vi "RUNNER_Sievert_auto_RLC-CRZPhi.vi"() -> ()   [LabVIEW 2011]
uses:
  <vilib>/Utility/error.llb/DialogType.ctl
  <vilib>/DAQmx/write.llb/DAQmx Write (Digital Bool 1Line 1Point).vi
  <vilib>/DAQmx/create/channels.llb/DAQmx Create Channel (DO-Digital Output).vi
  <vilib>/DAQmx/miscellaneous.llb/DAQmx Fill In Error Info.vi
  <vilib>/Analysis/Matrix/Numeric/Conversions/Array To Matrix - RA.vi
  <vilib>/Analysis/Matrix/Numeric/Conversions/Matrix To Array - RM.vi
  <vilib>/Analysis/NI_AALPro.lvlib
  <vilib>/Analysis/Matrix/NI_Matrix.lvlib
  <vilib>/Analysis/NI_AALBase.lvlib
panel:
  out "S#1_auto":dbl
  out "S#01":dbl
  out "output array 3":u32[](array[numeric])
  out "PCh1 2":dbl[](array[numeric])
  out "tempo carga 2":dbl[](array[numeric])
  out "path RLC_mean 2":path
  out "MEASURE R [Ohm ]":dbl
  out "tempo carga":dbl[](array[numeric])
  out "PCh1":dbl[](array[numeric])
  out "output array 2":u32[](array[numeric])
  out "MEASURE C [F ]":dbl
  out "Automatico 2":dynamicdata(graph)
  out "termopar K 2":dbl format="%.3g"
  out "termopar K":string
  out "output NTC":dbl
  out "termopar K":dbl format="%.3g"
  out "path RLC_mean":path
  out "estagio 5":i32
  out "FIM":bool=TRUE
  out "limpo":i32
  in  "N fit":i32=5
  in  "ATM wait":u32
  in  "SET":i32
  in  "time subarray":dbl[](array[numeric])
  out "P cinetica mean 2":dbl format="%0.2f"
  out "T cinetica mean 3":dbl format="%0.2f"
  out "Time cinetica":dbl format="%0.2f"
  in  "T subarray 3":dbl[](array[numeric])
  in  "P T  index 2":i32
  in  "P subarray 2":dbl[](array[numeric])
  in  "Numeric":dbl=4.0
  in  "T subarray 2":dbl[](array[numeric])
  out "T cinetica mean 2":dbl format="%0.2f"
  out "P cinetica mean":dbl format="%0.2f"
  in  "P subarray":dbl[](array[numeric])
  in  "P T  index":i32
  out "T string":string
  out "P string":string
  out "path 2_cinetica":path
  out "Polynomial Coefficients 2":dbl[](array[numeric])
  out "Polynomial Coefficients":dbl[](array[numeric])
  in  "Count SET":i32=-1
  out "Set atual":i32
  out "mean pressure":dbl format="%.4p"
  out "Set number":i32
  in  "Tab Control":T1(tab)
  out "T":bool
  out "ZPf2":bool
  out "Pf2":bool
  out "Pit":bool
  out "ZPit":bool
  out "Camara":dbl(slide) scale=0.0..59.5 scale format="%#_3g"
  in  "Save manual":bool
  in  "Open Button":bool
  out "String 2":string
  in  "ATM":bool
  in  "Câmara":bool
  in  "Vácuo":bool
  in  "Entrada Gás":bool
  in  "Manual Ctrl":bool
  in  "stop":bool
  out "P-manual":dynamicdata(graph)
  in  "Clear":bool
  out "path":path
  in  "Nota":string
  in  "Sample name":string
  in  "File name":string
  out "Linear Model Graph":dbl[][](graph)
  out "Linear Model Graph 2":dbl[][](graph)
  in  "N to fit":i32=60
  out "N":i32
  out "Vácuo":bool
  out "Atm":bool
  out "Câmara":bool
  out "String_cinetica":string
  out "Vol Ref":dbl(slide) scale=0.0..60.0 scale format="%#_4f"
  out "Entrada gás":bool
  in  "Guardar\nCinetica":bool
  out "p fit":dbl format="%#_4g"
  out "T fit":dbl format="%#_4g"
  in  "Open Button 2":bool
  out "x >= y?":bool
  in  "seconds":dbl
  out "Elapsed Time (sec)":dbl format="%.1f"
  out "bar/N":dbl format="%#_4p"
  in  "correção\n NTC":dbl
  out "mean H2 sensor (V)":dbl format="%#_4p"
  in  "correçao\n termopar":dbl
  out "Boolean 3":bool
  out "String 3":string
  out "T 2":bool
  out "ZPit 2":bool
  out "Pit 2":bool
  out "Pf2 2":bool
  out "ZPf2 2":bool
  out "Camara 2":dbl(slide) scale=0.0..40.0 scale format="%#_3g"
  out "Vácuo 2":bool
  out "Atm 2":bool
  out "Câmara 2":bool
  out "Vol Ref 3":dbl(slide) scale=0.0..100.0 scale format="%#_4f"
  out "Entrada gás 2":bool
  in  "Auto Ctrl":bool
  in  "Play Button":bool
  out "time stamp":timestamp format="%<%.2X>T"
  out "Time (sec)":dbl format="%.1f"
  in  "clear":bool
  out "Automatico":dynamicdata(graph)
  out "Linear P":T2(graph)
  out "Linear T":T2(graph)
  out "Contador":i32
  in  "STOP (bar/s)":dbl format="%#_5p"
  out "P (bar/s)":dbl format="%#_5p"
  out "bar/s":dbl format="%#_4p"
  out "P fit":dbl format="%#_4g"
  out "T fit":dbl format="%#_4g"
  out "x = y?":bool
  out "teste slope":i32
  in  "Set P auto":dbl
  in  "Step P":dbl=2.0
  in  "P_max":dbl=2.0
  in  "P_max camara":dbl=2.0
  out "Carga":bool=TRUE
  out "Descarga":bool
  out "String":string
  in  "P_min descarga":dbl
  in  "Boolean":bool
  in  "Array":dbl[](array[numeric])
  out "Boolean 2":bool
  out "Desc SET":i32
  in  "ZPf2 time":dbl=24.0
  in  "Ciclos":dbl
  out "Efetuados":dbl
  in  "patamar milliseconds to wait":u32=500
  in  "N fit patamar":i32=100
  in  "Step ZPit":dbl
  out "Read ZPit":bool
  in  "Estagio auto":i32
  out "mean H2 sensor":dbl format="%#_4p"
  in  "Ntest":i32=5
  in  "N fit 2":i32=100
  in  "Read val open":bool
  out "mean 18":dbl format="%.3p"
  out "mean 17":dbl format="%.3p"
  in  "C50L":bool
  in  "C50N":bool
  in  "C100L":bool
  in  "C100N":bool
  in  "C1KL":bool
  in  "C1KN":bool
  in  "C10KL":bool
  in  "C10KN":bool
  out "String 4":string
  in  "Combo Box":string(combo)
  in  "Refresh Button":bool
  in  "Close RLC 2":bool
  in  "RLC on/off":bool
  out "mean 16":dbl format="%.3p"
  out "mean 15":dbl format="%.3p"
  out "mean 14":dbl format="%.3p"
  out "mean 13":dbl format="%.3p"
  out "mean 12":dbl format="%.3p"
  out "mean 11":dbl format="%.3p"
  out "mean 10":dbl format="%.3p"
  out "mean 9":dbl format="%.3p"
  out "mean 8":dbl format="%.3p"
  out "mean 7":dbl format="%.3p"
  out "mean 6":dbl format="%.3p"
  out "mean 5":dbl format="%.3p"
  out "mean 4":dbl format="%.3p"
  out "mean 3":dbl format="%.3p"
  out "mean 2":dbl format="%.3p"
  out "mean":dbl format="%.3p"
  out "SET 2":dbl
  out "C-50-L":bool
  out "MEASURE B":dbl
  out "MEASURE A":dbl
  out "C-50-N":bool
  out "MEASURE B 2":dbl
  out "MEASURE A 2":dbl
  out "C-100-L":bool
  out "MEASURE B 3":dbl
  out "MEASURE A 3":dbl
  out "C-100-N":bool
  out "MEASURE B 4":dbl
  out "MEASURE A 4":dbl
  out "C-1K-L":bool
  out "MEASURE B 5":dbl
  out "MEASURE A 5":dbl
  out "C-1K-N":bool
  out "MEASURE B 6":dbl
  out "MEASURE A 6":dbl
  out "C-10K-L":bool
  out "MEASURE B 7":dbl
  out "MEASURE A 7":dbl
  out "C-10K-N":bool
  out "MEASURE B 8":dbl
  out "MEASURE A 8":dbl
  out "Z-50-L":bool
  out "MEASURE B 9":dbl
  out "MEASURE A 9":dbl
  out "Z-50-N":bool
  out "MEASURE B 10":dbl
  out "MEASURE A 10":dbl
  out "Z-100-L":bool
  out "MEASURE B 11":dbl
  out "MEASURE A 11":dbl
  out "Z-100-N":bool
  out "MEASURE B 12":dbl
  out "MEASURE A 12":dbl
  out "Z-1K-L":bool
  out "MEASURE B 13":dbl
  out "MEASURE A 13":dbl
  out "Z-1K-N":bool
  out "MEASURE B 14":dbl
  out "MEASURE A 14":dbl
  out "Z-10K-L":bool
  out "MEASURE B 15":dbl
  out "MEASURE A 15":dbl
  out "Z-10K-N":bool
  out "MEASURE B 16":dbl
  out "MEASURE A 16":dbl
  out "RLC300 - digimess":string
  in  "Time RLC":u32=5000
  in  "Ligar RLC":bool
  out "path RLC_completo":path
  out "Waveform Chart P 2":dbl[][](graph)
  out "Waveform Chart":dynamicdata(graph)
  in  "graph RLC":bool
  in  "Refresh Button 2":bool
  in  "Z50L":bool
  in  "Z50N":bool
  in  "Z100L":bool
  in  "Z100N":bool
  in  "Z1KL":bool
  in  "Z1KN":bool
  in  "Z10KL":bool
  in  "Z10KN":bool
  out "T(º) FIT":dbl
  out "Waveform Chart 2":dynamicdata(graph)
  out "XY Graph 2":cluster{"Value":dbl[], "Value":dbl[]}[](graph)
  in  "t-sivert01(s)":dbl
  out "dP/dt (bar/s)":dbl format="%#_5p"
  in  "Save - Sievert 01":bool
  in  "File name 2":string
  in  "Nota 01":string
  in  "Sample name 2":string
  in  "Save S#1":bool
  out "path 2":path
  out "Boolean 4":bool
  out "P(bar) FIT":dbl
  in  "ON/OFF":bool
  in  "Refresh Button 3":bool
  # "P vol ref"
  # "P Câmara"
  # "P vol ref"
  # "P Câmara"
  # "C ( F )"
  # "R ( Ohm )"
  # "Z ( Ohm )"
  # "Phase ( deg)"
types:
  T1 = enum32{"Manual", "Automatico", "RLC - CDH2", "Sievert 01"}
  T2 = cluster{"Real 2D Array":dbl[], "Best Linear Fit":dbl[]}[]
  T3 = enum16{"open", "replace", "create", "open or create", "replace or create", "replace or create with confirmation"}
  T4 = typedef "DialogType.ctl" = u16
  T5 = cluster{"Value":dbl[], "Best Polynomial Fit":dbl[]}
  T6 = cluster{"Value":dbl[], "Best Polynomial Fit":dbl[]}[]
  T7 = typedef "NI_Matrix.lvlib/RealMatrix.ctl" = dbl[][]
  T8 = cluster{"Real 2D Array":dbl[], "Real 2D Array":dbl[]}
  T9 = cluster{"Real 2D Array":dbl[], "Best Linear Fit":dbl[]}
  T10 = cluster{"Real 2D Array":dbl[], "Best Polynomial Fit":dbl[]}
  T11 = cluster{"Real 2D Array":dbl[], "Best Polynomial Fit":dbl[]}[]
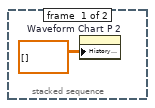
[diagram p7: hidden frame]
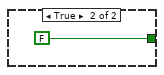
[diagram p12: hidden frame]
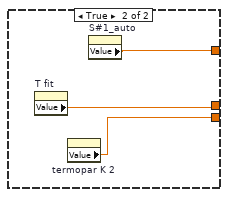
[diagram p15: hidden frame]
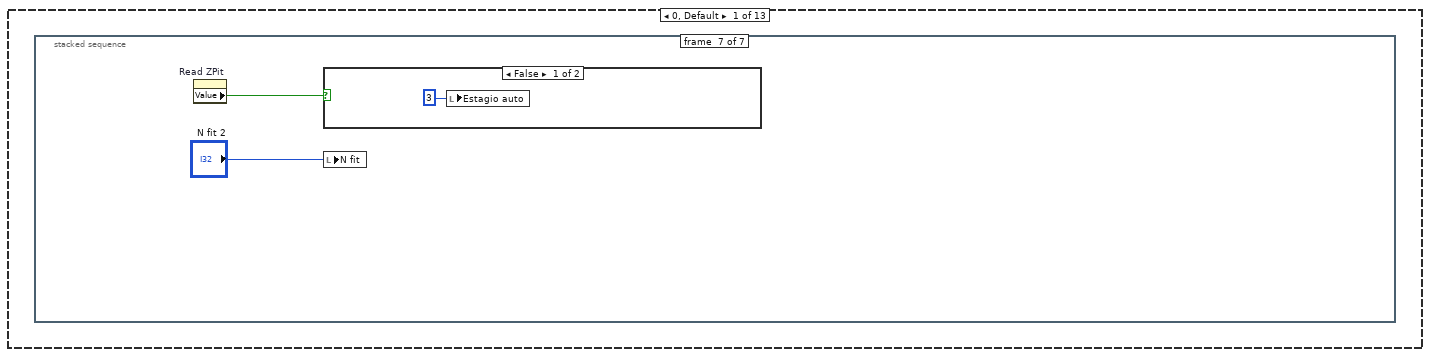
[diagram p20: hidden frame]
diagram:
  w2 = TRUE ("C1KN")
  (unwired) dbl[] [0.5, 1.0, 2.0, 3.0, 4.0, 5.0, 6.0, 7.0, 8.0, 9.0, 10.0, 11.0, 12.0, 13.0, 14.0, 15.0, 16.0, 17.0, 18.0, 19.0, 20.0, 30.0, 40.0, 50.0, 60.0, 70.0] ("Array")
  n1 = local write "N to fit"(5 ("Numeric")) -> ()
  n2 = local write "Step ZPit"(5.0 ("Step ZPit")) -> ()
  n3 = local write "Time RLC"(u32 5 ("Time RLC")) -> ()
  n4 = local write "Ciclos"(0.0 ("Ciclos")) -> ()
  n5 = local write "Desc SET"(0 ("Desc SET")) -> ()
  n6 = local write "Efetuados"(0.0 ("Efetuados")) -> ()
  n7 = local write "estagio 5"(0 ("estagio 5")) -> ()
  n8 = local write "teste slope"(0 ("teste slope")) -> ()
  n9 = local write "SET"(0 ("SET auto")) -> ()
  n10 = local write "limpo"(0 ("limpo")) -> ()
  n11 = local write "N fit"(5 ("N fit")) -> ()
  n12 = local write "ATM wait"(u32 4 ("ATM wait")) -> ()
  n13 = local write "Estagio auto"(0 ("Estagio auto")) -> ()
  n14 = local write "P T  index"(0 ("index")) -> ()
  n15 = local write "seconds"(2.0 ("seconds")) -> ()
  n16 = local write "C1KN"(w2) -> ()
  n17 = local write "Z1KN"(w2) -> ()
  n18 = local write "Read ZPit"(TRUE ("Read ZPit")) -> ()
  n19 = local write "Descarga"(FALSE ("Descarga")) -> ()
  n20 = local write "Carga"(TRUE ("Carga")) -> ()
  n21 = local write "FIM"(FALSE ("FIM")) -> ()
  n22 = local write "t-sivert01(s)"(10.0 ("t-sivert01(s)")) -> ()
  n23 = local write "P_max"(50.0 ("P_max")) -> ()
  n24 = local write "P_max camara"(25.0 ("P_max camara")) -> ()
  n25 = local write "correção\n NTC"(0.5 ("correção NTC")) -> ()
  n26 = local write "Set P auto"(0.5 ("Set P auto")) -> ()
  n27 = local write "P_min descarga"(0.025 ("P_min descarga")) -> ()
  n28 = local write "Array"(dbl[] [0.5, 1.0, 2.0, 3.0, 4.0, 4.0, 4.0, 4.0, 4.0, 4.0, 4.0, 5.0, 5.0, 5.0, 7.0, 10.0, 15.0, 20.0, 25.0, 25.0, 25.0, 30.0, 40.0, 50.0, 60.0, 70.0] ("Array")) -> ()
  n29 = local write "P subarray"(dbl[] [0.0, 1.0] ("subarray")) -> ()
  n30 = local write "T subarray 2"(dbl[] [0.0, 1.0] ("subarray")) -> ()
  n31 = local write "Combo Box"("rlc_read_cCN.py" ("Combo Box")) -> ()
  n32 = while {
    tunnel: path "C:/H2_Painel/painel_auto/RLC_CDH" ("Path") -> [w40]
    stop <- w52 stop-if-true
    n33 = property on="FIM" class="Bool (strict)"() -> ("Value"=w50:bool)  [unwired: 2 in, 2 out]
    n34 = property on="path" class="Path"() -> ("Value"=w47:path)  [unwired: 2 in, 2 out]
    n35 = case shown="True" "Ligar RLC" {
      tunnel: w40 -> [_ w231]
      frame False {
      }
      frame True {
        n36 = call "RLC_open.vi"("Path"=w231) -> ("String 2"=w232:string)  [unwired: 9 in, 1 out]
        n37 = local write "RLC300 - digimess"(w232) -> ()
      }
    }
    n38 = case shown="True" "RLC on/off" {
      tunnel: w40 -> [_ _]
      frame False {
      }
      frame True {
        n39 = call "RLC READ DINAMICO.vi"("Boolean"="graph RLC") -> ("MEASURE R [Ohm ]"=w66:dbl, "MEASURE C [F ]"=w65:dbl)  [unwired: 9 in]
        "MEASURE C [F ]" <- w65
        "MEASURE R [Ohm ]" <- w66
        n40 = Merge Signals(w65, w66) -> (→"Waveform Chart":dynamicdata)
        "String 4" <- "Combo Box"
      }
    }
    n41 = case shown="True" "Manual Ctrl" {
      tunnel: w40 -> [_ w1859]
      tunnel: "RLC on/off" -> [_ w1858]
      tunnel: [FALSE w1861] -> w42
      frame False {
      }
      frame True {
        w1873 = 0 ("polynomial order")
        n42 = case shown="True" "Save manual" {
          selector: "Save manual" -> [_ w2475]
          frame False {
          }
          frame True {
            n43 = feedback #1() -> (w2471:dbl)  [unwired: 1 in]
            n44 = Equal To 0?(x=w2471) -> (x = 0?=w2477:bool)
            n45 = stacked-sequence {
              tunnel: w2477 -> [_ w2493 _]
              tunnel: [_ w2492 _] -> w2473
              frame #0 {
                w2486 = i16 3 ("precision (6)")
                n46 = property on="T fit" class="DigNum (strict)"() -> ("Value"=w2488:dbl)  [unwired: 2 in, 2 out]
                n47 = property on="p fit" class="DigNum (strict)"() -> ("Value"=w2489:dbl)  [unwired: 2 in, 2 out]
                n48 = property on="termopar K" class="DigNum (strict)"() -> ("Value"=w2487:dbl)  [unwired: 2 in, 2 out]
                n49 = Number To Fractional String(number=w2488, precision (6)=w2486) -> (F-format string=→"T string":string)  [unwired: 2 in]
                n50 = Number To Fractional String(number=w2489, precision (6)=w2486) -> (F-format string=→"P string":string)  [unwired: 2 in]
                n51 = Number To Fractional String(number=w2487, precision (6)=w2486) -> (F-format string=→"termopar K":string)  [unwired: 2 in]
              }
              frame #1 {
                n52 = case shown="True" w2493 {
                  tunnel: [TRUE ("y") FALSE ("y")] -> w2492
                  frame False {
                    n53 = property on="path" class="Path"() -> ("Value"=w2497:path)  [unwired: 2 in, 2 out]
                    n54 = property on="P string" class="Str"() -> ("Value"=w2496:string)  [unwired: 2 in, 2 out]
                    n55 = Concatenate Strings(w2496, "\t") -> (w2494:string)
                    n56 = Open/Create/Replace File(file path (use dialog)=w2497, operation (0:open)=T3."open") -> (refnum out=w2501:refnum<file>, error out=w2500:errorcluster)  [unwired: 2 in, 3 out]
                    n57 = Set File Position(refnum=w2501, from (0:start)=enum16{"start", "end", "current"}."end", error in=w2500) -> (refnum out=w2503:refnum<file>, error out=w2504:errorcluster)  [unwired: 1 in]
                    n58 = Write to Text File(file (use dialog)=w2503, text=w2494, error in=w2504) -> (refnum out=w2499:refnum<file>, error out=w2498:errorcluster)  [unwired: 2 out]
                    n59 = Close File(refnum=w2499, error in=w2498) -> (error out=w2506:errorcluster)  [unwired: 1 out]
                    n60 = call <vilib>:"Simple Error Handler.vi"("error in (no error)"=w2506) -> ()  [unwired: 1 in, 8 out]
                  }
                  frame True {
                    w2509 = "\t"
                    n61 = property on="path" class="Path"() -> ("Value"=w2516:path)  [unwired: 2 in, 2 out]
                    n62 = property on="Count SET" class="DigNum (strict)"() -> ("Value"=w2512:i32)  [unwired: 2 in, 2 out]
                    n63 = Open/Create/Replace File(file path (use dialog)=w2516, operation (0:open)=T3."open") -> (refnum out=w2515:refnum<file>, error out=w2514:errorcluster)  [unwired: 2 in, 3 out]
                    n64 = Increment(x=w2512) -> (x+1=w2513:i32)
                    "Set atual" <- w2513
                    n65 = Set File Position(refnum=w2515, from (0:start)=enum16{"start", "end", "current"}."end", error in=w2514) -> (refnum out=w2524:refnum<file>, error out=w2525:errorcluster)  [unwired: 1 in]
                    n66 = Number To Decimal String(number=w2513) -> (decimal integer string=w2517:string)  [unwired: 1 in]
                    n67 = property on="termopar K" class="Str"() -> ("Value"=w2508:string)  [unwired: 2 in, 2 out]
                    n68 = property on="T string" class="Str"() -> ("Value"=w2510:string)  [unwired: 2 in, 2 out]
                    n69 = Concatenate Strings(w2510, w2509, w2508, "\r\n", w2517, w2509) -> (w2519:string)
                    n70 = Write to Text File(file (use dialog)=w2524, text=w2519, error in=w2525) -> (refnum out=w2522:refnum<file>, error out=w2521:errorcluster)  [unwired: 2 out]
                    n71 = Close File(refnum=w2522, error in=w2521) -> (error out=w2527:errorcluster)  [unwired: 1 out]
                    n72 = call <vilib>:"Simple Error Handler.vi"("error in (no error)"=w2527) -> ()  [unwired: 1 in, 8 out]
                    "T" <- TRUE ("T")
                  }
                }
              }
              frame #2 {
                n73 = property on="path" class="Path"() -> ("Value"=w2529:path)  [unwired: 2 in, 2 out]
                n74 = property on="Set atual" class="DigNum (strict)"() -> ("Value"=w2528:i32)  [unwired: 2 in, 2 out]
                n75 = local write "Count SET"(w2528) -> ()
                n76 = Read from Text File(file (use dialog)=w2529, count=-1 ("Count  3")) -> (refnum out=w2531:refnum<file>, text=w2530:string, error out=w2532:errorcluster)  [unwired: 2 in, 1 out]
                n77 = property on="String 2" class="Str"("Value"=w2530) -> ()  [unwired: 2 in, 2 out]
                n78 = Close File(refnum=w2531, error in=w2532) -> (error out=w2534:errorcluster)  [unwired: 1 out]
                n79 = call <vilib>:"Simple Error Handler.vi"("error in (no error)"=w2534) -> ()  [unwired: 1 in, 8 out]
              }
            }
            n80 = Implies(1:w2473, 2:w2475) -> (0:w2474:bool)
            n81 = Select(t=w2471, s=w2474, f=5.0 ("t")) -> (s? t:f=w2472:dbl)
            n82 = case shown="1" w2472 {
              frame 0, Default {
              }
              frame 1 {
                "ZPf2" <- TRUE ("ZPf2")
              }
              frame 2 {
                "Pf2" <- TRUE ("Pf2")
              }
              frame 3 {
                "Pit" <- TRUE ("Pit")
              }
              frame 4 {
                n83 = local write "T"(FALSE ("T")) -> ()
                "ZPit" <- TRUE ("ZPit")
              }
              frame 5 {
                w2484 = FALSE
                n84 = local write "Pit"(w2484) -> ()
                n85 = local write "ZPf2"(w2484) -> ()
                n86 = local write "ZPit"(w2484) -> ()
                n87 = local write "Pf2"(w2484) -> ()
              }
            }
            n88 = Decrement(x=w2472) -> (x-1=w2478:dbl)
            n89 = feedback-in #1(w2478) -> ()
          }
        }
        n90 = case shown="True" w1858 {
          tunnel: [FALSE ("Save manual") w2470] -> w1860
          tunnel: "Save manual" -> [_ w2470]
          frame False {
          }
          frame True {
          }
        }
        n91 = case shown="True" w1858 {
          tunnel: [FALSE w1878] -> w1861
          tunnel: w1860 -> [_ w1877]
          tunnel: w1859 -> [_ w1876]
          frame False {
          }
          frame True {
            n92 = flat-sequence {
              tunnel: w1876 -> [w1899]
              tunnel: w1877 -> [w1900]
              tunnel: [w1900] -> w1897
              tunnel: [w1899] -> w1896
              tunnel: [w1907] -> w1895
              tunnel: [w1908] -> w1894
              tunnel: [w1909] -> w1893
              tunnel: [w1910] -> w1892
              tunnel: [w1911] -> w1891
              tunnel: [w1912] -> w1890
              tunnel: [w1913] -> w1889
              tunnel: [w1915] -> w1888
              tunnel: [w1916] -> w1887
              tunnel: [w1917] -> w1886
              tunnel: [w1918] -> w1885
              tunnel: [w1919] -> w1884
              tunnel: [w1914] -> w1883
              tunnel: [w1906] -> w1882
              tunnel: [w1905] -> w1881
              tunnel: [w1904] -> w1880
              tunnel: [w1903] -> w1879
              tunnel: w1897 -> [w1902]
              tunnel: w1896 -> [w1901]
              tunnel: w1895 -> [w2417]
              tunnel: w1894 -> [w2416]
              tunnel: w1893 -> [w2415]
              tunnel: w1892 -> [w2414]
              tunnel: w1891 -> [w2413]
              tunnel: w1890 -> [w2412]
              tunnel: w1889 -> [w2411]
              tunnel: w1888 -> [w2410]
              tunnel: w1887 -> [w2409]
              tunnel: w1886 -> [w2408]
              tunnel: w1885 -> [w2407]
              tunnel: w1884 -> [w2406]
              tunnel: w1883 -> [w2405]
              tunnel: w1882 -> [w2418]
              tunnel: w1881 -> [w2419]
              tunnel: w1880 -> [w2420]
              tunnel: [w2403] -> w1878
              tunnel: w1879 -> [w2403]
              tunnel: [TRUE] -> w1875
              frame #0 {
                n93 = local write "graph RLC"(FALSE) -> ()
              }
              frame #1 {
                n94 = case shown="True" w1902 {
                  tunnel: [_ w1954] -> w1903
                  tunnel: w1901 -> [_ w1936]
                  tunnel: [_ w1935] -> w1904
                  tunnel: [_ w1934] -> w1905
                  tunnel: [_ w1933] -> w1906
                  tunnel: [_ w1932] -> w1907
                  tunnel: [_ w1931] -> w1908
                  tunnel: [_ w1930] -> w1909
                  tunnel: [_ w1929] -> w1910
                  tunnel: [_ w1928] -> w1911
                  tunnel: [_ w1927] -> w1912
                  tunnel: [_ w1926] -> w1913
                  tunnel: [_ w1925] -> w1914
                  tunnel: [_ w1924] -> w1915
                  tunnel: [_ w1923] -> w1916
                  tunnel: [_ w1922] -> w1917
                  tunnel: [_ w1921] -> w1918
                  tunnel: [_ w1920] -> w1919
                  frame False {
                  }
                  frame True {
                    n95 = for {
                      N: 5 -> [_]
                      tunnel: TRUE -> [w1977]
                      tunnel: FALSE -> [w1976]
                      tunnel: [w1975] -> w1954
                      tunnel: [w1974] -> w1952 mode=indexing
                      tunnel: [w1973] -> w1951 mode=indexing
                      tunnel: [w1972] -> w1950 mode=indexing
                      tunnel: [w1971] -> w1949 mode=indexing
                      tunnel: [w1970] -> w1948 mode=indexing
                      tunnel: [w1969] -> w1947 mode=indexing
                      tunnel: [w1968] -> w1946 mode=indexing
                      tunnel: [w1967] -> w1945 mode=indexing
                      tunnel: [w1966] -> w1944 mode=indexing
                      tunnel: [w1965] -> w1943 mode=indexing
                      tunnel: [w1964] -> w1942 mode=indexing
                      tunnel: [w1963] -> w1941 mode=indexing
                      tunnel: [w1962] -> w1940 mode=indexing
                      tunnel: [w1961] -> w1939 mode=indexing
                      tunnel: [w1960] -> w1938 mode=indexing
                      tunnel: [w1959] -> w1937 mode=indexing
                      tunnel: w1936 -> [w1958]
                      n96 = property on="path RLC_completo" class="Path"() -> ("Value"=w1957:path)  [unwired: 2 in, 2 out]
                      n97 = stacked-sequence {
                        tunnel: w1977 -> [_ w2002 w2027 w2052 w2077 w2102 w2127 w2152 w2175 w2200 w2227 w2250 w2277 w2302 w2327 w2350 w2377 _]
                        tunnel: w1976 -> [w1978 _ _ _ _ _ _ _ _ _ _ _ _ _ _ _ _ w2401]
                        tunnel: [_ _ _ _ _ _ _ _ _ _ _ _ _ _ _ _ _ TRUE] -> w1975
                        tunnel: [_ w2001 _ _ _ _ _ _ _ _ _ _ _ _ _ _ _ _] -> w1974
                        tunnel: [_ _ w2026 _ _ _ _ _ _ _ _ _ _ _ _ _ _ _] -> w1973
                        tunnel: [_ _ _ w2051 _ _ _ _ _ _ _ _ _ _ _ _ _ _] -> w1972
                        tunnel: [_ _ _ _ w2076 _ _ _ _ _ _ _ _ _ _ _ _ _] -> w1971
                        tunnel: [_ _ _ _ _ w2101 _ _ _ _ _ _ _ _ _ _ _ _] -> w1970
                        tunnel: [_ _ _ _ _ _ w2126 _ _ _ _ _ _ _ _ _ _ _] -> w1969
                        tunnel: [_ _ _ _ _ _ _ w2151 _ _ _ _ _ _ _ _ _ _] -> w1968
                        tunnel: [_ _ _ _ _ _ _ _ w2177 _ _ _ _ _ _ _ _ _] -> w1967
                        tunnel: [_ _ _ _ _ _ _ _ _ w2202 _ _ _ _ _ _ _ _] -> w1966
                        tunnel: [_ _ _ _ _ _ _ _ _ _ w2226 _ _ _ _ _ _ _] -> w1965
                        tunnel: [_ _ _ _ _ _ _ _ _ _ _ w2252 _ _ _ _ _ _] -> w1964
                        tunnel: [_ _ _ _ _ _ _ _ _ _ _ _ w2276 _ _ _ _ _] -> w1963
                        tunnel: [_ _ _ _ _ _ _ _ _ _ _ _ _ w2301 _ _ _ _] -> w1962
                        tunnel: [_ _ _ _ _ _ _ _ _ _ _ _ _ _ w2326 _ _ _] -> w1961
                        tunnel: [_ _ _ _ _ _ _ _ _ _ _ _ _ _ _ w2352 _ _] -> w1960
                        tunnel: [_ _ _ _ _ _ _ _ _ _ _ _ _ _ _ _ w2376 _] -> w1959
                        tunnel: w1958 -> [_ w2004 w2030 w2054 w2079 w2104 w2129 w2154 w2179 w2204 w2229 w2254 w2279 w2304 w2329 w2354 w2379 _]
                        tunnel: w1957 -> [w1980 w2003 w2029 w2053 w2078 w2103 w2128 w2153 w2178 w2203 w2228 w2253 w2278 w2303 w2328 w2353 w2378 _]
                        frame #0 {
                          w1981 = "\t"
                          n98 = local write "C-50-L"(w1978) -> ()
                          n99 = local write "C-50-N"(w1978) -> ()
                          n100 = local write "Z-50-L"(w1978) -> ()
                          n101 = local write "Z-50-N"(w1978) -> ()
                          n102 = local write "C-1K-L"(w1978) -> ()
                          n103 = local write "C-1K-N"(w1978) -> ()
                          n104 = local write "Z-1K-N"(w1978) -> ()
                          n105 = local write "Z-1K-L"(w1978) -> ()
                          n106 = local write "Z-100-L"(w1978) -> ()
                          n107 = local write "C-10K-L"(w1978) -> ()
                          n108 = local write "C-100-N"(w1978) -> ()
                          n109 = local write "C-10K-N"(w1978) -> ()
                          n110 = local write "Z-10K-N"(w1978) -> ()
                          n111 = local write "Z-10K-L"(w1978) -> ()
                          n112 = local write "Z-100-N"(w1978) -> ()
                          n113 = local write "C-100-L"(w1978) -> ()
                          n114 = Open/Create/Replace File(file path (use dialog)=w1980, operation (0:open)=T3."open") -> (refnum out=w1994:refnum<file>, error out=w1993:errorcluster)  [unwired: 2 in, 3 out]
                          n115 = Get Date/Time String(date format (0)=enum16{"short", "long", "abbreviated"}."short", want seconds? (F)=TRUE) -> (date string=w1986:string, time string=w1985:string)  [unwired: 1 in]
                          n116 = feedback #2() -> (w1979:dbl)  [unwired: 1 in]
                          n117 = local write "SET 2"(w1979) -> ()
                          n118 = Set File Position(refnum=w1994, from (0:start)=enum16{"start", "end", "current"}."end", error in=w1993) -> (refnum out=w1996:refnum<file>, error out=w1997:errorcluster)  [unwired: 1 in]
                          n119 = Number To Fractional String(number=w1979, precision (6)=i16 2) -> (F-format string=w1984:string)  [unwired: 2 in]
                          n120 = Add(x=w1979, y=0.2) -> (x+y=w1990:dbl)
                          n121 = feedback-in #2(w1990) -> ()
                          n122 = Concatenate Strings(w1984, w1981, w1986, w1981, w1985, w1981) -> (w1983:string)
                          n123 = Write to Text File(file (use dialog)=w1996, text=w1983, error in=w1997) -> (refnum out=w1992:refnum<file>, error out=w1991:errorcluster)  [unwired: 1 in, 1 out]
                          n124 = Close File(refnum=w1992, error in=w1991) -> (error out=w1999:errorcluster)  [unwired: 1 out]
                          n125 = call <vilib>:"Simple Error Handler.vi"("error in (no error)"=w1999) -> ()  [unwired: 1 in, 8 out]
                        }
                        frame #1 {
                          w2005 = "\t"
                          w2022 = i16 4 ("width (-)")
                          n126 = local write "C-50-L"(w2002) -> ()
                          n127 = Wait (ms)(milliseconds to wait=u32 5000) -> ()  [unwired: 1 out]
                          n128 = Open/Create/Replace File(file path (use dialog)=w2003, operation (0:open)=T3."open") -> (refnum out=w2014:refnum<file>, error out=w2013:errorcluster)  [unwired: 2 in, 3 out]
                          n129 = Set File Position(refnum=w2014, from (0:start)=enum16{"start", "end", "current"}."end", error in=w2013) -> (refnum out=w2016:refnum<file>, error out=w2017:errorcluster)  [unwired: 1 in]
                          n130 = call "RLC_read.vi"("Path"=w2004, "String"="cmd /c rlc_read_cAL.py") -> ("MEASURE A"=w2001:dbl, "MEASURE V [V]"=w2021:dbl, "MEASURE B"=w2000:dbl, "MEASURE I [A]"=w2020:dbl)  [unwired: 2 out]
                          n131 = Number To Engineering String(2:w2022, 4:w2020) -> (0:w2006:string)  [unwired: 2 in]
                          n132 = local write "MEASURE A"(w2001) -> ()
                          n133 = local write "MEASURE B"(w2000) -> ()
                          n134 = Number To Engineering String(2:w2022, 4:w2021) -> (0:w2007:string)  [unwired: 2 in]
                          n135 = Number To Engineering String(2:w2022, 4:w2001) -> (0:w2009:string)  [unwired: 2 in]
                          n136 = Number To Engineering String(2:w2022, 4:w2000) -> (0:w2008:string)  [unwired: 2 in]
                          n137 = Concatenate Strings(w2009, w2005, w2008, w2005, w2007, w2005, w2006, w2005) -> (w2010:string)
                          n138 = Write to Text File(file (use dialog)=w2016, text=w2010, error in=w2017) -> (refnum out=w2012:refnum<file>, error out=w2011:errorcluster)  [unwired: 1 in, 1 out]
                          n139 = Close File(refnum=w2012, error in=w2011) -> (error out=w2019:errorcluster)  [unwired: 1 out]
                          n140 = call <vilib>:"Simple Error Handler.vi"("error in (no error)"=w2019) -> ()  [unwired: 1 in, 8 out]
                        }
                        frame #2 {
                          w2033 = "\t"
                          w2047 = i16 4 ("width (-)")
                          n141 = local write "C-50-N"(w2027) -> ()
                          n142 = Wait (ms)(milliseconds to wait=u32 5000) -> ()  [unwired: 1 out]
                          n143 = Open/Create/Replace File(file path (use dialog)=w2029, operation (0:open)=T3."open") -> (refnum out=w2041:refnum<file>, error out=w2040:errorcluster)  [unwired: 2 in, 3 out]
                          n144 = Set File Position(refnum=w2041, from (0:start)=enum16{"start", "end", "current"}."end", error in=w2040) -> (refnum out=w2043:refnum<file>, error out=w2044:errorcluster)  [unwired: 1 in]
                          n145 = call "RLC_read.vi"("Path"=w2030, "String"="cmd /c rlc_read_cAN.py") -> ("MEASURE A"=w2026:dbl, "MEASURE V [V]"=w2032:dbl, "MEASURE B"=w2025:dbl, "MEASURE I [A]"=w2031:dbl)  [unwired: 2 out]
                          n146 = Number To Engineering String(2:w2047, 4:w2031) -> (0:w2034:string)  [unwired: 2 in]
                          n147 = local write "MEASURE A 2"(w2026) -> ()
                          n148 = local write "MEASURE B 2"(w2025) -> ()
                          n149 = Number To Engineering String(2:w2047, 4:w2032) -> (0:w2035:string)  [unwired: 2 in]
                          n150 = Number To Engineering String(2:w2047, 4:w2026) -> (0:w2037:string)  [unwired: 2 in]
                          n151 = Number To Engineering String(2:w2047, 4:w2025) -> (0:w2036:string)  [unwired: 2 in]
                          n152 = Concatenate Strings(w2037, w2033, w2036, w2033, w2035, w2033, w2034, w2033) -> (w2028:string)
                          n153 = Write to Text File(file (use dialog)=w2043, text=w2028, error in=w2044) -> (refnum out=w2039:refnum<file>, error out=w2038:errorcluster)  [unwired: 1 in, 1 out]
                          n154 = Close File(refnum=w2039, error in=w2038) -> (error out=w2046:errorcluster)  [unwired: 1 out]
                          n155 = call <vilib>:"Simple Error Handler.vi"("error in (no error)"=w2046) -> ()  [unwired: 1 in, 8 out]
                        }
                        frame #3 {
                          w2057 = "\t"
                          w2072 = i16 4 ("width (-)")
                          n156 = Wait (ms)(milliseconds to wait=u32 5000) -> ()  [unwired: 1 out]
                          n157 = local write "C-100-L"(w2052) -> ()
                          n158 = Open/Create/Replace File(file path (use dialog)=w2053, operation (0:open)=T3."open") -> (refnum out=w2066:refnum<file>, error out=w2065:errorcluster)  [unwired: 2 in, 3 out]
                          n159 = Set File Position(refnum=w2066, from (0:start)=enum16{"start", "end", "current"}."end", error in=w2065) -> (refnum out=w2068:refnum<file>, error out=w2069:errorcluster)  [unwired: 1 in]
                          n160 = call "RLC_read.vi"("Path"=w2054, "String"="cmd /c rlc_read_cBL.py") -> ("MEASURE A"=w2051:dbl, "MEASURE V [V]"=w2056:dbl, "MEASURE B"=w2050:dbl, "MEASURE I [A]"=w2055:dbl)  [unwired: 2 out]
                          n161 = Number To Engineering String(2:w2072, 4:w2055) -> (0:w2058:string)  [unwired: 2 in]
                          n162 = local write "MEASURE A 3"(w2051) -> ()
                          n163 = local write "MEASURE B 3"(w2050) -> ()
                          n164 = Number To Engineering String(2:w2072, 4:w2056) -> (0:w2059:string)  [unwired: 2 in]
                          n165 = Number To Engineering String(2:w2072, 4:w2051) -> (0:w2061:string)  [unwired: 2 in]
                          n166 = Number To Engineering String(2:w2072, 4:w2050) -> (0:w2060:string)  [unwired: 2 in]
                          n167 = Concatenate Strings(w2061, w2057, w2060, w2057, w2059, w2057, w2058, w2057) -> (w2062:string)
                          n168 = Write to Text File(file (use dialog)=w2068, text=w2062, error in=w2069) -> (refnum out=w2064:refnum<file>, error out=w2063:errorcluster)  [unwired: 1 in, 1 out]
                          n169 = Close File(refnum=w2064, error in=w2063) -> (error out=w2071:errorcluster)  [unwired: 1 out]
                          n170 = call <vilib>:"Simple Error Handler.vi"("error in (no error)"=w2071) -> ()  [unwired: 1 in, 8 out]
                        }
                        frame #4 {
                          w2082 = "\t"
                          w2097 = i16 4 ("width (-)")
                          n171 = Wait (ms)(milliseconds to wait=u32 5000) -> ()  [unwired: 1 out]
                          n172 = local write "C-100-N"(w2077) -> ()
                          n173 = Open/Create/Replace File(file path (use dialog)=w2078, operation (0:open)=T3."open") -> (refnum out=w2091:refnum<file>, error out=w2090:errorcluster)  [unwired: 2 in, 3 out]
                          n174 = Set File Position(refnum=w2091, from (0:start)=enum16{"start", "end", "current"}."end", error in=w2090) -> (refnum out=w2093:refnum<file>, error out=w2094:errorcluster)  [unwired: 1 in]
                          n175 = call "RLC_read.vi"("Path"=w2079, "String"="cmd /c rlc_read_cBN.py") -> ("MEASURE A"=w2076:dbl, "MEASURE V [V]"=w2081:dbl, "MEASURE B"=w2075:dbl, "MEASURE I [A]"=w2080:dbl)  [unwired: 2 out]
                          n176 = Number To Engineering String(2:w2097, 4:w2080) -> (0:w2083:string)  [unwired: 2 in]
                          n177 = local write "MEASURE A 4"(w2076) -> ()
                          n178 = local write "MEASURE B 4"(w2075) -> ()
                          n179 = Number To Engineering String(2:w2097, 4:w2081) -> (0:w2084:string)  [unwired: 2 in]
                          n180 = Number To Engineering String(2:w2097, 4:w2076) -> (0:w2086:string)  [unwired: 2 in]
                          n181 = Number To Engineering String(2:w2097, 4:w2075) -> (0:w2085:string)  [unwired: 2 in]
                          n182 = Concatenate Strings(w2086, w2082, w2085, w2082, w2084, w2082, w2083, w2082) -> (w2087:string)
                          n183 = Write to Text File(file (use dialog)=w2093, text=w2087, error in=w2094) -> (refnum out=w2089:refnum<file>, error out=w2088:errorcluster)  [unwired: 1 in, 1 out]
                          n184 = Close File(refnum=w2089, error in=w2088) -> (error out=w2096:errorcluster)  [unwired: 1 out]
                          n185 = call <vilib>:"Simple Error Handler.vi"("error in (no error)"=w2096) -> ()  [unwired: 1 in, 8 out]
                        }
                        frame #5 {
                          w2122 = "\t"
                          w2107 = i16 4 ("width (-)")
                          n186 = local write "C-1K-L"(w2102) -> ()
                          n187 = Wait (ms)(milliseconds to wait=u32 5000) -> ()  [unwired: 1 out]
                          n188 = Open/Create/Replace File(file path (use dialog)=w2103, operation (0:open)=T3."open") -> (refnum out=w2113:refnum<file>, error out=w2114:errorcluster)  [unwired: 2 in, 3 out]
                          n189 = Set File Position(refnum=w2113, from (0:start)=enum16{"start", "end", "current"}."end", error in=w2114) -> (refnum out=w2111:refnum<file>, error out=w2110:errorcluster)  [unwired: 1 in]
                          n190 = call "RLC_read.vi"("Path"=w2104, "String"="cmd /c rlc_read_cCL.py") -> ("MEASURE A"=w2101:dbl, "MEASURE V [V]"=w2106:dbl, "MEASURE B"=w2100:dbl, "MEASURE I [A]"=w2105:dbl)  [unwired: 2 out]
                          n191 = Number To Engineering String(2:w2107, 4:w2105) -> (0:w2121:string)  [unwired: 2 in]
                          n192 = local write "MEASURE A 5"(w2101) -> ()
                          n193 = local write "MEASURE B 5"(w2100) -> ()
                          n194 = Number To Engineering String(2:w2107, 4:w2106) -> (0:w2120:string)  [unwired: 2 in]
                          n195 = Number To Engineering String(2:w2107, 4:w2101) -> (0:w2118:string)  [unwired: 2 in]
                          n196 = Number To Engineering String(2:w2107, 4:w2100) -> (0:w2119:string)  [unwired: 2 in]
                          n197 = Concatenate Strings(w2118, w2122, w2119, w2122, w2120, w2122, w2121, w2122) -> (w2117:string)
                          n198 = Write to Text File(file (use dialog)=w2111, text=w2117, error in=w2110) -> (refnum out=w2115:refnum<file>, error out=w2116:errorcluster)  [unwired: 1 in, 1 out]
                          n199 = Close File(refnum=w2115, error in=w2116) -> (error out=w2108:errorcluster)  [unwired: 1 out]
                          n200 = call <vilib>:"Simple Error Handler.vi"("error in (no error)"=w2108) -> ()  [unwired: 1 in, 8 out]
                        }
                        frame #6 {
                          w2147 = "\t"
                          w2132 = i16 4 ("width (-)")
                          n201 = local write "C-1K-N"(w2127) -> ()
                          n202 = Wait (ms)(milliseconds to wait=u32 5000) -> ()  [unwired: 1 out]
                          n203 = Open/Create/Replace File(file path (use dialog)=w2128, operation (0:open)=T3."open") -> (refnum out=w2138:refnum<file>, error out=w2139:errorcluster)  [unwired: 2 in, 3 out]
                          n204 = Set File Position(refnum=w2138, from (0:start)=enum16{"start", "end", "current"}."end", error in=w2139) -> (refnum out=w2136:refnum<file>, error out=w2135:errorcluster)  [unwired: 1 in]
                          n205 = call "RLC_read.vi"("Path"=w2129, "String"="cmd /c rlc_read_cCN.py") -> ("MEASURE A"=w2126:dbl, "MEASURE V [V]"=w2131:dbl, "MEASURE B"=w2125:dbl, "MEASURE I [A]"=w2130:dbl)  [unwired: 2 out]
                          n206 = Number To Engineering String(2:w2132, 4:w2130) -> (0:w2146:string)  [unwired: 2 in]
                          n207 = local write "MEASURE A 6"(w2126) -> ()
                          n208 = local write "MEASURE B 6"(w2125) -> ()
                          n209 = Number To Engineering String(2:w2132, 4:w2131) -> (0:w2145:string)  [unwired: 2 in]
                          n210 = Number To Engineering String(2:w2132, 4:w2126) -> (0:w2143:string)  [unwired: 2 in]
                          n211 = Number To Engineering String(2:w2132, 4:w2125) -> (0:w2144:string)  [unwired: 2 in]
                          n212 = Concatenate Strings(w2143, w2147, w2144, w2147, w2145, w2147, w2146, w2147) -> (w2142:string)
                          n213 = Write to Text File(file (use dialog)=w2136, text=w2142, error in=w2135) -> (refnum out=w2140:refnum<file>, error out=w2141:errorcluster)  [unwired: 1 in, 1 out]
                          n214 = Close File(refnum=w2140, error in=w2141) -> (error out=w2133:errorcluster)  [unwired: 1 out]
                          n215 = call <vilib>:"Simple Error Handler.vi"("error in (no error)"=w2133) -> ()  [unwired: 1 in, 8 out]
                        }
                        frame #7 {
                          w2157 = "\t"
                          w2172 = i16 4 ("width (-)")
                          n216 = Wait (ms)(milliseconds to wait=u32 5000) -> ()  [unwired: 1 out]
                          n217 = local write "C-10K-L"(w2152) -> ()
                          n218 = Open/Create/Replace File(file path (use dialog)=w2153, operation (0:open)=T3."open") -> (refnum out=w2166:refnum<file>, error out=w2165:errorcluster)  [unwired: 2 in, 3 out]
                          n219 = Set File Position(refnum=w2166, from (0:start)=enum16{"start", "end", "current"}."end", error in=w2165) -> (refnum out=w2168:refnum<file>, error out=w2169:errorcluster)  [unwired: 1 in]
                          n220 = call "RLC_read.vi"("Path"=w2154, "String"="cmd /c rlc_read_cDL.py") -> ("MEASURE A"=w2151:dbl, "MEASURE V [V]"=w2156:dbl, "MEASURE B"=w2150:dbl, "MEASURE I [A]"=w2155:dbl)  [unwired: 2 out]
                          n221 = Number To Engineering String(2:w2172, 4:w2155) -> (0:w2158:string)  [unwired: 2 in]
                          n222 = local write "MEASURE A 7"(w2151) -> ()
                          n223 = local write "MEASURE B 7"(w2150) -> ()
                          n224 = Number To Engineering String(2:w2172, 4:w2156) -> (0:w2159:string)  [unwired: 2 in]
                          n225 = Number To Engineering String(2:w2172, 4:w2151) -> (0:w2161:string)  [unwired: 2 in]
                          n226 = Number To Engineering String(2:w2172, 4:w2150) -> (0:w2160:string)  [unwired: 2 in]
                          n227 = Concatenate Strings(w2161, w2157, w2160, w2157, w2159, w2157, w2158, w2157) -> (w2162:string)
                          n228 = Write to Text File(file (use dialog)=w2168, text=w2162, error in=w2169) -> (refnum out=w2164:refnum<file>, error out=w2163:errorcluster)  [unwired: 1 in, 1 out]
                          n229 = Close File(refnum=w2164, error in=w2163) -> (error out=w2171:errorcluster)  [unwired: 1 out]
                          n230 = call <vilib>:"Simple Error Handler.vi"("error in (no error)"=w2171) -> ()  [unwired: 1 in, 8 out]
                        }
                        frame #8 {
                          w2182 = "\t"
                          w2197 = i16 4 ("width (-)")
                          n231 = Wait (ms)(milliseconds to wait=u32 5000) -> ()  [unwired: 1 out]
                          n232 = local write "C-10K-N"(w2175) -> ()
                          n233 = Open/Create/Replace File(file path (use dialog)=w2178, operation (0:open)=T3."open") -> (refnum out=w2191:refnum<file>, error out=w2190:errorcluster)  [unwired: 2 in, 3 out]
                          n234 = Set File Position(refnum=w2191, from (0:start)=enum16{"start", "end", "current"}."end", error in=w2190) -> (refnum out=w2193:refnum<file>, error out=w2194:errorcluster)  [unwired: 1 in]
                          n235 = call "RLC_read.vi"("Path"=w2179, "String"="cmd /c rlc_read_cDN.py") -> ("MEASURE A"=w2177:dbl, "MEASURE V [V]"=w2181:dbl, "MEASURE B"=w2176:dbl, "MEASURE I [A]"=w2180:dbl)  [unwired: 2 out]
                          n236 = Number To Engineering String(2:w2197, 4:w2180) -> (0:w2183:string)  [unwired: 2 in]
                          n237 = local write "MEASURE A 8"(w2177) -> ()
                          n238 = local write "MEASURE B 8"(w2176) -> ()
                          n239 = Number To Engineering String(2:w2197, 4:w2181) -> (0:w2184:string)  [unwired: 2 in]
                          n240 = Number To Engineering String(2:w2197, 4:w2177) -> (0:w2186:string)  [unwired: 2 in]
                          n241 = Number To Engineering String(2:w2197, 4:w2176) -> (0:w2185:string)  [unwired: 2 in]
                          n242 = Concatenate Strings(w2186, w2182, w2185, w2182, w2184, w2182, w2183, w2182) -> (w2187:string)
                          n243 = Write to Text File(file (use dialog)=w2193, text=w2187, error in=w2194) -> (refnum out=w2189:refnum<file>, error out=w2188:errorcluster)  [unwired: 1 in, 1 out]
                          n244 = Close File(refnum=w2189, error in=w2188) -> (error out=w2196:errorcluster)  [unwired: 1 out]
                          n245 = call <vilib>:"Simple Error Handler.vi"("error in (no error)"=w2196) -> ()  [unwired: 1 in, 8 out]
                        }
                        frame #9 {
                          w2207 = "\t"
                          w2222 = i16 4 ("width (-)")
                          n246 = local write "Z-50-L"(w2200) -> ()
                          n247 = Wait (ms)(milliseconds to wait=u32 5000) -> ()  [unwired: 1 out]
                          n248 = Open/Create/Replace File(file path (use dialog)=w2203, operation (0:open)=T3."open") -> (refnum out=w2216:refnum<file>, error out=w2215:errorcluster)  [unwired: 2 in, 3 out]
                          n249 = Set File Position(refnum=w2216, from (0:start)=enum16{"start", "end", "current"}."end", error in=w2215) -> (refnum out=w2218:refnum<file>, error out=w2219:errorcluster)  [unwired: 1 in]
                          n250 = call "RLC_read.vi"("Path"=w2204, "String"="cmd /c rlc_read_ZAL.py") -> ("MEASURE A"=w2202:dbl, "MEASURE V [V]"=w2206:dbl, "MEASURE B"=w2201:dbl, "MEASURE I [A]"=w2205:dbl)  [unwired: 2 out]
                          n251 = Number To Engineering String(2:w2222, 4:w2205) -> (0:w2208:string)  [unwired: 2 in]
                          n252 = local write "MEASURE A 9"(w2202) -> ()
                          n253 = local write "MEASURE B 9"(w2201) -> ()
                          n254 = Number To Engineering String(2:w2222, 4:w2206) -> (0:w2209:string)  [unwired: 2 in]
                          n255 = Number To Engineering String(2:w2222, 4:w2202) -> (0:w2211:string)  [unwired: 2 in]
                          n256 = Number To Engineering String(2:w2222, 4:w2201) -> (0:w2210:string)  [unwired: 2 in]
                          n257 = Concatenate Strings(w2211, w2207, w2210, w2207, w2209, w2207, w2208, w2207) -> (w2212:string)
                          n258 = Write to Text File(file (use dialog)=w2218, text=w2212, error in=w2219) -> (refnum out=w2214:refnum<file>, error out=w2213:errorcluster)  [unwired: 1 in, 1 out]
                          n259 = Close File(refnum=w2214, error in=w2213) -> (error out=w2221:errorcluster)  [unwired: 1 out]
                          n260 = call <vilib>:"Simple Error Handler.vi"("error in (no error)"=w2221) -> ()  [unwired: 1 in, 8 out]
                        }
                        frame #10 {
                          w2232 = "\t"
                          w2247 = i16 4 ("width (-)")
                          n261 = local write "Z-50-N"(w2227) -> ()
                          n262 = Wait (ms)(milliseconds to wait=u32 5000) -> ()  [unwired: 1 out]
                          n263 = Open/Create/Replace File(file path (use dialog)=w2228, operation (0:open)=T3."open") -> (refnum out=w2241:refnum<file>, error out=w2240:errorcluster)  [unwired: 2 in, 3 out]
                          n264 = Set File Position(refnum=w2241, from (0:start)=enum16{"start", "end", "current"}."end", error in=w2240) -> (refnum out=w2243:refnum<file>, error out=w2244:errorcluster)  [unwired: 1 in]
                          n265 = call "RLC_read.vi"("Path"=w2229, "String"="cmd /c rlc_read_ZAN.py") -> ("MEASURE A"=w2226:dbl, "MEASURE V [V]"=w2231:dbl, "MEASURE B"=w2225:dbl, "MEASURE I [A]"=w2230:dbl)  [unwired: 2 out]
                          n266 = Number To Engineering String(2:w2247, 4:w2230) -> (0:w2233:string)  [unwired: 2 in]
                          n267 = local write "MEASURE A 10"(w2226) -> ()
                          n268 = local write "MEASURE B 10"(w2225) -> ()
                          n269 = Number To Engineering String(2:w2247, 4:w2231) -> (0:w2234:string)  [unwired: 2 in]
                          n270 = Number To Engineering String(2:w2247, 4:w2226) -> (0:w2236:string)  [unwired: 2 in]
                          n271 = Number To Engineering String(2:w2247, 4:w2225) -> (0:w2235:string)  [unwired: 2 in]
                          n272 = Concatenate Strings(w2236, w2232, w2235, w2232, w2234, w2232, w2233, w2232) -> (w2237:string)
                          n273 = Write to Text File(file (use dialog)=w2243, text=w2237, error in=w2244) -> (refnum out=w2239:refnum<file>, error out=w2238:errorcluster)  [unwired: 1 in, 1 out]
                          n274 = Close File(refnum=w2239, error in=w2238) -> (error out=w2246:errorcluster)  [unwired: 1 out]
                          n275 = call <vilib>:"Simple Error Handler.vi"("error in (no error)"=w2246) -> ()  [unwired: 1 in, 8 out]
                        }
                        frame #11 {
                          w2257 = "\t"
                          w2272 = i16 4 ("width (-)")
                          n276 = Wait (ms)(milliseconds to wait=u32 5000) -> ()  [unwired: 1 out]
                          n277 = local write "Z-100-L"(w2250) -> ()
                          n278 = Open/Create/Replace File(file path (use dialog)=w2253, operation (0:open)=T3."open") -> (refnum out=w2266:refnum<file>, error out=w2265:errorcluster)  [unwired: 2 in, 3 out]
                          n279 = Set File Position(refnum=w2266, from (0:start)=enum16{"start", "end", "current"}."end", error in=w2265) -> (refnum out=w2268:refnum<file>, error out=w2269:errorcluster)  [unwired: 1 in]
                          n280 = call "RLC_read.vi"("Path"=w2254, "String"="cmd /c rlc_read_ZBL.py") -> ("MEASURE A"=w2252:dbl, "MEASURE V [V]"=w2256:dbl, "MEASURE B"=w2251:dbl, "MEASURE I [A]"=w2255:dbl)  [unwired: 2 out]
                          n281 = Number To Engineering String(2:w2272, 4:w2255) -> (0:w2258:string)  [unwired: 2 in]
                          n282 = local write "MEASURE A 11"(w2252) -> ()
                          n283 = local write "MEASURE B 11"(w2251) -> ()
                          n284 = Number To Engineering String(2:w2272, 4:w2256) -> (0:w2259:string)  [unwired: 2 in]
                          n285 = Number To Engineering String(2:w2272, 4:w2252) -> (0:w2261:string)  [unwired: 2 in]
                          n286 = Number To Engineering String(2:w2272, 4:w2251) -> (0:w2260:string)  [unwired: 2 in]
                          n287 = Concatenate Strings(w2261, w2257, w2260, w2257, w2259, w2257, w2258, w2257) -> (w2262:string)
                          n288 = Write to Text File(file (use dialog)=w2268, text=w2262, error in=w2269) -> (refnum out=w2264:refnum<file>, error out=w2263:errorcluster)  [unwired: 1 in, 1 out]
                          n289 = Close File(refnum=w2264, error in=w2263) -> (error out=w2271:errorcluster)  [unwired: 1 out]
                          n290 = call <vilib>:"Simple Error Handler.vi"("error in (no error)"=w2271) -> ()  [unwired: 1 in, 8 out]
                        }
                        frame #12 {
                          w2282 = "\t"
                          w2297 = i16 4 ("width (-)")
                          n291 = Wait (ms)(milliseconds to wait=u32 5000) -> ()  [unwired: 1 out]
                          n292 = local write "Z-100-N"(w2277) -> ()
                          n293 = Open/Create/Replace File(file path (use dialog)=w2278, operation (0:open)=T3."open") -> (refnum out=w2291:refnum<file>, error out=w2290:errorcluster)  [unwired: 2 in, 3 out]
                          n294 = Set File Position(refnum=w2291, from (0:start)=enum16{"start", "end", "current"}."end", error in=w2290) -> (refnum out=w2293:refnum<file>, error out=w2294:errorcluster)  [unwired: 1 in]
                          n295 = call "RLC_read.vi"("Path"=w2279, "String"="cmd /c rlc_read_ZBN.py") -> ("MEASURE A"=w2276:dbl, "MEASURE V [V]"=w2281:dbl, "MEASURE B"=w2275:dbl, "MEASURE I [A]"=w2280:dbl)  [unwired: 2 out]
                          n296 = Number To Engineering String(2:w2297, 4:w2280) -> (0:w2283:string)  [unwired: 2 in]
                          n297 = local write "MEASURE A 12"(w2276) -> ()
                          n298 = local write "MEASURE B 12"(w2275) -> ()
                          n299 = Number To Engineering String(2:w2297, 4:w2281) -> (0:w2284:string)  [unwired: 2 in]
                          n300 = Number To Engineering String(2:w2297, 4:w2276) -> (0:w2286:string)  [unwired: 2 in]
                          n301 = Number To Engineering String(2:w2297, 4:w2275) -> (0:w2285:string)  [unwired: 2 in]
                          n302 = Concatenate Strings(w2286, w2282, w2285, w2282, w2284, w2282, w2283, w2282) -> (w2287:string)
                          n303 = Write to Text File(file (use dialog)=w2293, text=w2287, error in=w2294) -> (refnum out=w2289:refnum<file>, error out=w2288:errorcluster)  [unwired: 1 in, 1 out]
                          n304 = Close File(refnum=w2289, error in=w2288) -> (error out=w2296:errorcluster)  [unwired: 1 out]
                          n305 = call <vilib>:"Simple Error Handler.vi"("error in (no error)"=w2296) -> ()  [unwired: 1 in, 8 out]
                        }
                        frame #13 {
                          w2307 = "\t"
                          w2322 = i16 4 ("width (-)")
                          n306 = local write "Z-1K-L"(w2302) -> ()
                          n307 = Wait (ms)(milliseconds to wait=u32 5000) -> ()  [unwired: 1 out]
                          n308 = Open/Create/Replace File(file path (use dialog)=w2303, operation (0:open)=T3."open") -> (refnum out=w2316:refnum<file>, error out=w2315:errorcluster)  [unwired: 2 in, 3 out]
                          n309 = Set File Position(refnum=w2316, from (0:start)=enum16{"start", "end", "current"}."end", error in=w2315) -> (refnum out=w2318:refnum<file>, error out=w2319:errorcluster)  [unwired: 1 in]
                          n310 = call "RLC_read.vi"("Path"=w2304, "String"="cmd /c rlc_read_ZCL.py") -> ("MEASURE A"=w2301:dbl, "MEASURE V [V]"=w2306:dbl, "MEASURE B"=w2300:dbl, "MEASURE I [A]"=w2305:dbl)  [unwired: 2 out]
                          n311 = Number To Engineering String(2:w2322, 4:w2305) -> (0:w2308:string)  [unwired: 2 in]
                          n312 = local write "MEASURE A 13"(w2301) -> ()
                          n313 = local write "MEASURE B 13"(w2300) -> ()
                          n314 = Number To Engineering String(2:w2322, 4:w2306) -> (0:w2309:string)  [unwired: 2 in]
                          n315 = Number To Engineering String(2:w2322, 4:w2301) -> (0:w2311:string)  [unwired: 2 in]
                          n316 = Number To Engineering String(2:w2322, 4:w2300) -> (0:w2310:string)  [unwired: 2 in]
                          n317 = Concatenate Strings(w2311, w2307, w2310, w2307, w2309, w2307, w2308, w2307) -> (w2312:string)
                          n318 = Write to Text File(file (use dialog)=w2318, text=w2312, error in=w2319) -> (refnum out=w2314:refnum<file>, error out=w2313:errorcluster)  [unwired: 1 in, 1 out]
                          n319 = Close File(refnum=w2314, error in=w2313) -> (error out=w2321:errorcluster)  [unwired: 1 out]
                          n320 = call <vilib>:"Simple Error Handler.vi"("error in (no error)"=w2321) -> ()  [unwired: 1 in, 8 out]
                        }
                        frame #14 {
                          w2332 = "\t"
                          w2347 = i16 4 ("width (-)")
                          n321 = local write "Z-1K-N"(w2327) -> ()
                          n322 = Wait (ms)(milliseconds to wait=u32 5000) -> ()  [unwired: 1 out]
                          n323 = Open/Create/Replace File(file path (use dialog)=w2328, operation (0:open)=T3."open") -> (refnum out=w2341:refnum<file>, error out=w2340:errorcluster)  [unwired: 2 in, 3 out]
                          n324 = Set File Position(refnum=w2341, from (0:start)=enum16{"start", "end", "current"}."end", error in=w2340) -> (refnum out=w2343:refnum<file>, error out=w2344:errorcluster)  [unwired: 1 in]
                          n325 = call "RLC_read.vi"("Path"=w2329, "String"="cmd /c rlc_read_ZCN.py") -> ("MEASURE A"=w2326:dbl, "MEASURE V [V]"=w2331:dbl, "MEASURE B"=w2325:dbl, "MEASURE I [A]"=w2330:dbl)  [unwired: 2 out]
                          n326 = Number To Engineering String(2:w2347, 4:w2330) -> (0:w2333:string)  [unwired: 2 in]
                          n327 = local write "MEASURE A 14"(w2326) -> ()
                          n328 = local write "MEASURE B 14"(w2325) -> ()
                          n329 = Number To Engineering String(2:w2347, 4:w2331) -> (0:w2334:string)  [unwired: 2 in]
                          n330 = Number To Engineering String(2:w2347, 4:w2326) -> (0:w2336:string)  [unwired: 2 in]
                          n331 = Number To Engineering String(2:w2347, 4:w2325) -> (0:w2335:string)  [unwired: 2 in]
                          n332 = Concatenate Strings(w2336, w2332, w2335, w2332, w2334, w2332, w2333, w2332) -> (w2337:string)
                          n333 = Write to Text File(file (use dialog)=w2343, text=w2337, error in=w2344) -> (refnum out=w2339:refnum<file>, error out=w2338:errorcluster)  [unwired: 1 in, 1 out]
                          n334 = Close File(refnum=w2339, error in=w2338) -> (error out=w2346:errorcluster)  [unwired: 1 out]
                          n335 = call <vilib>:"Simple Error Handler.vi"("error in (no error)"=w2346) -> ()  [unwired: 1 in, 8 out]
                        }
                        frame #15 {
                          w2357 = "\t"
                          w2372 = i16 4 ("width (-)")
                          n336 = Wait (ms)(milliseconds to wait=u32 5000) -> ()  [unwired: 1 out]
                          n337 = local write "Z-10K-L"(w2350) -> ()
                          n338 = Open/Create/Replace File(file path (use dialog)=w2353, operation (0:open)=T3."open") -> (refnum out=w2366:refnum<file>, error out=w2365:errorcluster)  [unwired: 2 in, 3 out]
                          n339 = Set File Position(refnum=w2366, from (0:start)=enum16{"start", "end", "current"}."end", error in=w2365) -> (refnum out=w2368:refnum<file>, error out=w2369:errorcluster)  [unwired: 1 in]
                          n340 = call "RLC_read.vi"("Path"=w2354, "String"="cmd /c rlc_read_ZDL.py") -> ("MEASURE A"=w2352:dbl, "MEASURE V [V]"=w2356:dbl, "MEASURE B"=w2351:dbl, "MEASURE I [A]"=w2355:dbl)  [unwired: 2 out]
                          n341 = Number To Engineering String(2:w2372, 4:w2355) -> (0:w2358:string)  [unwired: 2 in]
                          n342 = local write "MEASURE A 15"(w2352) -> ()
                          n343 = local write "MEASURE B 15"(w2351) -> ()
                          n344 = Number To Engineering String(2:w2372, 4:w2356) -> (0:w2359:string)  [unwired: 2 in]
                          n345 = Number To Engineering String(2:w2372, 4:w2352) -> (0:w2361:string)  [unwired: 2 in]
                          n346 = Number To Engineering String(2:w2372, 4:w2351) -> (0:w2360:string)  [unwired: 2 in]
                          n347 = Concatenate Strings(w2361, w2357, w2360, w2357, w2359, w2357, w2358, w2357) -> (w2362:string)
                          n348 = Write to Text File(file (use dialog)=w2368, text=w2362, error in=w2369) -> (refnum out=w2364:refnum<file>, error out=w2363:errorcluster)  [unwired: 1 in, 1 out]
                          n349 = Close File(refnum=w2364, error in=w2363) -> (error out=w2371:errorcluster)  [unwired: 1 out]
                          n350 = call <vilib>:"Simple Error Handler.vi"("error in (no error)"=w2371) -> ()  [unwired: 1 in, 8 out]
                        }
                        frame #16 {
                          w2383 = "\t"
                          w2398 = i16 4 ("width (-)")
                          n351 = Wait (ms)(milliseconds to wait=u32 5000) -> ()  [unwired: 1 out]
                          n352 = local write "Z-10K-N"(w2377) -> ()
                          n353 = Open/Create/Replace File(file path (use dialog)=w2378, operation (0:open)=T3."open") -> (refnum out=w2392:refnum<file>, error out=w2391:errorcluster)  [unwired: 2 in, 3 out]
                          n354 = Set File Position(refnum=w2392, from (0:start)=enum16{"start", "end", "current"}."end", error in=w2391) -> (refnum out=w2394:refnum<file>, error out=w2395:errorcluster)  [unwired: 1 in]
                          n355 = call "RLC_read.vi"("Path"=w2379, "String"="cmd /c rlc_read_ZDN.py") -> ("MEASURE A"=w2376:dbl, "MEASURE V [V]"=w2382:dbl, "MEASURE B"=w2375:dbl, "MEASURE I [A]"=w2381:dbl)  [unwired: 2 out]
                          n356 = Number To Engineering String(2:w2398, 4:w2381) -> (0:w2384:string)  [unwired: 2 in]
                          n357 = local write "MEASURE A 16"(w2376) -> ()
                          n358 = local write "MEASURE B 16"(w2375) -> ()
                          n359 = Number To Engineering String(2:w2398, 4:w2382) -> (0:w2385:string)  [unwired: 2 in]
                          n360 = Number To Engineering String(2:w2398, 4:w2376) -> (0:w2387:string)  [unwired: 2 in]
                          n361 = Number To Engineering String(2:w2398, 4:w2375) -> (0:w2386:string)  [unwired: 2 in]
                          n362 = Concatenate Strings(w2387, w2383, w2386, w2383, w2385, w2383, w2384, w2383, "\r\n") -> (w2388:string)
                          n363 = Write to Text File(file (use dialog)=w2394, text=w2388, error in=w2395) -> (refnum out=w2390:refnum<file>, error out=w2389:errorcluster)  [unwired: 1 in, 1 out]
                          n364 = Close File(refnum=w2390, error in=w2389) -> (error out=w2397:errorcluster)  [unwired: 1 out]
                          n365 = call <vilib>:"Simple Error Handler.vi"("error in (no error)"=w2397) -> ()  [unwired: 1 in, 8 out]
                        }
                        frame #17 {
                          n366 = local write "Z-50-N"(w2401) -> ()
                          n367 = local write "Z-50-L"(w2401) -> ()
                          n368 = local write "C-1K-N"(w2401) -> ()
                          n369 = local write "C-50-N"(w2401) -> ()
                          n370 = local write "C-50-L"(w2401) -> ()
                          n371 = local write "Z-1K-N"(w2401) -> ()
                          n372 = local write "C-1K-L"(w2401) -> ()
                          n373 = local write "Z-1K-L"(w2401) -> ()
                          n374 = local write "Z-100-L"(w2401) -> ()
                          n375 = local write "C-10K-L"(w2401) -> ()
                          n376 = local write "Z-10K-L"(w2401) -> ()
                          n377 = local write "C-10K-N"(w2401) -> ()
                          n378 = local write "Z-10K-N"(w2401) -> ()
                          n379 = local write "C-100-N"(w2401) -> ()
                          n380 = local write "C-100-L"(w2401) -> ()
                          n381 = local write "Z-100-N"(w2401) -> ()
                        }
                      }
                    }
                    n382 = call <vilib>:"Mean.vi"("X"=w1952) -> ("mean"=w1935:dbl)  [unwired: 1 out]
                    n383 = call <vilib>:"Mean.vi"("X"=w1951) -> ("mean"=w1934:dbl)  [unwired: 1 out]
                    n384 = call <vilib>:"Mean.vi"("X"=w1950) -> ("mean"=w1933:dbl)  [unwired: 1 out]
                    n385 = call <vilib>:"Mean.vi"("X"=w1949) -> ("mean"=w1932:dbl)  [unwired: 1 out]
                    n386 = call <vilib>:"Mean.vi"("X"=w1948) -> ("mean"=w1931:dbl)  [unwired: 1 out]
                    n387 = call <vilib>:"Mean.vi"("X"=w1947) -> ("mean"=w1930:dbl)  [unwired: 1 out]
                    n388 = call <vilib>:"Mean.vi"("X"=w1946) -> ("mean"=w1929:dbl)  [unwired: 1 out]
                    n389 = call <vilib>:"Mean.vi"("X"=w1945) -> ("mean"=w1928:dbl)  [unwired: 1 out]
                    n390 = call <vilib>:"Mean.vi"("X"=w1944) -> ("mean"=w1927:dbl)  [unwired: 1 out]
                    n391 = call <vilib>:"Mean.vi"("X"=w1943) -> ("mean"=w1926:dbl)  [unwired: 1 out]
                    n392 = call <vilib>:"Mean.vi"("X"=w1942) -> ("mean"=w1925:dbl)  [unwired: 1 out]
                    n393 = call <vilib>:"Mean.vi"("X"=w1941) -> ("mean"=w1924:dbl)  [unwired: 1 out]
                    n394 = call <vilib>:"Mean.vi"("X"=w1940) -> ("mean"=w1923:dbl)  [unwired: 1 out]
                    n395 = call <vilib>:"Mean.vi"("X"=w1939) -> ("mean"=w1922:dbl)  [unwired: 1 out]
                    n396 = call <vilib>:"Mean.vi"("X"=w1938) -> ("mean"=w1921:dbl)  [unwired: 1 out]
                    n397 = call <vilib>:"Mean.vi"("X"=w1937) -> ("mean"=w1920:dbl)  [unwired: 1 out]
                    n398 = local write "mean"(w1935) -> ()
                    n399 = local write "mean 2"(w1934) -> ()
                    n400 = local write "mean 3"(w1933) -> ()
                    n401 = local write "mean 4"(w1932) -> ()
                    n402 = local write "mean 5"(w1931) -> ()
                    n403 = local write "mean 6"(w1930) -> ()
                    n404 = local write "mean 7"(w1929) -> ()
                    n405 = local write "mean 8"(w1928) -> ()
                    n406 = local write "mean 9"(w1927) -> ()
                    n407 = local write "mean 10"(w1926) -> ()
                    n408 = local write "mean 11"(w1925) -> ()
                    n409 = local write "mean 12"(w1924) -> ()
                    n410 = local write "mean 13"(w1923) -> ()
                    n411 = local write "mean 14"(w1922) -> ()
                    n412 = local write "mean 15"(w1921) -> ()
                    n413 = local write "mean 16"(w1920) -> ()
                  }
                }
              }
              frame #2 {
                n414 = case shown="True" w2403 {
                  tunnel: w2420 -> [_ w2436]
                  tunnel: w2419 -> [_ w2435]
                  tunnel: w2418 -> [_ w2434]
                  tunnel: w2417 -> [_ w2433]
                  tunnel: w2416 -> [_ w2432]
                  tunnel: w2415 -> [_ w2431]
                  tunnel: w2414 -> [_ w2430]
                  tunnel: w2413 -> [_ w2429]
                  tunnel: w2412 -> [_ w2428]
                  tunnel: w2411 -> [_ w2427]
                  tunnel: w2410 -> [_ w2426]
                  tunnel: w2409 -> [_ w2425]
                  tunnel: w2408 -> [_ w2424]
                  tunnel: w2407 -> [_ w2423]
                  tunnel: w2406 -> [_ w2422]
                  tunnel: w2405 -> [_ w2421]
                  frame False {
                  }
                  frame True {
                    w2451 = "\t"
                    w2468 = i16 4 ("precision (6)")
                    n415 = property on="SET" class="DigNum (strict)"() -> ("Value"=w2437:i32)  [unwired: 2 in, 2 out]
                    n416 = Number To Engineering String(2:w2468, 4:w2436) -> (0:w2466:string)  [unwired: 2 in]
                    n417 = Number To Engineering String(2:w2468, 4:w2435) -> (0:w2465:string)  [unwired: 2 in]
                    n418 = Number To Engineering String(2:w2468, 4:w2434) -> (0:w2464:string)  [unwired: 2 in]
                    n419 = Number To Engineering String(2:w2468, 4:w2433) -> (0:w2463:string)  [unwired: 2 in]
                    n420 = Number To Engineering String(2:w2468, 4:w2432) -> (0:w2462:string)  [unwired: 2 in]
                    n421 = Number To Engineering String(2:w2468, 4:w2431) -> (0:w2461:string)  [unwired: 2 in]
                    n422 = Number To Engineering String(2:w2468, 4:w2430) -> (0:w2460:string)  [unwired: 2 in]
                    n423 = Number To Engineering String(2:w2468, 4:w2429) -> (0:w2459:string)  [unwired: 2 in]
                    n424 = Number To Engineering String(2:w2468, 4:w2428) -> (0:w2458:string)  [unwired: 2 in]
                    n425 = Number To Engineering String(2:w2468, 4:w2427) -> (0:w2457:string)  [unwired: 2 in]
                    n426 = Number To Engineering String(2:w2468, 4:w2421) -> (0:w2456:string)  [unwired: 2 in]
                    n427 = Number To Engineering String(2:w2468, 4:w2426) -> (0:w2455:string)  [unwired: 2 in]
                    n428 = Number To Engineering String(2:w2468, 4:w2425) -> (0:w2454:string)  [unwired: 2 in]
                    n429 = Number To Engineering String(2:w2468, 4:w2424) -> (0:w2453:string)  [unwired: 2 in]
                    n430 = Number To Engineering String(2:w2468, 4:w2423) -> (0:w2452:string)  [unwired: 2 in]
                    n431 = Number To Engineering String(2:w2468, 4:w2422) -> (0:w2450:string)  [unwired: 2 in]
                    n432 = Number To Decimal String(number=w2437) -> (decimal integer string=w2467:string)  [unwired: 1 in]
                    n433 = property on="path RLC_mean" class="Path"() -> ("Value"=w2438:path)  [unwired: 2 in, 2 out]
                    n434 = Open/Create/Replace File(file path (use dialog)=w2438, operation (0:open)=T3."open") -> (refnum out=w2443:refnum<file>, error out=w2442:errorcluster)  [unwired: 2 in, 3 out]
                    n435 = Concatenate Strings(w2467, w2451, w2466, w2451, w2465, w2451, w2464, w2451, w2463, w2451, w2462, w2451, w2461, w2451, w2460, w2451, w2459, w2451, w2458, w2451, w2457, w2451, w2456, w2451, w2455, w2451, w2454, w2451, w2453, w2451, w2452, w2451, w2450, "\r\n") -> (w2439:string)
                    n436 = Set File Position(refnum=w2443, from (0:start)=enum16{"start", "end", "current"}."end", error in=w2442) -> (refnum out=w2445:refnum<file>, error out=w2446:errorcluster)  [unwired: 1 in]
                    n437 = Write to Text File(file (use dialog)=w2445, text=w2439, error in=w2446) -> (refnum out=w2441:refnum<file>, error out=w2440:errorcluster)  [unwired: 1 in, 1 out]
                    n438 = Close File(refnum=w2441, error in=w2440) -> (error out=w2448:errorcluster)  [unwired: 1 out]
                    n439 = call <vilib>:"Simple Error Handler.vi"("error in (no error)"=w2448) -> ()  [unwired: 1 in, 8 out]
                  }
                }
              }
            }
            n440 = local write "graph RLC"(w1875) -> ()
          }
        }
        n441 = for {
          N: "N to fit" -> [_]
          tunnel: [w2552] -> w1848 mode=indexing
          tunnel: [w2557] -> w1866 mode=indexing
          tunnel: [w2557] -> w1852 mode=indexing
          tunnel: [w2545] -> w1857 mode=indexing
          i -> [w2557]
          n442 = property on="ON/OFF" class="Bool (strict)"() -> ("Value"=w2536:bool)  [unwired: 2 in, 2 out]
          n443 = property on="Manual Ctrl" class="Bool (strict)"() -> ("Value"=w2539:bool)  [unwired: 2 in, 2 out]
          n444 = property on="Save - Sievert 01" class="Bool (strict)"() -> ("Value"=w2540:bool)  [unwired: 2 in, 2 out]
          n445 = And(x=w2539, y=w2540) -> (x .and. y?=w2538:bool)
          n446 = case shown="True" "Câmara" {
            frame False {
            }
            frame True {
              n447 = property on="Vol Ref" class="Slide (strict)"() -> ("Value"=w2675:dbl)  [unwired: 2 in, 2 out]
              n448 = local write "Camara"(w2675) -> ()
            }
          }
          n449 = case shown="False" "Clear" {
            frame False {
            }
            frame True {
              n450 = property on="P-manual" class="WFChart (strict)"("History Data"=dynamicdata[] []) -> ()  [unwired: 2 in, 2 out]
            }
          }
          n451 = stacked-sequence {
            tunnel: "Entrada Gás" -> [w2706 _ _ _]
            tunnel: "Vácuo" -> [_ w2718 _ _]
            tunnel: "Câmara" -> [_ _ w2730 _]
            tunnel: "ATM" -> [_ _ _ w2742]
            frame #0 {
              w2711 = T4 3 items=["no dialog", "OK message", "continue or stop message", "OK message + warnings", "continue/stop + warnings"] ("type of dialog (OK msg:1)")
              n452 = property on="Entrada gás" class="Bool (strict)"("Value"=w2706) -> ()  [unwired: 2 in, 2 out]
              n453 = call-poly <vilib>:"DAQmx Create Virtual Channel.vi"("lines"=tag "Dev1/port0/line1") -> ("task out"=w2709:refnum<k21>, "error out"=w2710:errorcluster)  [unwired: 13 in]
              n454 = call <vilib>:"DAQmx Start Task.vi"("task/channels in"=w2709, "error in"=w2710) -> ("task out"=w2712:refnum<k21>, "error out"=w2713:errorcluster)  [unwired: 12 in]
              n455 = call-poly <vilib>:"DAQmx Write.vi"("task/channels in"=w2712, "data"=w2706, "error in"=w2713) -> ("task out"=w2717:refnum<k21>, "error out"=w2714:errorcluster)  [unwired: 10 in, 1 out]
              n456 = call <vilib>:"DAQmx Stop Task.vi"("task/channels in"=w2717, "error in"=w2714) -> ("task out"=w2716:refnum<k21>, "error out"=w2715:errorcluster)  [unwired: 12 in]
              n457 = call <vilib>:"DAQmx Clear Task.vi"("task in"=w2716, "error in"=w2715) -> ("error out"=w2708:errorcluster)  [unwired: 13 in]
              n458 = call <vilib>:"Simple Error Handler.vi"("type of dialog (OK msg:1)"=w2711, "error in (no error)"=w2708) -> ()  [unwired: 3 in, 5 out]
            }
            frame #1 {
              w2723 = T4 3 items=["no dialog", "OK message", "continue or stop message", "OK message + warnings", "continue/stop + warnings"] ("type of dialog (OK msg:1)")
              n459 = property on="Vácuo" class="Bool (strict)"("Value"=w2718) -> ()  [unwired: 2 in, 2 out]
              n460 = call-poly <vilib>:"DAQmx Create Virtual Channel.vi"("lines"=tag "Dev1/port0/line2") -> ("task out"=w2721:refnum<k21>, "error out"=w2722:errorcluster)  [unwired: 13 in]
              n461 = call <vilib>:"DAQmx Start Task.vi"("task/channels in"=w2721, "error in"=w2722) -> ("task out"=w2724:refnum<k21>, "error out"=w2725:errorcluster)  [unwired: 12 in]
              n462 = call-poly <vilib>:"DAQmx Write.vi"("task/channels in"=w2724, "data"=w2718, "error in"=w2725) -> ("task out"=w2729:refnum<k21>, "error out"=w2726:errorcluster)  [unwired: 10 in, 1 out]
              n463 = call <vilib>:"DAQmx Stop Task.vi"("task/channels in"=w2729, "error in"=w2726) -> ("task out"=w2728:refnum<k21>, "error out"=w2727:errorcluster)  [unwired: 12 in]
              n464 = call <vilib>:"DAQmx Clear Task.vi"("task in"=w2728, "error in"=w2727) -> ("error out"=w2720:errorcluster)  [unwired: 13 in]
              n465 = call <vilib>:"Simple Error Handler.vi"("type of dialog (OK msg:1)"=w2723, "error in (no error)"=w2720) -> ()  [unwired: 3 in, 5 out]
            }
            frame #2 {
              w2735 = T4 3 items=["no dialog", "OK message", "continue or stop message", "OK message + warnings", "continue/stop + warnings"] ("type of dialog (OK msg:1)")
              n466 = property on="Câmara" class="Bool (strict)"("Value"=w2730) -> ()  [unwired: 2 in, 2 out]
              n467 = call-poly <vilib>:"DAQmx Create Virtual Channel.vi"("lines"=tag "Dev1/port0/line3") -> ("task out"=w2733:refnum<k21>, "error out"=w2734:errorcluster)  [unwired: 13 in]
              n468 = call <vilib>:"DAQmx Start Task.vi"("task/channels in"=w2733, "error in"=w2734) -> ("task out"=w2736:refnum<k21>, "error out"=w2737:errorcluster)  [unwired: 12 in]
              n469 = call-poly <vilib>:"DAQmx Write.vi"("task/channels in"=w2736, "data"=w2730, "error in"=w2737) -> ("task out"=w2741:refnum<k21>, "error out"=w2738:errorcluster)  [unwired: 10 in, 1 out]
              n470 = call <vilib>:"DAQmx Stop Task.vi"("task/channels in"=w2741, "error in"=w2738) -> ("task out"=w2740:refnum<k21>, "error out"=w2739:errorcluster)  [unwired: 12 in]
              n471 = call <vilib>:"DAQmx Clear Task.vi"("task in"=w2740, "error in"=w2739) -> ("error out"=w2732:errorcluster)  [unwired: 13 in]
              n472 = call <vilib>:"Simple Error Handler.vi"("type of dialog (OK msg:1)"=w2735, "error in (no error)"=w2732) -> ()  [unwired: 3 in, 5 out]
            }
            frame #3 {
              w2747 = T4 3 items=["no dialog", "OK message", "continue or stop message", "OK message + warnings", "continue/stop + warnings"] ("type of dialog (OK msg:1)")
              n473 = property on="Atm" class="Bool (strict)"("Value"=w2742) -> ()  [unwired: 2 in, 2 out]
              n474 = call-poly <vilib>:"DAQmx Create Virtual Channel.vi"("lines"=tag "Dev1/port0/line4") -> ("task out"=w2745:refnum<k21>, "error out"=w2746:errorcluster)  [unwired: 13 in]
              n475 = call <vilib>:"DAQmx Start Task.vi"("task/channels in"=w2745, "error in"=w2746) -> ("task out"=w2748:refnum<k21>, "error out"=w2749:errorcluster)  [unwired: 12 in]
              n476 = call-poly <vilib>:"DAQmx Write.vi"("task/channels in"=w2748, "data"=w2742, "error in"=w2749) -> ("task out"=w2753:refnum<k21>, "error out"=w2750:errorcluster)  [unwired: 10 in, 1 out]
              n477 = call <vilib>:"DAQmx Stop Task.vi"("task/channels in"=w2753, "error in"=w2750) -> ("task out"=w2752:refnum<k21>, "error out"=w2751:errorcluster)  [unwired: 12 in]
              n478 = call <vilib>:"DAQmx Clear Task.vi"("task in"=w2752, "error in"=w2751) -> ("error out"=w2744:errorcluster)  [unwired: 13 in]
              n479 = call <vilib>:"Simple Error Handler.vi"("type of dialog (OK msg:1)"=w2747, "error in (no error)"=w2744) -> ()  [unwired: 3 in, 5 out]
            }
          }
          n480 = case shown="True" w2536 {
            frame False {
            }
            frame True {
              n481 = property on="Auto Ctrl" class="Bool (strict)"() -> ("Value"=w2563:bool)  [unwired: 2 in, 2 out]
              n482 = case shown="True" w2563 {
                tunnel: [w2564 w2569] -> w2561
                tunnel: [w2565 w2568] -> w2562
                tunnel: [w2566 w2567] -> w2560
                frame False {
                  n483 = property on="S#01" class="DigNum (strict)"() -> ("Value"=w2566:dbl)  [unwired: 2 in, 2 out]
                  n484 = property on="T fit" class="DigNum (strict)"() -> ("Value"=w2564:dbl)  [unwired: 2 in, 2 out]
                  n485 = property on="termopar K" class="DigNum (strict)"() -> ("Value"=w2565:dbl)  [unwired: 2 in, 2 out]
                }
                frame True {
                  n486 = property on="termopar K 2" class="DigNum (strict)"() -> ("Value"=w2568:dbl)  [unwired: 2 in, 2 out]
                  n487 = property on="S#1_auto" class="DigNum (strict)"() -> ("Value"=w2567:dbl)  [unwired: 2 in, 2 out]
                  n488 = property on="T fit" class="DigNum (strict)"() -> ("Value"=w2569:dbl)  [unwired: 2 in, 2 out]
                }
              }
              n489 = Merge Signals(w2560, w2561, w2562) -> (w2559:dynamicdata)
              n490 = property on="Waveform Chart 2" class="WFChart (strict)"("Value"=w2559) -> ()  [unwired: 2 in, 2 out]
            }
          }
          n491 = case shown="True" "Guardar\nCinetica" {
            frame False {
            }
            frame True {
              n492 = feedback #3() -> (w2628:bool)  [unwired: 1 in]
              "x >= y?" <- w2628
              n493 = call "Elapsed Time"("Reset"=w2628) -> ("Elapsed Time (s)"=w2630:dbl)  [unwired: 11 in, 7 out]
              "Elapsed Time (sec)" <- w2630
              n494 = case shown="True" w2628 {
                frame False {
                }
                frame True {
                  n495 = flat-sequence {
                    tunnel: [w2647] -> w2633
                    tunnel: [w2646] -> w2632
                    tunnel: w2633 -> [w2665]
                    tunnel: w2632 -> [w2664]
                    frame #0 {
                      w2635 = "\t"
                      w2638 = i16 6 ("precision (6)")
                      n496 = property on="P cinetica mean" class="DigNum (strict)"() -> ("Value"=w2644:dbl)  [unwired: 2 in, 2 out]
                      n497 = property on="MEASURE R [Ohm ]" class="DigNum (strict)"() -> ("Value"=w2637:dbl)  [unwired: 2 in, 2 out]
                      n498 = property on="T cinetica mean 2" class="DigNum (strict)"() -> ("Value"=w2643:dbl)  [unwired: 2 in, 2 out]
                      n499 = property on="termopar K" class="DigNum (strict)"() -> ("Value"=w2641:dbl)  [unwired: 2 in, 2 out]
                      n500 = property on="MEASURE C [F ]" class="DigNum (strict)"() -> ("Value"=w2639:dbl)  [unwired: 2 in, 2 out]
                      n501 = property on="path 2_cinetica" class="Path"() -> ("Value"=w2645:path)  [unwired: 2 in, 2 out]
                      n502 = Number To Fractional String(number=w2644, precision (6)=w2638) -> (F-format string=w2659:string)  [unwired: 2 in]
                      n503 = Number To Fractional String(number=w2643, precision (6)=w2638) -> (F-format string=w2658:string)  [unwired: 2 in]
                      n504 = Number To Fractional String(number=w2641, precision (6)=w2638) -> (F-format string=w2642:string)  [unwired: 2 in]
                      n505 = Number To Exponential String(number=w2639, precision (6)=w2638) -> (E-format string=w2640:string)  [unwired: 2 in]
                      n506 = Number To Exponential String(number=w2637, precision (6)=w2638) -> (E-format string=w2636:string)  [unwired: 2 in]
                      n507 = Get Date/Time String(date format (0)=enum16{"short", "long", "abbreviated"}."short", want seconds? (F)=TRUE) -> (date string=w2661:string, time string=w2660:string)  [unwired: 1 in]
                      n508 = Open/Create/Replace File(file path (use dialog)=w2645, operation (0:open)=T3."open") -> (refnum out=w2654:refnum<file>, error out=w2655:errorcluster)  [unwired: 2 in, 3 out]
                      n509 = Concatenate Strings(w2661, w2635, w2660, w2635, w2659, w2635, w2658, w2635, w2642, w2635, w2640, w2635, w2636, w2635, "\r\n") -> (w2648:string)
                      n510 = Set File Position(refnum=w2654, from (0:start)=enum16{"start", "end", "current"}."end", error in=w2655) -> (refnum out=w2652:refnum<file>, error out=w2651:errorcluster)  [unwired: 1 in]
                      n511 = Write to Text File(file (use dialog)=w2652, text=w2648, error in=w2651) -> (refnum out=w2656:refnum<file>, error out=w2657:errorcluster)  [unwired: 2 out]
                      n512 = Close File(refnum=w2656, error in=w2657) -> (path=w2647:path, error out=w2649:errorcluster)
                      n513 = call <vilib>:"Simple Error Handler.vi"("error in (no error)"=w2649) -> ("error out"=w2646:errorcluster)  [unwired: 1 in, 7 out]
                    }
                    frame #1 {
                      n514 = Read from Text File(file (use dialog)=w2665, count=-1 ("Count  3"), error in=w2664) -> (refnum out=w2666:refnum<file>, text=w2670:string, error out=w2667:errorcluster)  [unwired: 1 in, 1 out]
                      n515 = local write "String_cinetica"(w2670) -> ()
                      n516 = Close File(refnum=w2666, error in=w2667) -> (error out=w2668:errorcluster)  [unwired: 1 out]
                      n517 = call <vilib>:"Simple Error Handler.vi"("error in (no error)"=w2668) -> ()  [unwired: 1 in, 8 out]
                    }
                    frame #2 {
                      n518 = local write "P T  index"(0 ("P T  index")) -> ()
                      n519 = local write "T subarray 2"(dbl[] [0.0, 1.0] ("subarray")) -> ()
                      n520 = local write "P subarray"(dbl[] [0.0, 1.0] ("subarray")) -> ()
                    }
                  }
                }
              }
              n521 = Greater Or Equal?(x=w2630, y="seconds") -> (x >= y?=w2631:bool)
              n522 = feedback-in #3(w2631) -> ()
            }
          }
          n523 = property on="S#01" class="DigNum (strict)"() -> ("Value"=w2537:dbl)  [unwired: 2 in, 2 out]
          n524 = case shown="True" w2538 {
            tunnel: w2537 -> [_ w2572]
            frame False {
            }
            frame True {
              n525 = flat-sequence {
                tunnel: w2572 -> [w2615]
                tunnel: [w2614] -> w2571
                frame #0 {
                  n526 = property on="Boolean 4" class="Bool (strict)"() -> ("Value"=w2596:bool)  [unwired: 2 in, 2 out]
                  n527 = case shown="True" w2596 {
                    frame False {
                    }
                    frame True {
                      n528 = local write "PCh1 2"(dbl[] [] ("PCh1")) -> ()
                      n529 = local write "tempo carga 2"(dbl[] [] ("tempo carga")) -> ()
                      n530 = local write "output array 3"(u32[] [] ("output array 2")) -> ()
                    }
                  }
                }
                frame #1 {
                  n531 = Tick Count (ms)() -> (millisecond timer value=w2626:u32)
                  n532 = property on="output array 3" class="Arr (strict)"() -> ("Value"=w2627:u32[])  [unwired: 2 in, 2 out]
                  n533 = Build Array(w2626) -> (w2620:u32[])
                  n534 = Insert Into Array(array=w2627, new element=w2620) -> (w2621:u32[])  [unwired: 1 in]
                  "output array 3" <- w2621
                  n535 = Array Max & Min(array=w2621) -> (max value=w2625:u32, min value=w2624:u32)  [unwired: 2 out]
                  n536 = Subtract(x=w2625, y=w2624) -> (x-y=w2622:u32)
                  n537 = Divide(x=w2622, y=1000.0) -> (x/y=w2613:dbl)
                  n538 = property on="t-sivert01(s)" class="DigNum (strict)"() -> ("Value"=w2601:dbl)  [unwired: 2 in, 2 out]
                  n539 = Build Array(w2615) -> (w2616:dbl[])
                  n540 = Greater?(x=w2613, y=w2601) -> (0:w2614:bool)
                  n541 = Build Array(w2613) -> (w2619:dbl[])
                  n542 = property on="tempo carga 2" class="Arr (strict)"() -> ("Value"=w2618:dbl[])  [unwired: 2 in, 2 out]
                  n543 = property on="PCh1 2" class="Arr (strict)"() -> ("Value"=w2617:dbl[])  [unwired: 2 in, 2 out]
                  n544 = Insert Into Array(array=w2618, new element=w2619) -> (w2606:dbl[])  [unwired: 1 in]
                  "tempo carga 2" <- w2606
                  n545 = Insert Into Array(array=w2617, new element=w2616) -> (w2609:dbl[])  [unwired: 1 in]
                  "PCh1 2" <- w2609
                  n546 = call <vilib>:"General Polynomial Fit.vi"("Y"=w2609, "polynomial order"=0, "X"=w2606) -> ("Best Polynomial Fit"=w2605:dbl[], "Polynomial Coefficients"=w2604:dbl[])  [unwired: 9 in, 2 out]
                  n547 = call <vilib>:"Linear Fit.vi"("Y"=w2609, "X"=w2606) -> ("Best Linear Fit"=w2610:dbl[], "slope"=w2602:dbl)  [unwired: 9 in, 3 out]
                  n548 = local write "dP/dt (bar/s)"(w2602) -> ()
                  n549 = Index Array(array=w2604) -> (element=w2603:dbl)  [unwired: 1 in]
                  n550 = Bundle("Value"=w2606, "Best Polynomial Fit"=w2605) -> (w2607:T5)  [unwired: 1 in]
                  n551 = Bundle("Value"=w2606, "Best Linear Fit"=w2610) -> (w2611:cluster{"Value":dbl[], "Best Linear Fit":dbl[]})  [unwired: 1 in]
                  n552 = Bundle("Value"=w2606, "Value"=w2609) -> (w2612:cluster{"Value":dbl[], "Value":dbl[]})  [unwired: 1 in]
                  n553 = local write "P(bar) FIT"(w2603) -> ()
                  n554 = Build Array(w2612, w2611, w2607) -> (w2600:T6)
                  n555 = property on="XY Graph 2" class="XYGraph (strict)"("Value"=w2600) -> ()  [unwired: 2 in, 2 out]
                }
              }
              n556 = property on="T fit" class="DigNum (strict)"() -> ("Value"=w2570:dbl)  [unwired: 2 in, 2 out]
              n557 = local write "T(º) FIT"(w2570) -> ()
              n558 = local write "Boolean 4"(w2571) -> ()
              n559 = case shown="True" w2571 {
                frame False {
                }
                frame True {
                  w2580 = "\t"
                  w2578 = i16 6 ("precision (6)")
                  n560 = property on="P(bar) FIT" class="DigNum (strict)"() -> ("Value"=w2576:dbl)  [unwired: 2 in, 2 out]
                  n561 = property on="T fit" class="DigNum (strict)"() -> ("Value"=w2574:dbl)  [unwired: 2 in, 2 out]
                  n562 = property on="termopar K" class="DigNum (strict)"() -> ("Value"=w2573:dbl)  [unwired: 2 in, 2 out]
                  n563 = Number To Engineering String(2:w2578, 4:w2576) -> (0:w2582:string)  [unwired: 2 in]
                  n564 = Number To Engineering String(2:w2578, 4:w2574) -> (0:w2581:string)  [unwired: 2 in]
                  n565 = Number To Engineering String(2:w2578, 4:w2573) -> (0:w2579:string)  [unwired: 2 in]
                  n566 = property on="path 2" class="Path"() -> ("Value"=w2575:path)  [unwired: 2 in, 2 out]
                  n567 = Get Date/Time String(date format (0)=enum16{"short", "long", "abbreviated"}."short", want seconds? (F)=TRUE) -> (date string=w2584:string, time string=w2583:string)  [unwired: 1 in]
                  n568 = Open/Create/Replace File(file path (use dialog)=w2575) -> (refnum out=w2592:refnum<file>, error out=w2593:errorcluster)  [unwired: 3 in, 3 out]
                  n569 = Concatenate Strings(w2584, w2580, w2583, w2580, w2582, w2580, w2581, w2580, w2579, "\r\n") -> (w2587:string)
                  n570 = Set File Position(refnum=w2592, from (0:start)=enum16{"start", "end", "current"}."end", error in=w2593) -> (refnum out=w2590:refnum<file>, error out=w2589:errorcluster)  [unwired: 1 in]
                  n571 = Write to Text File(file (use dialog)=w2590, text=w2587, error in=w2589) -> (refnum out=w2594:refnum<file>, error out=w2595:errorcluster)  [unwired: 1 in, 1 out]
                  n572 = Close File(refnum=w2594, error in=w2595) -> (error out=w2588:errorcluster)  [unwired: 1 out]
                  n573 = call <vilib>:"Simple Error Handler.vi"("error in (no error)"=w2588) -> ()  [unwired: 1 in, 8 out]
                }
              }
            }
          }
          n574 = property on="correçao\n termopar" class="DigNum (strict)"() -> ("Value"=w2535:dbl)  [unwired: 2 in, 2 out]
          n575 = property on="correção\n NTC" class="DigNum (strict)"() -> ("Value"=w2548:dbl)  [unwired: 2 in, 2 out]
          n576 = call "Read P T.vi"("correção NTC"=w2548, "correçao termopar"=w2535) -> ("Sievert01"=w2541:dbl, "mean H2 sensor"=→"mean H2 sensor (V)":dbl, "termopar K"=w2546:dbl, "output NTC"=w2545:dbl, "P Set 2 Output 2"=w2544:dbl)  [unwired: 2 in, 7 out]
          "termopar K" <- w2546
          "output NTC" <- w2545
          n577 = Multiply(x=w2541, y=10.0) -> (x*y=w2542:dbl)
          "S#01" <- w2542
          n578 = Multiply(x=w2544, y=10.0) -> (x*y=w2552:dbl)
          n579 = local write "Vol Ref"(w2552) -> ()
          n580 = Merge Signals(w2552, w2545, w2546, w2542) -> (→"P-manual":dynamicdata)
          n581 = stacked-sequence {
            tunnel: w2552 -> [w2698 _]
            tunnel: w2545 -> [w2677 _]
            frame #0 {
              w2676 = 2 ("y")
              n582 = property on="P subarray" class="Arr (strict)"() -> ("Value"=w2700:dbl[])  [unwired: 2 in, 2 out]
              n583 = property on="P T  index" class="DigNum (strict)"() -> ("Value"=w2678:i32)  [unwired: 2 in, 2 out]
              n584 = property on="T subarray 2" class="Arr (strict)"() -> ("Value"=w2687:dbl[])  [unwired: 2 in, 2 out]
              n585 = Replace Array Subset(array=w2700, new element=w2698, index=w2678) -> (w2696:dbl[])
              n586 = Replace Array Subset(array=w2687, new element=w2677, index=w2678) -> (w2684:dbl[])
              n587 = call-poly <vilib>:"Array To Matrix.vi"("Real 1D Array"=w2696) -> ("Real Matrix (Column Vector)"=w2703:T7)
              n588 = call-poly <vilib>:"Array To Matrix.vi"("Real 1D Array"=w2684) -> ("Real Matrix (Column Vector)"=w2690:T7)
              n589 = Matrix Size(0:w2703) -> (1:w2702:i32, 2:w2701:i32)
              n590 = Matrix Size(0:w2690) -> (1:w2689:i32, 2:w2688:i32)
              n591 = Increment(x=w2702) -> (x+1=w2691:i32)
              n592 = Increment(x=w2689) -> (x+1=w2679:i32)
              n593 = Resize Matrix(1:w2701, 2:w2691, 4:w2703) -> (0:w2699:T7)
              n594 = Resize Matrix(1:w2688, 2:w2679, 4:w2690) -> (0:w2686:T7)
              n595 = call-poly <vilib>:"Matrix To Array.vi"("Real Matrix"=w2699) -> ("Real 2D Array"=w2694:dbl[][])
              n596 = call-poly <vilib>:"Matrix To Array.vi"("Real Matrix"=w2686) -> ("Real 2D Array"=w2682:dbl[][])
              n597 = Subtract(x=w2691, y=w2676) -> (x-y=w2692:i32)
              n598 = Subtract(x=w2679, y=w2676) -> (x-y=w2680:i32)
              n599 = Reshape Array(w2694, w2691) -> (w2693:dbl[])
              n600 = Reshape Array(w2682, w2679) -> (w2681:dbl[])
              n601 = local write "P subarray"(w2693) -> ()
              n602 = Reshape Array(w2693, w2692) -> (w2695:dbl[])
              n603 = local write "T subarray 2"(w2681) -> ()
              n604 = Reshape Array(w2681, w2680) -> (w2683:dbl[])
              n605 = call <vilib>:"Mean.vi"("X"=w2695) -> ("mean"=→"P cinetica mean":dbl)  [unwired: 1 out]
              n606 = call <vilib>:"Mean.vi"("X"=w2683) -> ("mean"=→"T cinetica mean 2":dbl)  [unwired: 1 out]
            }
            frame #1 {
              n607 = property on="P T  index" class="DigNum (strict)"() -> ("Value"=w2705:i32)  [unwired: 2 in, 2 out]
              n608 = Increment(x=w2705) -> (x+1=w2704:i32)
              n609 = local write "P T  index"(w2704) -> ()
            }
          }
          "N" <- w2557
        }
        n610 = call <vilib>:"Linear Fit.vi"("Y"=w1848, "X"=w1852) -> ("Best Linear Fit"=w1850:dbl[], "slope"=→"bar/N":dbl)  [unwired: 9 in, 3 out]
        n611 = Bundle(w1852, w1848) -> (w1855:cluster{i32[], dbl[]})  [unwired: 1 in]
        n612 = call <vilib>:"General Polynomial Fit.vi"("Y"=w1857, "polynomial order"=w1873, "X"=w1852) -> ("Best Polynomial Fit"=w1869:dbl[], "Polynomial Coefficients"=w1870:dbl[])  [unwired: 9 in, 2 out]
        "Polynomial Coefficients 2" <- w1870
        n613 = call <vilib>:"General Polynomial Fit.vi"("Y"=w1848, "polynomial order"=w1873, "X"=w1866) -> ("Best Polynomial Fit"=w1851:dbl[], "Polynomial Coefficients"=w1864:dbl[])  [unwired: 9 in, 2 out]
        "Polynomial Coefficients" <- w1864
        n614 = Bundle(w1852, "Best Polynomial Fit"=w1851) -> (w1854:cluster{i32[], "Best Polynomial Fit":dbl[]})  [unwired: 1 in]
        n615 = Build Array(w1857, w1869) -> (→"Linear Model Graph 2":dbl[][])
        n616 = Index Array(array=w1864, index=0) -> (element=→"p fit":dbl)
        n617 = Index Array(array=w1870, index=0) -> (element=→"T fit":dbl)
        n618 = Build Array(w1848, w1851, w1850) -> (→"Linear Model Graph":dbl[][])
        n619 = Bundle(w1852, "Best Linear Fit"=w1850) -> (w1853:cluster{i32[], "Best Linear Fit":dbl[]})  [unwired: 1 in]
        n620 = Build Array(w1855, w1854, w1853) -> ()  [unwired: 1 out]
      }
    }
    n621 = case shown="True" "Ligar RLC" {
      tunnel: w47 -> [_ w176]
      frame False {
      }
      frame True {
        w184 = "\t"
        w205 = "\t"
        w188 = "\r"
        w181 = "\r\n"
        w221 = "\r"
        w211 = "\t"
        n622 = Strip Path(path=w176) -> (stripped path=w177:path, name=w180:string)
        n623 = Get Date/Time String(date format (0)=enum16{"short", "long", "abbreviated"}."short", want seconds? (F)=TRUE) -> (date string=w228:string, time string=w227:string)  [unwired: 1 in]
        n624 = Concatenate Strings("SET" ("Nota 4"), w184, "DATE" ("Nota 4"), w184, "TIME" ("Nota 4"), w184, w205, "P (BAR)" ("Nota 4"), w205, "T (ºC)" ("Nota 4"), w205, "C-50-L" ("Nota 4"), w205, "C-50-N" ("Nota 4"), w205, "C-100-L" ("Nota 4"), w205, "C-100-N" ("Nota 4"), w205, "C-1K-L" ("Nota 4"), w205, "C-1K-N" ("Nota 4"), w205, "C-10K-L" ("Nota 4"), w205, "C-10K-N" ("Nota 4"), w205, "Z-50-L" ("Nota 4"), w205, "Z-50-N" ("Nota 4"), w205, "Z-100-L" ("Nota 4"), w205, "Z-100-N" ("Nota 4"), w205, "Z-1K-L" ("Nota 4"), w205, "Z-1K-N" ("Nota 4"), w205, "Z-10K-L" ("Nota 4"), w205, "Z-10K-N" ("Nota 4")) -> (w189:string)
        n625 = Concatenate Strings(w228, w211, w227) -> (w223:string)
        n626 = Concatenate Strings(w180, "_RLC_CDH completo" ("string")) -> (w178:string)
        n627 = Concatenate Strings("Sievert RLC - CDH:" ("string"), w211, w181, w181) -> (w209:string)
        n628 = Concatenate Strings("Data Table" ("string"), w188, "==========" ("string"), w188, w189, w188) -> (w222:string)
        n629 = File Dialog(6:".txt" ("pattern label"), 9:w178, 11:w177) -> (0:w219:errorcluster, 3:w220:path)  [unwired: 2 in, 4 out]
        n630 = Open/Create/Replace File(file path (use dialog)=w220, error in=w219, operation (0:open)=T3."replace or create with confirmation", access (0:read/write)=enum16{"read/write", "read-only", "write-only"}."read/write") -> (refnum out=w216:refnum<file>, error out=w215:errorcluster)  [unwired: 3 out]
        n631 = Concatenate Strings(w223, w221, w221, w209, w221, w221, "Nota 01: MEDIDAS COM RLC 300 - MULTILEITURA" ("Nota 4"), w221, w221, w222) -> (w226:string)
        n632 = Write to Text File(file (use dialog)=w216, text=w226, error in=w215) -> (refnum out=w214:refnum<file>, error out=w212:errorcluster)  [unwired: 1 in, 1 out]
        n633 = Close File(refnum=w214, error in=w212) -> (path=w208:path)  [unwired: 1 out]
        n634 = local write "path RLC_completo"(w208) -> ()
      }
    }
    n635 = case shown="True" "Ligar RLC" {
      tunnel: w47 -> [_ w119]
      frame False {
      }
      frame True {
        w128 = "\t"
        w149 = "\t"
        w132 = "\r"
        w125 = "\r\n"
        w164 = "\r"
        w154 = "\t"
        n636 = Strip Path(path=w119) -> (stripped path=w121:path, name=w124:string)
        n637 = Get Date/Time String(date format (0)=enum16{"short", "long", "abbreviated"}."short", want seconds? (F)=TRUE) -> (date string=w171:string, time string=w170:string)  [unwired: 1 in]
        n638 = Concatenate Strings("SET" ("Nota 4"), w128, "DATE" ("Nota 4"), w128, "TIME" ("Nota 4"), w128, w149, "P (BAR)" ("Nota 4"), w149, "T (ºC)" ("Nota 4"), w149, "C-50-L" ("Nota 4"), w149, "C-50-N" ("Nota 4"), w149, "C-100-L" ("Nota 4"), w149, "C-100-N" ("Nota 4"), w149, "C-1K-L" ("Nota 4"), w149, "C-1K-N" ("Nota 4"), w149, "C-10K-L" ("Nota 4"), w149, "C-10K-N" ("Nota 4"), w149, "Z-50-L" ("Nota 4"), w149, "Z-50-N" ("Nota 4"), w149, "Z-100-L" ("Nota 4"), w149, "Z-100-N" ("Nota 4"), w149, "Z-1K-L" ("Nota 4"), w149, "Z-1K-N" ("Nota 4"), w149, "Z-10K-L" ("Nota 4"), w149, "Z-10K-N" ("Nota 4")) -> (w133:string)
        n639 = Concatenate Strings(w171, w154, w170) -> (w166:string)
        n640 = Concatenate Strings(w124, "_RLC_CDH mean" ("string")) -> (w122:string)
        n641 = Concatenate Strings("Sievert RLC - CDH:" ("string"), w154, w125, w125) -> (w152:string)
        n642 = Concatenate Strings("Data Table" ("string"), w132, "==========" ("string"), w132, w133, w132) -> (w165:string)
        n643 = File Dialog(6:".txt" ("pattern label"), 9:w122, 11:w121) -> (0:w162:errorcluster, 3:w163:path)  [unwired: 2 in, 4 out]
        n644 = Open/Create/Replace File(file path (use dialog)=w163, error in=w162, operation (0:open)=T3."replace or create with confirmation", access (0:read/write)=enum16{"read/write", "read-only", "write-only"}."read/write") -> (refnum out=w159:refnum<file>, error out=w158:errorcluster)  [unwired: 3 out]
        n645 = Concatenate Strings(w166, w164, w164, w152, w164, w164, "Nota 01: MEDIDAS COM RLC 300 - MULTILEITURA" ("Nota 4"), w164, w164, w165) -> (w169:string)
        n646 = Write to Text File(file (use dialog)=w159, text=w169, error in=w158) -> (refnum out=w157:refnum<file>, error out=w155:errorcluster)  [unwired: 1 in, 1 out]
        n647 = Close File(refnum=w157, error in=w155) -> (path=w120:path)  [unwired: 1 out]
        n648 = local write "path RLC_mean"(w120) -> ()
      }
    }
    n649 = case shown="False" "Auto Ctrl" {
      tunnel: [TRUE ("Auto Ctrl") FALSE ("Auto Ctrl")] -> w53
      frame False {
      }
      frame True {
      }
    }
    n650 = case shown="True" "Save S#1" {
      frame False {
      }
      frame True {
        n651 = call "File_data_cineticaS1.vi"("Nota 01"="Nota 01", "Sample name"="Sample name 2", "File name"="File name 2") -> ("path"=→"path 2":path)  [unwired: 8 in]
      }
    }
    n652 = Exclusive Or(1:w50, 2:"stop") -> (0:w52:bool)
    n653 = case shown="True" "Close RLC 2" {
      tunnel: w40 -> [_ w174]
      frame False {
      }
      frame True {
        n654 = call "RLC_close.vi"("Path"=w174) -> ("String"=w175:string)  [unwired: 10 in]
        n655 = local write "RLC300 - digimess"(w175) -> ()
      }
    }
    n656 = case shown="True" "Open Button 2" {
      frame False {
      }
      frame True {
        n657 = property on="Sample name" class="Str"() -> ("Value"=w1827:string)  [unwired: 2 in, 2 out]
        n658 = property on="File name" class="Str"() -> ("Value"=w1828:string)  [unwired: 2 in, 2 out]
        n659 = property on="Nota" class="Str"() -> ("Value"=w1826:string)  [unwired: 2 in, 2 out]
        n660 = call "Open file.vi"("Nota 01"=w1826, "Sample name"=w1827, "File name"=w1828) -> ("path open old"=w1825:path)  [unwired: 8 in]
        n661 = local write "path"(w1825) -> ()
      }
    }
    n662 = case shown="True" "Refresh Button 2" {
      frame False {
      }
      frame True {
        n663 = property on="Waveform Chart" class="WFChart (strict)"("History Data"=dynamicdata[] []) -> ()  [unwired: 2 in, 2 out]
      }
    }
    n664 = case shown="True" "Refresh Button 3" {
      frame False {
      }
      frame True {
        n665 = property on="Waveform Chart 2" class="WFChart (strict)"("History Data"=dynamicdata[] []) -> ()  [unwired: 2 in, 2 out]
      }
    }
    n666 = case shown="True" "Open Button" {
      frame False {
      }
      frame True {
        n667 = flat-sequence {
          tunnel: ["Sample name"] -> w1831
          tunnel: ["Nota"] -> w1830
          tunnel: [w1833] -> w1829
          tunnel: w1831 -> [w1846]
          tunnel: w1830 -> [w1845]
          tunnel: w1829 -> [w1840]
          frame #0 {
            n668 = local write "Count SET"(0 ("Count SET")) -> ()
            n669 = local write "Set atual"(0 ("Count  3")) -> ()
            n670 = call "File_data_new.vi"("Nota 01"="Nota", "Sample name"="Sample name", "File name"="File name") -> ("path"=w1833:path)  [unwired: 8 in]
            "path" <- w1833
          }
          frame #1 {
            w1841 = FALSE
            n671 = Strip Path(path=w1840) -> (stripped path=w1839:path, name=w1838:string)
            n672 = local write "Pf2"(w1841) -> ()
            n673 = local write "ZPit"(w1841) -> ()
            n674 = local write "Pit"(w1841) -> ()
            n675 = local write "ZPf2"(w1841) -> ()
            n676 = local write "T"(w1841) -> ()
            n677 = Concatenate Strings(w1838, "_cinetica" ("string")) -> (w1843:string)
            n678 = call "File_data_cinetica.vi"("path in"=w1839, "Nota 01"=w1845, "Sample name"=w1846, "File name"=w1843) -> ("path"=→"path 2_cinetica":path)  [unwired: 7 in]
          }
        }
      }
    }
    n679 = local write "Manual Ctrl"(w53) -> ()
    n680 = case shown="True" "Auto Ctrl" {
      tunnel: w40 -> [_ w237]
      tunnel: "RLC on/off" -> [_ w236]
      tunnel: [_ w235] -> w43
      frame False {
      }
      frame True {
        n681 = local write "P T  index 2"(0 ("P T  index")) -> ()
        n682 = local write "time subarray"(dbl[] [0.0, 1.0] ("subarray")) -> ()
        n683 = for {
          N: "N fit" -> [w266]
          tunnel: w237 -> [w257]
          tunnel: w236 -> [w256]
          tunnel: [w255] -> w235
          i -> [w268]
          w272 = 0 ("polynomial order")
          w263 = 0 ("polynomial order")
          n684 = case shown="True" "clear" {
            frame False {
            }
            frame True {
              n685 = property on="Linear P" class="XYGraph (strict)"("Value"=T2 [] ("Linear P")) -> ()  [unwired: 2 in, 2 out]
              n686 = property on="Linear T" class="XYGraph (strict)"("Value"=T2 [] ("Linear T")) -> ()  [unwired: 2 in, 2 out]
              n687 = property on="Automatico" class="WFChart (strict)"("History Data"=dynamicdata[] []) -> ()  [unwired: 2 in, 2 out]
              n688 = property on="Automatico 2" class="WFChart (strict)"("History Data"=dynamicdata[] []) -> ()  [unwired: 2 in, 2 out]
            }
          }
          n689 = property on="path 2_cinetica" class="Path"() -> ("Value"=w260:path)  [unwired: 2 in, 2 out]
          n690 = Increment(x=w268) -> (x+1=w267:i32)
          n691 = call "Read P T.vi"("correção NTC"="correção\n NTC", "correçao termopar"="correçao\n termopar") -> ("Sievert01"=w249:dbl, "mean H2 sensor"=w252:dbl, "termopar K"=w247:dbl, "output NTC"=w246:dbl, "P Set 2 Output 2"=w251:dbl)  [unwired: 2 in, 7 out]
          "termopar K 2" <- w247
          "mean H2 sensor" <- w252
          n692 = Equal?(x=w267, y=w266) -> (x = y?=w269:bool)
          "x = y?" <- w269
          n693 = Merge Signals(w252) -> (→"Automatico 2":dynamicdata)
          n694 = Multiply(x=w249, y=10.0) -> (x*y=w245:dbl)
          "S#1_auto" <- w245
          n695 = Multiply(x=w251, y=10.0) -> (x*y=w262:dbl)
          n696 = local write "Vol Ref 3"(w262) -> ()
          n697 = case shown="True" "Save - Sievert 01" {
            tunnel: w245 -> [_ w308]
            frame False {
            }
            frame True {
              n698 = flat-sequence {
                tunnel: w308 -> [w351]
                tunnel: [w349] -> w307
                frame #0 {
                  n699 = property on="Boolean 4" class="Bool (strict)"() -> ("Value"=w332:bool)  [unwired: 2 in, 2 out]
                  n700 = case shown="True" w332 {
                    frame False {
                    }
                    frame True {
                      n701 = local write "PCh1"(dbl[] [] ("PCh1")) -> ()
                      n702 = local write "tempo carga"(dbl[] [] ("tempo carga")) -> ()
                      n703 = local write "output array 2"(u32[] [] ("output array 2")) -> ()
                    }
                  }
                }
                frame #1 {
                  n704 = property on="PCh1" class="Arr (strict)"() -> ("Value"=w353:dbl[])  [unwired: 2 in, 2 out]
                  n705 = Build Array(w351) -> (w352:dbl[])
                  n706 = Tick Count (ms)() -> (millisecond timer value=w362:u32)
                  n707 = Insert Into Array(array=w353, new element=w352) -> (w342:dbl[])  [unwired: 1 in]
                  "PCh1" <- w342
                  n708 = Build Array(w362) -> (w356:u32[])
                  n709 = property on="tempo carga" class="Arr (strict)"() -> ("Value"=w354:dbl[])  [unwired: 2 in, 2 out]
                  n710 = property on="output array 2" class="Arr (strict)"() -> ("Value"=w363:u32[])  [unwired: 2 in, 2 out]
                  n711 = Insert Into Array(array=w363, new element=w356) -> (w357:u32[])  [unwired: 1 in]
                  "output array 2" <- w357
                  n712 = Array Max & Min(array=w357) -> (max value=w361:u32, min value=w360:u32)  [unwired: 2 out]
                  n713 = Subtract(x=w361, y=w360) -> (x-y=w358:u32)
                  n714 = Divide(x=w358, y=1000.0) -> (x/y=w348:dbl)
                  n715 = Greater?(x=w348, y="t-sivert01(s)") -> (0:w349:bool)
                  n716 = Build Array(w348) -> (w355:dbl[])
                  n717 = Insert Into Array(array=w354, new element=w355) -> (w339:dbl[])  [unwired: 1 in]
                  "tempo carga" <- w339
                  n718 = call <vilib>:"General Polynomial Fit.vi"("Y"=w342, "polynomial order"=0, "X"=w339) -> ("Best Polynomial Fit"=w338:dbl[], "Polynomial Coefficients"=w337:dbl[])  [unwired: 9 in, 2 out]
                  n719 = Bundle("Value"=w339, "Value"=w342) -> (w346:cluster{"Value":dbl[], "Value":dbl[]})  [unwired: 1 in]
                  n720 = call <vilib>:"Linear Fit.vi"("Y"=w342, "X"=w339) -> ("Best Linear Fit"=w343:dbl[], "slope"=→"dP/dt (bar/s)":dbl)  [unwired: 9 in, 3 out]
                  n721 = Index Array(array=w337) -> (element=→"P(bar) FIT":dbl)  [unwired: 1 in]
                  n722 = Bundle("Value"=w339, "Best Polynomial Fit"=w338) -> (w340:T5)  [unwired: 1 in]
                  n723 = Bundle("Value"=w339, "Best Linear Fit"=w343) -> (w345:cluster{"Value":dbl[], "Best Linear Fit":dbl[]})  [unwired: 1 in]
                  n724 = Build Array(w346, w345, w340) -> (→"XY Graph 2":T6)
                }
              }
              n725 = property on="T fit" class="DigNum (strict)"() -> ("Value"=→"T(º) FIT":dbl)  [unwired: 2 in, 2 out]
              n726 = case shown="True" w307 {
                frame False {
                }
                frame True {
                  w314 = "\t"
                  w312 = i16 6 ("precision (6)")
                  n727 = property on="T fit" class="DigNum (strict)"() -> ("Value"=w315:dbl)  [unwired: 2 in, 2 out]
                  n728 = property on="path 2" class="Path"() -> ("Value"=w309:path)  [unwired: 2 in, 2 out]
                  n729 = property on="P(bar) FIT" class="DigNum (strict)"() -> ("Value"=w323:dbl)  [unwired: 2 in, 2 out]
                  n730 = Number To Engineering String(2:w312, 4:w323) -> (0:w317:string)  [unwired: 2 in]
                  n731 = Number To Engineering String(2:w312, 4:w315) -> (0:w316:string)  [unwired: 2 in]
                  n732 = Open/Create/Replace File(file path (use dialog)=w309) -> (refnum out=w328:refnum<file>, error out=w329:errorcluster)  [unwired: 3 in, 3 out]
                  n733 = Get Date/Time String(date format (0)=enum16{"short", "long", "abbreviated"}."short", want seconds? (F)=TRUE) -> (date string=w319:string, time string=w318:string)  [unwired: 1 in]
                  n734 = property on="termopar K 2" class="DigNum (strict)"() -> ("Value"=w310:dbl)  [unwired: 2 in, 2 out]
                  n735 = Number To Engineering String(2:w312, 4:w310) -> (0:w313:string)  [unwired: 2 in]
                  n736 = Set File Position(refnum=w328, from (0:start)=enum16{"start", "end", "current"}."end", error in=w329) -> (refnum out=w326:refnum<file>, error out=w325:errorcluster)  [unwired: 1 in]
                  n737 = Concatenate Strings(w319, w314, w318, w314, w317, w314, w316, w314, w313, "\r\n") -> (w322:string)
                  n738 = Write to Text File(file (use dialog)=w326, text=w322, error in=w325) -> (refnum out=w330:refnum<file>, error out=w331:errorcluster)  [unwired: 1 in, 1 out]
                  n739 = Close File(refnum=w330, error in=w331) -> (error out=w324:errorcluster)  [unwired: 1 out]
                  n740 = call <vilib>:"Simple Error Handler.vi"("error in (no error)"=w324) -> ()  [unwired: 1 in, 8 out]
                }
              }
              "Boolean 4" <- w307
            }
          }
          n741 = call "Elapsed Time2"("Reset"=w269) -> ("Elapsed Time (s)"=w283:dbl)  [unwired: 11 in, 7 out]
          "Time (sec)" <- w283
          n742 = Merge Signals(w262, w246, w247, w245) -> (→"Automatico":dynamicdata)
          n743 = stacked-sequence {
            tunnel: w262 -> [w1813 _]
            tunnel: w246 -> [w1799 _]
            tunnel: [w1780 _] -> w281
            tunnel: [w1796 _] -> w280
            tunnel: w283 -> [w1783 _]
            tunnel: [w1781 _] -> w277
            tunnel: [w1779 _] -> w259
            tunnel: [w1778 _] -> w258
            frame #0 {
              w1782 = 2 ("y")
              n744 = property on="P subarray 2" class="Arr (strict)"() -> ("Value"=w1815:dbl[])  [unwired: 2 in, 2 out]
              n745 = property on="T subarray 3" class="Arr (strict)"() -> ("Value"=w1805:dbl[])  [unwired: 2 in, 2 out]
              n746 = property on="time subarray" class="Arr (strict)"() -> ("Value"=w1792:dbl[])  [unwired: 2 in, 2 out]
              n747 = property on="P T  index 2" class="DigNum (strict)"() -> ("Value"=w1784:i32)  [unwired: 2 in, 2 out]
              n748 = Replace Array Subset(array=w1792, new element=w1783, index=w1784) -> (w1785:dbl[])
              n749 = Replace Array Subset(array=w1815, new element=w1813, index=w1784) -> (w1798:dbl[])
              n750 = Replace Array Subset(array=w1805, new element=w1799, index=w1784) -> (w1797:dbl[])
              n751 = call-poly <vilib>:"Array To Matrix.vi"("Real 1D Array"=w1785) -> ("Real Matrix (Column Vector)"=w1795:T7)
              n752 = call-poly <vilib>:"Array To Matrix.vi"("Real 1D Array"=w1798) -> ("Real Matrix (Column Vector)"=w1818:T7)
              n753 = call-poly <vilib>:"Array To Matrix.vi"("Real 1D Array"=w1797) -> ("Real Matrix (Column Vector)"=w1808:T7)
              n754 = Matrix Size(0:w1795) -> (1:w1794:i32, 2:w1793:i32)
              n755 = Matrix Size(0:w1818) -> (1:w1817:i32, 2:w1816:i32)
              n756 = Matrix Size(0:w1808) -> (1:w1807:i32, 2:w1806:i32)
              n757 = Increment(x=w1794) -> (x+1=w1786:i32)
              n758 = Increment(x=w1817) -> (x+1=w1809:i32)
              n759 = Increment(x=w1807) -> (x+1=w1800:i32)
              n760 = Subtract(x=w1786, y=w1782) -> (x-y=w1787:i32)
              n761 = Subtract(x=w1809, y=w1782) -> (x-y=w1810:i32)
              n762 = Subtract(x=w1800, y=w1782) -> (x-y=w1801:i32)
              n763 = Resize Matrix(1:w1793, 2:w1786, 4:w1795) -> (0:w1791:T7)
              n764 = Resize Matrix(1:w1816, 2:w1809, 4:w1818) -> (0:w1814:T7)
              n765 = Resize Matrix(1:w1806, 2:w1800, 4:w1808) -> (0:w1804:T7)
              n766 = call-poly <vilib>:"Matrix To Array.vi"("Real Matrix"=w1791) -> ("Real 2D Array"=w1789:dbl[][])
              n767 = call-poly <vilib>:"Matrix To Array.vi"("Real Matrix"=w1814) -> ("Real 2D Array"=w1812:dbl[][])
              n768 = call-poly <vilib>:"Matrix To Array.vi"("Real Matrix"=w1804) -> ("Real 2D Array"=w1803:dbl[][])
              n769 = Reshape Array(w1789, w1786) -> (w1788:dbl[])
              n770 = Reshape Array(w1812, w1809) -> (w1811:dbl[])
              n771 = Reshape Array(w1803, w1800) -> (w1802:dbl[])
              n772 = local write "time subarray"(w1788) -> ()
              n773 = local write "P subarray 2"(w1811) -> ()
              n774 = local write "T subarray 3"(w1802) -> ()
              n775 = Reshape Array(w1788, w1787) -> (w1781:dbl[])
              n776 = Reshape Array(w1811, w1810) -> (w1780:dbl[])
              n777 = Reshape Array(w1802, w1801) -> (w1796:dbl[])
              n778 = call <vilib>:"Mean.vi"("X"=w1781) -> ("mean"=→"Time cinetica":dbl)  [unwired: 1 out]
              n779 = call <vilib>:"Mean.vi"("X"=w1780) -> ("mean"=w1779:dbl)  [unwired: 1 out]
              "P cinetica mean 2" <- w1779
              n780 = call <vilib>:"Mean.vi"("X"=w1796) -> ("mean"=w1778:dbl)  [unwired: 1 out]
              "T cinetica mean 3" <- w1778
            }
            frame #1 {
              n781 = property on="P T  index 2" class="DigNum (strict)"() -> ("Value"=w1820:i32)  [unwired: 2 in, 2 out]
              n782 = Increment(x=w1820) -> (x+1=w1819:i32)
              n783 = local write "P T  index 2"(w1819) -> ()
            }
          }
          n784 = To Time Stamp(1:w283) -> (0:→"time stamp":timestamp)
          n785 = call <vilib>:"Linear Fit.vi"("Y"=w280, "X"=w277) -> ("Best Linear Fit"=w289:dbl[])  [unwired: 9 in, 4 out]
          n786 = Bundle("Real 2D Array"=w277, "Real 2D Array"=w280) -> (w287:T8)  [unwired: 1 in]
          n787 = Bundle("Real 2D Array"=w277, "Real 2D Array"=w281) -> (w286:T8)  [unwired: 1 in]
          n788 = call <vilib>:"General Polynomial Fit.vi"("Y"=w280, "polynomial order"=w263, "X"=w277) -> ("Best Polynomial Fit"=w278:dbl[], "Polynomial Coefficients"=w273:dbl[])  [unwired: 9 in, 2 out]
          n789 = call <vilib>:"General Polynomial Fit.vi"("Y"=w281, "polynomial order"=w263, "X"=w277) -> ("Best Polynomial Fit"=w279:dbl[], "Polynomial Coefficients"=w274:dbl[])  [unwired: 9 in, 2 out]
          n790 = call <vilib>:"Linear Fit.vi"("Y"=w281, "X"=w277) -> ("Best Linear Fit"=w284:dbl[], "slope"=w264:dbl)  [unwired: 9 in, 3 out]
          "bar/s" <- w264
          n791 = property on="path" class="Path"() -> ("Value"=w261:path)  [unwired: 2 in, 2 out]
          n792 = case shown="True" "Play Button" {
            tunnel: w261 -> [_ w372]
            tunnel: w262 -> [_ w371]
            tunnel: w260 -> [_ w370]
            tunnel: w259 -> [_ w369]
            tunnel: w258 -> [_ w368]
            tunnel: w257 -> [_ w367]
            tunnel: w256 -> [_ w366]
            tunnel: [_ w365] -> w255
            tunnel: w247 -> [_ w364]
            frame False {
            }
            frame True {
              n793 = case shown="7" "Estagio auto" {
                tunnel: w372 -> [_ _ _ w464 _ _ w617 _ w779 _ _ w1619 w1688]
                tunnel: w371 -> [_ w438 _ _ w513 w564 _ _ _ w1537 _ _ _]
                tunnel: w370 -> [_ _ _ _ _ _ _ w659 _ _ _ _ _]
                tunnel: w369 -> [_ _ _ _ _ _ _ w658 _ _ _ _ _]
                tunnel: w368 -> [_ _ _ _ _ _ _ w657 _ _ _ _ _]
                tunnel: w367 -> [_ _ _ _ _ _ _ _ w758 _ _ _ _]
                tunnel: w366 -> [_ _ _ _ _ _ _ _ w775 _ _ _ _]
                tunnel: [_ _ _ _ _ _ _ _ w757 _ _ _ _] -> w365
                tunnel: w364 -> [_ _ _ _ _ _ _ _ _ _ _ w1615 _]
                frame 0, Default {
                  n794 = stacked-sequence {
                    frame #0 {
                      w374 = FALSE ("Pit")
                      n795 = local write "String"("Verificar e fechar todas as valvulas" ("String")) -> ()
                      "ZPf2 2" <- w374
                      "Pf2 2" <- w374
                      "Pit 2" <- w374
                      "ZPit 2" <- w374
                      "T 2" <- w374
                    }
                    frame #1 {
                      w377 = FALSE ("Boolean 4")
                      w382 = T4 3 items=["no dialog", "OK message", "continue or stop message", "OK message + warnings", "continue/stop + warnings"] ("type of dialog (OK msg:1)")
                      n796 = Wait (ms)(milliseconds to wait=u32 500) -> ()  [unwired: 1 out]
                      n797 = local write "Entrada gás 2"(w377) -> ()
                      n798 = call-poly <vilib>:"DAQmx Create Virtual Channel.vi"("lines"=tag "Dev1/port0/line1") -> ("task out"=w380:refnum<k21>, "error out"=w381:errorcluster)  [unwired: 13 in]
                      n799 = call <vilib>:"DAQmx Start Task.vi"("task/channels in"=w380, "error in"=w381) -> ("task out"=w383:refnum<k21>, "error out"=w384:errorcluster)  [unwired: 12 in]
                      n800 = call-poly <vilib>:"DAQmx Write.vi"("task/channels in"=w383, "data"=w377, "error in"=w384) -> ("task out"=w388:refnum<k21>, "error out"=w385:errorcluster)  [unwired: 10 in, 1 out]
                      n801 = call <vilib>:"DAQmx Stop Task.vi"("task/channels in"=w388, "error in"=w385) -> ("task out"=w387:refnum<k21>, "error out"=w386:errorcluster)  [unwired: 12 in]
                      n802 = call <vilib>:"DAQmx Clear Task.vi"("task in"=w387, "error in"=w386) -> ("error out"=w379:errorcluster)  [unwired: 13 in]
                      n803 = call <vilib>:"Simple Error Handler.vi"("type of dialog (OK msg:1)"=w382, "error in (no error)"=w379) -> ()  [unwired: 3 in, 5 out]
                    }
                    frame #2 {
                      w390 = FALSE ("Boolean 4")
                      w395 = T4 3 items=["no dialog", "OK message", "continue or stop message", "OK message + warnings", "continue/stop + warnings"] ("type of dialog (OK msg:1)")
                      n804 = Wait (ms)(milliseconds to wait=u32 500) -> ()  [unwired: 1 out]
                      n805 = local write "Vácuo 2"(w390) -> ()
                      n806 = call-poly <vilib>:"DAQmx Create Virtual Channel.vi"("lines"=tag "Dev1/port0/line2") -> ("task out"=w393:refnum<k21>, "error out"=w394:errorcluster)  [unwired: 13 in]
                      n807 = call <vilib>:"DAQmx Start Task.vi"("task/channels in"=w393, "error in"=w394) -> ("task out"=w396:refnum<k21>, "error out"=w397:errorcluster)  [unwired: 12 in]
                      n808 = call-poly <vilib>:"DAQmx Write.vi"("task/channels in"=w396, "data"=w390, "error in"=w397) -> ("task out"=w401:refnum<k21>, "error out"=w398:errorcluster)  [unwired: 10 in, 1 out]
                      n809 = call <vilib>:"DAQmx Stop Task.vi"("task/channels in"=w401, "error in"=w398) -> ("task out"=w400:refnum<k21>, "error out"=w399:errorcluster)  [unwired: 12 in]
                      n810 = call <vilib>:"DAQmx Clear Task.vi"("task in"=w400, "error in"=w399) -> ("error out"=w392:errorcluster)  [unwired: 13 in]
                      n811 = call <vilib>:"Simple Error Handler.vi"("type of dialog (OK msg:1)"=w395, "error in (no error)"=w392) -> ()  [unwired: 3 in, 5 out]
                    }
                    frame #3 {
                      w403 = FALSE ("Boolean 4")
                      w408 = T4 3 items=["no dialog", "OK message", "continue or stop message", "OK message + warnings", "continue/stop + warnings"] ("type of dialog (OK msg:1)")
                      n812 = Wait (ms)(milliseconds to wait=u32 500) -> ()  [unwired: 1 out]
                      n813 = local write "Câmara 2"(w403) -> ()
                      n814 = call-poly <vilib>:"DAQmx Create Virtual Channel.vi"("lines"=tag "Dev1/port0/line3") -> ("task out"=w406:refnum<k21>, "error out"=w407:errorcluster)  [unwired: 13 in]
                      n815 = call <vilib>:"DAQmx Start Task.vi"("task/channels in"=w406, "error in"=w407) -> ("task out"=w409:refnum<k21>, "error out"=w410:errorcluster)  [unwired: 12 in]
                      n816 = call-poly <vilib>:"DAQmx Write.vi"("task/channels in"=w409, "data"=w403, "error in"=w410) -> ("task out"=w414:refnum<k21>, "error out"=w411:errorcluster)  [unwired: 10 in, 1 out]
                      n817 = call <vilib>:"DAQmx Stop Task.vi"("task/channels in"=w414, "error in"=w411) -> ("task out"=w413:refnum<k21>, "error out"=w412:errorcluster)  [unwired: 12 in]
                      n818 = call <vilib>:"DAQmx Clear Task.vi"("task in"=w413, "error in"=w412) -> ("error out"=w405:errorcluster)  [unwired: 13 in]
                      n819 = call <vilib>:"Simple Error Handler.vi"("type of dialog (OK msg:1)"=w408, "error in (no error)"=w405) -> ()  [unwired: 3 in, 5 out]
                    }
                    frame #4 {
                      w416 = FALSE ("Boolean 4")
                      w421 = T4 3 items=["no dialog", "OK message", "continue or stop message", "OK message + warnings", "continue/stop + warnings"] ("type of dialog (OK msg:1)")
                      n820 = Wait (ms)(milliseconds to wait=u32 500) -> ()  [unwired: 1 out]
                      n821 = local write "Atm 2"(w416) -> ()
                      n822 = call-poly <vilib>:"DAQmx Create Virtual Channel.vi"("lines"=tag "Dev1/port0/line4") -> ("task out"=w419:refnum<k21>, "error out"=w420:errorcluster)  [unwired: 13 in]
                      n823 = call <vilib>:"DAQmx Start Task.vi"("task/channels in"=w419, "error in"=w420) -> ("task out"=w422:refnum<k21>, "error out"=w423:errorcluster)  [unwired: 12 in]
                      n824 = call-poly <vilib>:"DAQmx Write.vi"("task/channels in"=w422, "data"=w416, "error in"=w423) -> ("task out"=w427:refnum<k21>, "error out"=w424:errorcluster)  [unwired: 10 in, 1 out]
                      n825 = call <vilib>:"DAQmx Stop Task.vi"("task/channels in"=w427, "error in"=w424) -> ("task out"=w426:refnum<k21>, "error out"=w425:errorcluster)  [unwired: 12 in]
                      n826 = call <vilib>:"DAQmx Clear Task.vi"("task in"=w426, "error in"=w425) -> ("error out"=w418:errorcluster)  [unwired: 13 in]
                      n827 = call <vilib>:"Simple Error Handler.vi"("type of dialog (OK msg:1)"=w421, "error in (no error)"=w418) -> ()  [unwired: 3 in, 5 out]
                    }
                    frame #5 {
                      n828 = Wait (ms)(milliseconds to wait=u32 500) -> ()  [unwired: 1 out]
                    }
                    frame #6 {
                      n829 = property on="Read ZPit" class="Bool (strict)"() -> ("Value"=w430:bool)  [unwired: 2 in, 2 out]
                      n830 = case shown="False" w430 {
                        frame False {
                          n831 = local write "Estagio auto"(3 ("Estagio auto")) -> ()
                        }
                        frame True {
                          n832 = local write "Estagio auto"(1 ("Estagio auto")) -> ()
                        }
                      }
                      n833 = local write "N fit"("N fit 2") -> ()
                    }
                  }
                }
                frame 1 {
                  n834 = Greater?(x=w438, y=1.0) -> (0:w437:bool)
                  n835 = case shown="True" w437 {
                    tunnel: [FALSE ("Boolean") TRUE ("Boolean")] -> w434
                    frame False {
                      w450 = TRUE ("Boolean")
                      n836 = local write "Vácuo 2"(w450) -> ()
                      n837 = call "Controle_vacuo.vi"("time (s) to wait vacuo"=u32 5, "Boolean"=w450) -> ("Vacuo"=w451:bool)  [unwired: 9 in]
                      n838 = local write "Vácuo 2"(w451) -> ()
                      n839 = local write "String"("Limpar volume referencia" ("String")) -> ()
                    }
                    frame True {
                      n840 = call "Controle_ATM.vi"("seconds to wait"="ATM wait") -> ("String 2"=w455:string, "Atm"=w454:bool)  [unwired: 9 in]
                      n841 = local write "Atm 2"(w454) -> ()
                      n842 = local write "String"(w455) -> ()
                    }
                  }
                  n843 = for {
                    N: 1 -> [_]
                    tunnel: [w440] -> w435
                    tunnel: w434 -> [w440]
                    n844 = Wait (ms)(milliseconds to wait=u32 500 ("x")) -> ()  [unwired: 1 out]
                  }
                  n845 = case shown="True" w435 {
                    frame False {
                      n846 = local write "Estagio auto"(2 ("Estagio auto")) -> ()
                    }
                    frame True {
                      w445 = TRUE ("Boolean")
                      n847 = local write "Estagio auto"(2 ("Estagio auto")) -> ()
                      n848 = local write "Vácuo 2"(w445) -> ()
                      n849 = call "Controle_vacuo.vi"("time (s) to wait vacuo"=u32 5, "Boolean"=w445) -> ("Vacuo"=w446:bool)  [unwired: 9 in]
                      n850 = local write "Vácuo 2"(w446) -> ()
                      n851 = local write "String"("Limpar volume referencia" ("String")) -> ()
                    }
                  }
                }
                frame 2 {
                  n852 = property on="Contador" class="DigNum (strict)"() -> ("Value"=w459:i32)  [unwired: 2 in, 2 out]
                  n853 = local write "String"("Ler ZPit" ("String")) -> ()
                  n854 = Increment(x=w459) -> (x+1=w458:i32)
                  n855 = property on="N fit 2" class="DigNum (strict)"() -> ("Value"=w456:i32)  [unwired: 2 in, 2 out]
                  n856 = Equal?(x=w458, y=w456) -> (x = y?=w457:bool)
                  n857 = case shown="True" w457 {
                    frame False {
                    }
                    frame True {
                      n858 = local write "Estagio auto"(3 ("Estagio auto")) -> ()
                    }
                  }
                }
                frame 3 {
                  w467 = "\t"
                  n859 = property on="SET" class="DigNum (strict)"() -> ("Value"=w463:i32)  [unwired: 2 in, 2 out]
                  n860 = property on="Read ZPit" class="Bool (strict)"() -> ("Value"=w462:bool)  [unwired: 2 in, 2 out]
                  n861 = case shown="False" w462 {
                    tunnel: ["  ==>" w474] -> w468
                    frame False {
                    }
                    frame True {
                      n862 = property on="P fit" class="DigNum (strict)"() -> ("Value"=w473:dbl)  [unwired: 2 in, 2 out]
                      n863 = Number To Fractional String(number=w473, precision (6)=i16 3) -> (F-format string=w474:string)  [unwired: 2 in]
                    }
                  }
                  n864 = Number To Decimal String(number=w463) -> (decimal integer string=w466:string)  [unwired: 1 in]
                  n865 = Concatenate Strings(w466, w467, w468, w467) -> (w465:string)
                  n866 = flat-sequence {
                    tunnel: [w478] -> w470
                    tunnel: [w477] -> w469
                    tunnel: w465 -> [w476]
                    tunnel: w464 -> [w475]
                    tunnel: w470 -> [w494]
                    tunnel: w469 -> [w493]
                    frame #0 {
                      n867 = Open/Create/Replace File(file path (use dialog)=w475, operation (0:open)=T3."open") -> (refnum out=w484:refnum<file>, error out=w485:errorcluster)  [unwired: 2 in, 3 out]
                      n868 = Set File Position(refnum=w484, from (0:start)=enum16{"start", "end", "current"}."end", error in=w485) -> (refnum out=w482:refnum<file>, error out=w481:errorcluster)  [unwired: 1 in]
                      n869 = Write to Text File(file (use dialog)=w482, text=w476, error in=w481) -> (refnum out=w486:refnum<file>, error out=w487:errorcluster)  [unwired: 2 out]
                      n870 = Close File(refnum=w486, error in=w487) -> (path=w478:path, error out=w479:errorcluster)
                      n871 = call <vilib>:"Simple Error Handler.vi"("error in (no error)"=w479) -> ("error out"=w477:errorcluster)  [unwired: 1 in, 7 out]
                    }
                    frame #1 {
                      w488 = 0 ("limpo")
                      n872 = local write "Estagio auto"(4 ("Estagio auto")) -> ()
                      n873 = local write "ZPit 2"(TRUE ("ZPit")) -> ()
                      n874 = Wait (ms)(milliseconds to wait=u32 500) -> ()  [unwired: 1 out]
                      n875 = local write "limpo"(w488) -> ()
                      n876 = Read from Text File(file (use dialog)=w494, count=-1 ("Count  3"), error in=w493) -> (refnum out=w495:refnum<file>, text=w499:string, error out=w496:errorcluster)  [unwired: 1 in, 1 out]
                      n877 = local write "String 3"(w499) -> ()
                      n878 = local write "estagio 5"(w488) -> ()
                      n879 = Close File(refnum=w495, error in=w496) -> (error out=w497:errorcluster)  [unwired: 1 out]
                      n880 = local write "String"("abrir valvula entrada gas" ("String")) -> ()
                      n881 = call <vilib>:"Simple Error Handler.vi"("error in (no error)"=w497) -> ()  [unwired: 1 in, 8 out]
                    }
                    frame #2 {
                      w500 = T4 3 items=["no dialog", "OK message", "continue or stop message", "OK message + warnings", "continue/stop + warnings"] ("type of dialog (OK msg:1)")
                      w506 = TRUE ("Boolean 4")
                      n882 = local write "Entrada gás 2"(w506) -> ()
                      n883 = call-poly <vilib>:"DAQmx Create Virtual Channel.vi"("lines"=tag "Dev1/port0/line1") -> ("task out"=w508:refnum<k21>, "error out"=w509:errorcluster)  [unwired: 13 in]
                      n884 = call <vilib>:"DAQmx Start Task.vi"("task/channels in"=w508, "error in"=w509) -> ("task out"=w510:refnum<k21>, "error out"=w511:errorcluster)  [unwired: 12 in]
                      n885 = call-poly <vilib>:"DAQmx Write.vi"("task/channels in"=w510, "data"=w506, "error in"=w511) -> ("task out"=w503:refnum<k21>, "error out"=w502:errorcluster)  [unwired: 10 in, 1 out]
                      n886 = call <vilib>:"DAQmx Stop Task.vi"("task/channels in"=w503, "error in"=w502) -> ("task out"=w504:refnum<k21>, "error out"=w505:errorcluster)  [unwired: 12 in]
                      n887 = call <vilib>:"DAQmx Clear Task.vi"("task in"=w504, "error in"=w505) -> ("error out"=w501:errorcluster)  [unwired: 13 in]
                      n888 = call <vilib>:"Simple Error Handler.vi"("type of dialog (OK msg:1)"=w500, "error in (no error)"=w501) -> ()  [unwired: 3 in, 5 out]
                    }
                  }
                }
                frame 4 {
                  n889 = Greater Or Equal?(x=w513, y="Set P auto") -> (x >= y?=w514:bool)
                  n890 = case shown="True" w514 {
                    tunnel: "Set P auto" -> [_ w529]
                    frame False {
                      w522 = T4 3 items=["no dialog", "OK message", "continue or stop message", "OK message + warnings", "continue/stop + warnings"] ("type of dialog (OK msg:1)")
                      w528 = TRUE ("data")
                      n891 = local write "Estagio auto"(5 ("Estagio auto")) -> ()
                      n892 = Wait (ms)(milliseconds to wait=u32 500) -> ()  [unwired: 1 out]
                      n893 = local write "Entrada gás 2"(w528) -> ()
                      n894 = call-poly <vilib>:"DAQmx Create Virtual Channel.vi"("lines"=tag "Dev1/port0/line1") -> ("task out"=w519:refnum<k21>, "error out"=w518:errorcluster)  [unwired: 13 in]
                      n895 = call <vilib>:"DAQmx Start Task.vi"("task/channels in"=w519, "error in"=w518) -> ("task out"=w517:refnum<k21>, "error out"=w516:errorcluster)  [unwired: 12 in]
                      n896 = call-poly <vilib>:"DAQmx Write.vi"("task/channels in"=w517, "data"=w528, "error in"=w516) -> ("task out"=w525:refnum<k21>, "error out"=w524:errorcluster)  [unwired: 10 in, 1 out]
                      n897 = call <vilib>:"DAQmx Stop Task.vi"("task/channels in"=w525, "error in"=w524) -> ("task out"=w527:refnum<k21>, "error out"=w526:errorcluster)  [unwired: 12 in]
                      n898 = call <vilib>:"DAQmx Clear Task.vi"("task in"=w527, "error in"=w526) -> ("error out"=w523:errorcluster)  [unwired: 13 in]
                      n899 = call <vilib>:"Simple Error Handler.vi"("type of dialog (OK msg:1)"=w522, "error in (no error)"=w523) -> ()  [unwired: 3 in, 5 out]
                    }
                    frame True {
                      n900 = flat-sequence {
                        tunnel: [w532] -> w530
                        tunnel: w529 -> [w532]
                        tunnel: [w547] -> w531
                        tunnel: w530 -> [w546]
                        tunnel: w531 -> [w561]
                        frame #0 {
                          w538 = T4 3 items=["no dialog", "OK message", "continue or stop message", "OK message + warnings", "continue/stop + warnings"] ("type of dialog (OK msg:1)")
                          w545 = FALSE ("data")
                          n901 = Wait (ms)(milliseconds to wait=u32 500) -> ()  [unwired: 1 out]
                          n902 = local write "Entrada gás 2"(w545) -> ()
                          n903 = call-poly <vilib>:"DAQmx Create Virtual Channel.vi"("lines"=tag "Dev1/port0/line1") -> ("task out"=w536:refnum<k21>, "error out"=w537:errorcluster)  [unwired: 13 in]
                          n904 = call <vilib>:"DAQmx Start Task.vi"("task/channels in"=w536, "error in"=w537) -> ("task out"=w534:refnum<k21>, "error out"=w533:errorcluster)  [unwired: 12 in]
                          n905 = call-poly <vilib>:"DAQmx Write.vi"("task/channels in"=w534, "data"=w545, "error in"=w533) -> ("task out"=w542:refnum<k21>, "error out"=w541:errorcluster)  [unwired: 10 in, 1 out]
                          n906 = call <vilib>:"DAQmx Stop Task.vi"("task/channels in"=w542, "error in"=w541) -> ("task out"=w544:refnum<k21>, "error out"=w543:errorcluster)  [unwired: 12 in]
                          n907 = call <vilib>:"DAQmx Clear Task.vi"("task in"=w544, "error in"=w543) -> ("error out"=w539:errorcluster)  [unwired: 13 in]
                          n908 = call <vilib>:"Simple Error Handler.vi"("type of dialog (OK msg:1)"=w538, "error in (no error)"=w539) -> ()  [unwired: 3 in, 5 out]
                        }
                        frame #1 {
                          n909 = stacked-sequence {
                            tunnel: [_ _ _ w558] -> w547
                            tunnel: w546 -> [_ _ w551 _]
                            frame #0 {
                              n910 = call "Controle_ATM.vi"("seconds to wait"=2.0) -> ("Atm"=w549:bool)  [unwired: 9 in, 1 out]
                              n911 = local write "Atm 2"(w549) -> ()
                            }
                            frame #1 {
                              n912 = Wait (ms)(milliseconds to wait=u32 1000) -> ()  [unwired: 1 out]
                            }
                            frame #2 {
                              n913 = Less Or Equal?(x=w551, y=1.5) -> (x <= y?=w553:bool)
                              n914 = case shown="True" w553 {
                                frame False {
                                n915 = call "Controle_ATM.vi"("seconds to wait"=2.0) -> ()  [unwired: 9 in, 2 out]
                                }
                                frame True {
                                w556 = TRUE ("Vácuo")
                                n916 = local write "Vácuo 2"(w556) -> ()
                                n917 = call "Controle_vacuo.vi"("time (s) to wait vacuo"=3.0, "Boolean"=w556) -> ("Vacuo"=w557:bool)  [unwired: 9 in]
                                n918 = local write "Vácuo 2"(w557) -> ()
                                }
                              }
                            }
                            frame #3 {
                              n919 = property on="limpo" class="DigNum (strict)"() -> ("Value"=w559:i32)  [unwired: 2 in, 2 out]
                              n920 = Wait (ms)(milliseconds to wait=u32 1000) -> ()  [unwired: 1 out]
                              n921 = Increment(x=w559) -> (x+1=w558:i32)
                            }
                          }
                        }
                        frame #2 {
                          "limpo" <- w561
                        }
                      }
                    }
                  }
                }
                frame 5 {
                  n922 = property on="Set P auto" class="DigNum (strict)"() -> ("Value"=w563:dbl)  [unwired: 2 in, 2 out]
                  n923 = Greater Or Equal?(x=w564, y=w563) -> (x >= y?=w562:bool)
                  n924 = case shown="True" w562 {
                    selector: w562 -> [_ w586]
                    frame False {
                      n925 = flat-sequence {
                        tunnel: [w566] -> w565
                        tunnel: w565 -> [w582]
                        frame #0 {
                          w569 = T4 3 items=["no dialog", "OK message", "continue or stop message", "OK message + warnings", "continue/stop + warnings"] ("type of dialog (OK msg:1)")
                          w579 = TRUE ("Boolean 4")
                          n926 = property on="estagio 5" class="DigNum (strict)"() -> ("Value"=w567:i32)  [unwired: 2 in, 2 out]
                          n927 = local write "Entrada gás 2"(w579) -> ()
                          n928 = Increment(x=w567) -> (x+1=w566:i32)
                          n929 = call-poly <vilib>:"DAQmx Create Virtual Channel.vi"("lines"=tag "Dev1/port0/line1") -> ("task out"=w573:refnum<k21>, "error out"=w572:errorcluster)  [unwired: 13 in]
                          n930 = call <vilib>:"DAQmx Start Task.vi"("task/channels in"=w573, "error in"=w572) -> ("task out"=w571:refnum<k21>, "error out"=w570:errorcluster)  [unwired: 12 in]
                          n931 = call-poly <vilib>:"DAQmx Write.vi"("task/channels in"=w571, "data"=w579, "error in"=w570) -> ("task out"=w576:refnum<k21>, "error out"=w575:errorcluster)  [unwired: 10 in, 1 out]
                          n932 = call <vilib>:"DAQmx Stop Task.vi"("task/channels in"=w576, "error in"=w575) -> ("task out"=w577:refnum<k21>, "error out"=w578:errorcluster)  [unwired: 12 in]
                          n933 = call <vilib>:"DAQmx Clear Task.vi"("task in"=w577, "error in"=w578) -> ("error out"=w568:errorcluster)  [unwired: 13 in]
                          n934 = call <vilib>:"Simple Error Handler.vi"("type of dialog (OK msg:1)"=w569, "error in (no error)"=w568) -> ()  [unwired: 3 in, 5 out]
                        }
                        frame #1 {
                          n935 = Less?(x=w582, y=6) -> (x < y?=w580:bool)
                          n936 = case shown="False" w580 {
                            frame False {
                              n937 = local write "Estagio auto"(5 ("Estagio auto")) -> ()
                            }
                            frame True {
                              n938 = local write "Estagio auto"(4 ("Estagio auto")) -> ()
                            }
                          }
                          "estagio 5" <- w582
                        }
                      }
                    }
                    frame True {
                      n939 = flat-sequence {
                        tunnel: w586 -> [w587]
                        tunnel: [w587] -> w585
                        tunnel: w585 -> [w603]
                        frame #0 {
                          w588 = FALSE ("Boolean 4")
                          w593 = T4 3 items=["no dialog", "OK message", "continue or stop message", "OK message + warnings", "continue/stop + warnings"] ("type of dialog (OK msg:1)")
                          n940 = local write "Entrada gás 2"(w588) -> ()
                          n941 = call-poly <vilib>:"DAQmx Create Virtual Channel.vi"("lines"=tag "Dev1/port0/line1") -> ("task out"=w591:refnum<k21>, "error out"=w592:errorcluster)  [unwired: 13 in]
                          n942 = call <vilib>:"DAQmx Start Task.vi"("task/channels in"=w591, "error in"=w592) -> ("task out"=w594:refnum<k21>, "error out"=w595:errorcluster)  [unwired: 12 in]
                          n943 = call-poly <vilib>:"DAQmx Write.vi"("task/channels in"=w594, "data"=w588, "error in"=w595) -> ("task out"=w599:refnum<k21>, "error out"=w596:errorcluster)  [unwired: 10 in, 1 out]
                          n944 = call <vilib>:"DAQmx Stop Task.vi"("task/channels in"=w599, "error in"=w596) -> ("task out"=w598:refnum<k21>, "error out"=w597:errorcluster)  [unwired: 12 in]
                          n945 = call <vilib>:"DAQmx Clear Task.vi"("task in"=w598, "error in"=w597) -> ("error out"=w590:errorcluster)  [unwired: 13 in]
                          n946 = call <vilib>:"Simple Error Handler.vi"("type of dialog (OK msg:1)"=w593, "error in (no error)"=w590) -> ()  [unwired: 3 in, 5 out]
                        }
                        frame #1 {
                          n947 = property on="estagio 5" class="DigNum (strict)"() -> ("Value"=w601:i32)  [unwired: 2 in, 2 out]
                          n948 = Greater?(x=w601, y=5) -> (0:w604:bool)
                          n949 = And(x=w603, y=w604) -> (x .and. y?=w602:bool)
                          n950 = case shown="True" w602 {
                            frame False {
                              n951 = local write "Estagio auto"(4 ("Estagio auto")) -> ()
                              n952 = Wait (ms)(milliseconds to wait=u32 500) -> ()  [unwired: 1 out]
                            }
                            frame True {
                              n953 = property on="Contador" class="DigNum (strict)"() -> ("Value"=w608:i32)  [unwired: 2 in, 2 out]
                              n954 = local write "String"("Ler Pit" ("String")) -> ()
                              n955 = Increment(x=w608) -> (x+1=w610:i32)
                              n956 = property on="N fit 2" class="DigNum (strict)"() -> ("Value"=w607:i32)  [unwired: 2 in, 2 out]
                              n957 = Equal?(x=w610, y=w607) -> (x = y?=w609:bool)
                              n958 = case shown="True" w609 {
                                frame False {
                                }
                                frame True {
                                n959 = local write "Estagio auto"(6 ("Estagio auto")) -> ()
                                }
                              }
                            }
                          }
                        }
                      }
                    }
                  }
                }
                frame 6 {
                  n960 = property on="Contador" class="DigNum (strict)"() -> ("Value"=w614:i32)  [unwired: 2 in, 2 out]
                  n961 = Increment(x=w614) -> (x+1=w616:i32)
                  n962 = property on="N fit 2" class="DigNum (strict)"() -> ("Value"=w613:i32)  [unwired: 2 in, 2 out]
                  n963 = Equal?(x=w616, y=w613) -> (x = y?=w615:bool)
                  n964 = case shown="True" w615 {
                    tunnel: w617 -> [_ w618]
                    frame False {
                    }
                    frame True {
                      n965 = property on="P fit" class="DigNum (strict)"() -> ("Value"=w619:dbl)  [unwired: 2 in, 2 out]
                      n966 = Number To Fractional String(number=w619, precision (6)=i16 3) -> (F-format string=w623:string)  [unwired: 2 in]
                      n967 = Concatenate Strings(w623, "\t") -> (w621:string)
                      n968 = flat-sequence {
                        tunnel: [w629] -> w625
                        tunnel: [w628] -> w624
                        tunnel: w621 -> [w627]
                        tunnel: w618 -> [w626]
                        tunnel: w625 -> [w645]
                        tunnel: w624 -> [w644]
                        frame #0 {
                          n969 = Open/Create/Replace File(file path (use dialog)=w626, operation (0:open)=T3."open") -> (refnum out=w635:refnum<file>, error out=w636:errorcluster)  [unwired: 2 in, 3 out]
                          n970 = Set File Position(refnum=w635, from (0:start)=enum16{"start", "end", "current"}."end", error in=w636) -> (refnum out=w633:refnum<file>, error out=w632:errorcluster)  [unwired: 1 in]
                          n971 = Write to Text File(file (use dialog)=w633, text=w627, error in=w632) -> (refnum out=w637:refnum<file>, error out=w638:errorcluster)  [unwired: 2 out]
                          n972 = Close File(refnum=w637, error in=w638) -> (path=w629:path, error out=w630:errorcluster)
                          n973 = call <vilib>:"Simple Error Handler.vi"("error in (no error)"=w630) -> ("error out"=w628:errorcluster)  [unwired: 1 in, 7 out]
                        }
                        frame #1 {
                          n974 = local write "Estagio auto"(7 ("Estagio auto")) -> ()
                          n975 = local write "teste slope"(0 ("teste slope")) -> ()
                          n976 = local write "Pit 2"(TRUE ("ZPit")) -> ()
                          n977 = Wait (ms)(milliseconds to wait=u32 500) -> ()  [unwired: 1 out]
                          n978 = Read from Text File(file (use dialog)=w645, count=-1 ("Count  3"), error in=w644) -> (refnum out=w646:refnum<file>, text=w650:string, error out=w647:errorcluster)  [unwired: 1 in, 1 out]
                          n979 = local write "String 3"(w650) -> ()
                          n980 = Close File(refnum=w646, error in=w647) -> (error out=w648:errorcluster)  [unwired: 1 out]
                          n981 = call <vilib>:"Simple Error Handler.vi"("error in (no error)"=w648) -> ()  [unwired: 1 in, 8 out]
                          n982 = local write "String"("abrir valvula entrada camara" ("String")) -> ()
                        }
                      }
                    }
                  }
                }
                frame 7 {
                  n983 = flat-sequence {
                    tunnel: w657 -> [w661]
                    tunnel: w658 -> [w662]
                    tunnel: w659 -> [w663]
                    tunnel: [w663] -> w656
                    tunnel: [w662] -> w654
                    tunnel: [w661] -> w652
                    tunnel: w656 -> [w666]
                    tunnel: [w666] -> w655
                    tunnel: w654 -> [w664]
                    tunnel: [w664] -> w653
                    tunnel: w652 -> [w665]
                    tunnel: [w665] -> w651
                    tunnel: w655 -> [_]
                    tunnel: w653 -> [_]
                    tunnel: w651 -> [_]
                    frame #0 {
                      n984 = local write "N fit"("N fit patamar") -> ()
                    }
                    frame #1 {
                      n985 = flat-sequence {
                        tunnel: w666 -> [w671]
                        tunnel: w664 -> [w670]
                        tunnel: w665 -> [w669]
                        frame #0 {
                          (unwired) i16 6 ("precision (6)")
                          w668 = "\t"
                          w688 = i16 4 ("precision (6)")
                          n986 = Number To Fractional String(number=w670, precision (6)=w688) -> (F-format string=w683:string)  [unwired: 2 in]
                          n987 = Number To Fractional String(number=w669, precision (6)=w688) -> (F-format string=w682:string)  [unwired: 2 in]
                          n988 = Get Date/Time String(date format (0)=enum16{"short", "long", "abbreviated"}."short", want seconds? (F)=TRUE) -> (date string=w685:string, time string=w684:string)  [unwired: 1 in]
                          n989 = Open/Create/Replace File(file path (use dialog)=w671, operation (0:open)=T3."open") -> (refnum out=w679:refnum<file>, error out=w672:errorcluster)  [unwired: 2 in, 3 out]
                          n990 = Concatenate Strings(w685, w668, w684, w668, w683, w668, w682, w668, w668, "\r\n") -> (w673:string)
                          n991 = Set File Position(refnum=w679, from (0:start)=enum16{"start", "end", "current"}."end", error in=w672) -> (refnum out=w677:refnum<file>, error out=w676:errorcluster)  [unwired: 1 in]
                          n992 = Write to Text File(file (use dialog)=w677, text=w673, error in=w676) -> (refnum out=w680:refnum<file>, error out=w681:errorcluster)  [unwired: 2 out]
                          n993 = Close File(refnum=w680, error in=w681) -> (error out=w674:errorcluster)  [unwired: 1 out]
                          n994 = call <vilib>:"Simple Error Handler.vi"("error in (no error)"=w674) -> ()  [unwired: 1 in, 8 out]
                        }
                      }
                    }
                    frame #2 {
                      n995 = property on="Contador" class="DigNum (strict)"() -> ("Value"=w697:i32)  [unwired: 2 in, 2 out]
                      n996 = Increment(x=w697) -> (x+1=w696:i32)
                      n997 = property on="N fit patamar" class="DigNum (strict)"() -> ("Value"=w689:i32)  [unwired: 2 in, 2 out]
                      n998 = Equal?(x=w696, y=w689) -> (x = y?=w698:bool)
                      n999 = case shown="True" w698 {
                        tunnel: [FALSE w703] -> w695
                        tunnel: [_ w702] -> w694
                        frame False {
                        }
                        frame True {
                          n1000 = property on="P (bar/s)" class="DigNum (strict)"() -> ("Value"=w705:dbl)  [unwired: 2 in, 2 out]
                          n1001 = Absolute Value(x=w705) -> (abs(x)=w704:dbl)
                          n1002 = Less Or Equal?(x=w704, y="STOP (bar/s)") -> (x <= y?=w703:bool)
                          n1003 = case shown="True" w703 {
                            tunnel: [_ w707] -> w702
                            frame False {
                            }
                            frame True {
                              n1004 = property on="teste slope" class="DigNum (strict)"() -> ("Value"=w708:i32)  [unwired: 2 in, 2 out]
                              n1005 = local write "Estagio auto"(7 ("Estagio auto")) -> ()
                              n1006 = Increment(x=w708) -> (x+1=w707:i32)
                              "teste slope" <- w707
                            }
                          }
                        }
                      }
                      n1007 = Greater Or Equal?(x=w694, y="Ntest") -> (x >= y?=w692:bool)
                      n1008 = And(x=w698, y=w692) -> (x .and. y?=w691:bool)
                      n1009 = case shown="True" w691 {
                        frame False {
                        }
                        frame True {
                          n1010 = flat-sequence {
                            frame #0 {
                              n1011 = property on="N fit 2" class="DigNum (strict)"() -> ("Value"=w746:i32)  [unwired: 2 in, 2 out]
                              n1012 = Wait (ms)(milliseconds to wait=u32 500) -> ()  [unwired: 1 out]
                              n1013 = local write "N fit"(w746) -> ()
                            }
                            frame #1 {
                              n1014 = local write "Estagio auto"(8 ("Estagio auto")) -> ()
                            }
                          }
                        }
                      }
                      n1015 = case shown="True" w691 {
                        tunnel: [TRUE ("Boolean") FALSE ("Boolean")] -> w690
                        frame False {
                        }
                        frame True {
                        }
                      }
                      n1016 = case shown="True" w695 {
                        tunnel: w690 -> [_ w726]
                        frame False {
                          w722 = T4 3 items=["no dialog", "OK message", "continue or stop message", "OK message + warnings", "continue/stop + warnings"] ("type of dialog (OK msg:1)")
                          w710 = TRUE ("Boolean")
                          n1017 = call-poly <vilib>:"DAQmx Create Virtual Channel.vi"("lines"=tag "Dev1/port0/line3") -> ("task out"=w712:refnum<k21>, "error out"=w713:errorcluster)  [unwired: 13 in]
                          n1018 = Wait (ms)(milliseconds to wait="patamar milliseconds to wait") -> ()  [unwired: 1 out]
                          n1019 = call <vilib>:"DAQmx Start Task.vi"("task/channels in"=w712, "error in"=w713) -> ("task out"=w714:refnum<k21>, "error out"=w715:errorcluster)  [unwired: 12 in]
                          n1020 = case shown="True" w710 {
                            frame False {
                            }
                            frame True {
                              n1021 = property on="Vol Ref 3" class="Slide (strict)"() -> ("Value"=w723:dbl)  [unwired: 2 in, 2 out]
                              n1022 = local write "Camara 2"(w723) -> ()
                            }
                          }
                          n1023 = local write "Câmara 2"(w710) -> ()
                          n1024 = call-poly <vilib>:"DAQmx Write.vi"("task/channels in"=w714, "data"=w710, "error in"=w715) -> ("task out"=w719:refnum<k21>, "error out"=w720:errorcluster)  [unwired: 10 in, 1 out]
                          n1025 = call <vilib>:"DAQmx Stop Task.vi"("task/channels in"=w719, "error in"=w720) -> ("task out"=w717:refnum<k21>, "error out"=w716:errorcluster)  [unwired: 12 in]
                          n1026 = call <vilib>:"DAQmx Clear Task.vi"("task in"=w717, "error in"=w716) -> ("error out"=w721:errorcluster)  [unwired: 13 in]
                          n1027 = call <vilib>:"Simple Error Handler.vi"("type of dialog (OK msg:1)"=w722, "error in (no error)"=w721) -> ()  [unwired: 3 in, 5 out]
                        }
                        frame True {
                          n1028 = flat-sequence {
                            tunnel: w726 -> [w727]
                            tunnel: [w727] -> w724
                            tunnel: [w729] -> w725
                            tunnel: w724 -> [w730]
                            tunnel: w725 -> [w733]
                            frame #0 {
                            }
                            frame #1 {
                              n1029 = case shown="True" "Read val open" {
                                tunnel: [w731 TRUE ("Boolean")] -> w729
                                tunnel: w730 -> [w731 _]
                                frame False {
                                }
                                frame True {
                                }
                              }
                            }
                            frame #2 {
                              w735 = T4 3 items=["no dialog", "OK message", "continue or stop message", "OK message + warnings", "continue/stop + warnings"] ("type of dialog (OK msg:1)")
                              n1030 = local write "Câmara 2"(w733) -> ()
                              n1031 = call-poly <vilib>:"DAQmx Create Virtual Channel.vi"("lines"=tag "Dev1/port0/line3") -> ("task out"=w744:refnum<k21>, "error out"=w743:errorcluster)  [unwired: 13 in]
                              n1032 = call <vilib>:"DAQmx Start Task.vi"("task/channels in"=w744, "error in"=w743) -> ("task out"=w742:refnum<k21>, "error out"=w741:errorcluster)  [unwired: 12 in]
                              n1033 = call-poly <vilib>:"DAQmx Write.vi"("task/channels in"=w742, "data"=w733, "error in"=w741) -> ("task out"=w737:refnum<k21>, "error out"=w736:errorcluster)  [unwired: 10 in, 1 out]
                              n1034 = call <vilib>:"DAQmx Stop Task.vi"("task/channels in"=w737, "error in"=w736) -> ("task out"=w739:refnum<k21>, "error out"=w740:errorcluster)  [unwired: 12 in]
                              n1035 = call <vilib>:"DAQmx Clear Task.vi"("task in"=w739, "error in"=w740) -> ("error out"=w734:errorcluster)  [unwired: 13 in]
                              n1036 = call <vilib>:"Simple Error Handler.vi"("type of dialog (OK msg:1)"=w735, "error in (no error)"=w734) -> ()  [unwired: 3 in, 5 out]
                            }
                            frame #3 {
                              n1037 = Wait (ms)(milliseconds to wait=u32 2000) -> ()  [unwired: 1 out]
                            }
                          }
                        }
                      }
                    }
                  }
                }
                frame 8 {
                  n1038 = property on="Contador" class="DigNum (strict)"() -> ("Value"=w777:i32)  [unwired: 2 in, 2 out]
                  n1039 = Increment(x=w777) -> (x+1=w778:i32)
                  n1040 = property on="N fit 2" class="DigNum (strict)"() -> ("Value"=w751:i32)  [unwired: 2 in, 2 out]
                  n1041 = Equal?(x=w778, y=w751) -> (x = y?=w776:bool)
                  n1042 = case shown="True" w776 {
                    tunnel: w779 -> [_ w1488]
                    frame False {
                    }
                    frame True {
                      n1043 = property on="P fit" class="DigNum (strict)"() -> ("Value"=w1489:dbl)  [unwired: 2 in, 2 out]
                      n1044 = Number To Fractional String(number=w1489, precision (6)=i16 3) -> (F-format string=w1493:string)  [unwired: 2 in]
                      n1045 = Concatenate Strings(w1493, "\t") -> (w1491:string)
                      n1046 = flat-sequence {
                        tunnel: [w1500] -> w1495
                        tunnel: [w1499] -> w1494
                        tunnel: w1491 -> [w1498]
                        tunnel: w1488 -> [w1497]
                        tunnel: w1495 -> [w1515]
                        tunnel: w1494 -> [w1514]
                        frame #0 {
                          n1047 = Wait (ms)(milliseconds to wait=u32 500) -> ()  [unwired: 1 out]
                          n1048 = Open/Create/Replace File(file path (use dialog)=w1497, operation (0:open)=T3."open") -> (refnum out=w1506:refnum<file>, error out=w1507:errorcluster)  [unwired: 2 in, 3 out]
                          n1049 = Set File Position(refnum=w1506, from (0:start)=enum16{"start", "end", "current"}."end", error in=w1507) -> (refnum out=w1504:refnum<file>, error out=w1503:errorcluster)  [unwired: 1 in]
                          n1050 = Write to Text File(file (use dialog)=w1504, text=w1498, error in=w1503) -> (refnum out=w1508:refnum<file>, error out=w1509:errorcluster)  [unwired: 2 out]
                          n1051 = Close File(refnum=w1508, error in=w1509) -> (path=w1500:path, error out=w1501:errorcluster)
                          n1052 = call <vilib>:"Simple Error Handler.vi"("error in (no error)"=w1501) -> ("error out"=w1499:errorcluster)  [unwired: 1 in, 7 out]
                        }
                        frame #1 {
                          n1053 = local write "Estagio auto"(9 ("Estagio auto")) -> ()
                          n1054 = local write "Pf2 2"(TRUE ("ZPit")) -> ()
                          n1055 = Wait (ms)(milliseconds to wait=u32 500) -> ()  [unwired: 1 out]
                          n1056 = Read from Text File(file (use dialog)=w1515, count=-1 ("Count  3"), error in=w1514) -> (refnum out=w1516:refnum<file>, text=w1520:string, error out=w1517:errorcluster)  [unwired: 1 in, 1 out]
                          n1057 = local write "String 3"(w1520) -> ()
                          n1058 = Close File(refnum=w1516, error in=w1517) -> (error out=w1518:errorcluster)  [unwired: 1 out]
                          n1059 = call <vilib>:"Simple Error Handler.vi"("error in (no error)"=w1518) -> ()  [unwired: 1 in, 8 out]
                          n1060 = local write "String"("abrir valvula vacuo" ("String")) -> ()
                        }
                        frame #2 {
                          n1061 = flat-sequence {
                            tunnel: [w1521] -> _
                            frame #0 {
                              w1521 = FALSE ("data")
                              w1523 = T4 3 items=["no dialog", "OK message", "continue or stop message", "OK message + warnings", "continue/stop + warnings"] ("type of dialog (OK msg:1)")
                              n1062 = local write "Câmara 2"(w1521) -> ()
                              n1063 = call-poly <vilib>:"DAQmx Create Virtual Channel.vi"("lines"=tag "Dev1/port0/line3") -> ("task out"=w1532:refnum<k21>, "error out"=w1531:errorcluster)  [unwired: 13 in]
                              n1064 = call <vilib>:"DAQmx Start Task.vi"("task/channels in"=w1532, "error in"=w1531) -> ("task out"=w1530:refnum<k21>, "error out"=w1529:errorcluster)  [unwired: 12 in]
                              n1065 = call-poly <vilib>:"DAQmx Write.vi"("task/channels in"=w1530, "data"=w1521, "error in"=w1529) -> ("task out"=w1525:refnum<k21>, "error out"=w1524:errorcluster)  [unwired: 10 in, 1 out]
                              n1066 = call <vilib>:"DAQmx Stop Task.vi"("task/channels in"=w1525, "error in"=w1524) -> ("task out"=w1527:refnum<k21>, "error out"=w1528:errorcluster)  [unwired: 12 in]
                              n1067 = call <vilib>:"DAQmx Clear Task.vi"("task in"=w1527, "error in"=w1528) -> ("error out"=w1522:errorcluster)  [unwired: 13 in]
                              n1068 = call <vilib>:"Simple Error Handler.vi"("type of dialog (OK msg:1)"=w1523, "error in (no error)"=w1522) -> ()  [unwired: 3 in, 5 out]
                            }
                            frame #1 {
                              n1069 = Wait (ms)(milliseconds to wait=u32 2000) -> ()  [unwired: 1 out]
                            }
                          }
                        }
                      }
                    }
                  }
                  n1070 = case shown="False" w775 {
                    tunnel: [FALSE ("Save manual") w1487] -> w755
                    tunnel: w776 -> [_ w1487]
                    frame False {
                    }
                    frame True {
                    }
                  }
                  n1071 = flat-sequence {
                    tunnel: w755 -> [w781]
                    tunnel: w758 -> [w782]
                    tunnel: [w782] -> w753
                    tunnel: [w781] -> w752
                    tunnel: [w786] -> w774
                    tunnel: [w788] -> w773
                    tunnel: [w789] -> w772
                    tunnel: [w790] -> w771
                    tunnel: [w791] -> w770
                    tunnel: [w792] -> w769
                    tunnel: [w793] -> w768
                    tunnel: [w794] -> w767
                    tunnel: [w795] -> w766
                    tunnel: [w796] -> w765
                    tunnel: [w797] -> w764
                    tunnel: [w798] -> w763
                    tunnel: [w799] -> w762
                    tunnel: [w800] -> w761
                    tunnel: [w801] -> w760
                    tunnel: [w787] -> w759
                    tunnel: [w785] -> w756
                    tunnel: w753 -> [w803]
                    tunnel: w752 -> [w802]
                    tunnel: [w784] -> w750
                    tunnel: [w783] -> w749
                    tunnel: w774 -> [w1431]
                    tunnel: w773 -> [w1430]
                    tunnel: w772 -> [w1429]
                    tunnel: w771 -> [w1428]
                    tunnel: w770 -> [w1427]
                    tunnel: w769 -> [w1426]
                    tunnel: w768 -> [w1425]
                    tunnel: w767 -> [w1424]
                    tunnel: w766 -> [w1423]
                    tunnel: w765 -> [w1422]
                    tunnel: w764 -> [w1421]
                    tunnel: w763 -> [w1420]
                    tunnel: w762 -> [w1419]
                    tunnel: w761 -> [w1418]
                    tunnel: w760 -> [w1417]
                    tunnel: w759 -> [w1416]
                    tunnel: [w1414] -> w757
                    tunnel: w756 -> [w1414]
                    tunnel: [TRUE ("graph RLC")] -> w754
                    tunnel: w750 -> [w1413]
                    tunnel: w749 -> [w1412]
                    frame #0 {
                      n1072 = local write "graph RLC"(FALSE) -> ()
                    }
                    frame #1 {
                      n1073 = case shown="True" w802 {
                        tunnel: [FALSE w844] -> w785
                        tunnel: w803 -> [_ w826]
                        tunnel: [_ w824] -> w786
                        tunnel: [_ w823] -> w787
                        tunnel: [_ w822] -> w788
                        tunnel: [_ w821] -> w789
                        tunnel: [_ w820] -> w790
                        tunnel: [_ w819] -> w791
                        tunnel: [_ w818] -> w792
                        tunnel: [_ w817] -> w793
                        tunnel: [_ w816] -> w794
                        tunnel: [_ w815] -> w795
                        tunnel: [_ w814] -> w796
                        tunnel: [_ w813] -> w797
                        tunnel: [_ w812] -> w798
                        tunnel: [_ w811] -> w799
                        tunnel: [_ w810] -> w800
                        tunnel: [_ w809] -> w801
                        tunnel: [_ w807] -> w784
                        tunnel: [_ w806] -> w783
                        frame False {
                        }
                        frame True {
                          n1074 = property on="path RLC_completo" class="Path"() -> ("Value"=w825:path)  [unwired: 2 in, 2 out]
                          n1075 = for {
                            N: 5 -> [_]
                            tunnel: TRUE -> [w869]
                            tunnel: FALSE -> [w868]
                            tunnel: [w867] -> w844
                            tunnel: [w866] -> w842 mode=indexing
                            tunnel: [w865] -> w841 mode=indexing
                            tunnel: [w864] -> w840 mode=indexing
                            tunnel: [w863] -> w839 mode=indexing
                            tunnel: [w862] -> w838 mode=indexing
                            tunnel: [w861] -> w837 mode=indexing
                            tunnel: [w860] -> w836 mode=indexing
                            tunnel: [w859] -> w835 mode=indexing
                            tunnel: [w858] -> w834 mode=indexing
                            tunnel: [w857] -> w833 mode=indexing
                            tunnel: [w856] -> w832 mode=indexing
                            tunnel: [w855] -> w831 mode=indexing
                            tunnel: [w854] -> w830 mode=indexing
                            tunnel: [w853] -> w829 mode=indexing
                            tunnel: [w852] -> w828 mode=indexing
                            tunnel: [w851] -> w827 mode=indexing
                            tunnel: w826 -> [w850]
                            tunnel: w825 -> [w849]
                            tunnel: [w848] -> w808 mode=indexing
                            tunnel: [w847] -> w805 mode=indexing
                            n1076 = stacked-sequence {
                              tunnel: w869 -> [_ w896 w930 w962 w994 w1026 w1059 w1091 w1123 w1155 w1187 w1219 w1251 w1283 w1316 w1349 w1381 _]
                              tunnel: w868 -> [w891 _ _ _ _ _ _ _ _ _ _ _ _ _ _ _ _ w1411]
                              tunnel: [_ _ _ _ _ _ _ _ _ _ _ _ _ _ _ _ _ TRUE] -> w867
                              tunnel: [_ w895 _ _ _ _ _ _ _ _ _ _ _ _ _ _ _ _] -> w866
                              tunnel: [_ _ w929 _ _ _ _ _ _ _ _ _ _ _ _ _ _ _] -> w865
                              tunnel: [_ _ _ w961 _ _ _ _ _ _ _ _ _ _ _ _ _ _] -> w864
                              tunnel: [_ _ _ _ w993 _ _ _ _ _ _ _ _ _ _ _ _ _] -> w863
                              tunnel: [_ _ _ _ _ w1025 _ _ _ _ _ _ _ _ _ _ _ _] -> w862
                              tunnel: [_ _ _ _ _ _ w1058 _ _ _ _ _ _ _ _ _ _ _] -> w861
                              tunnel: [_ _ _ _ _ _ _ w1090 _ _ _ _ _ _ _ _ _ _] -> w860
                              tunnel: [_ _ _ _ _ _ _ _ w1122 _ _ _ _ _ _ _ _ _] -> w859
                              tunnel: [_ _ _ _ _ _ _ _ _ w1154 _ _ _ _ _ _ _ _] -> w858
                              tunnel: [_ _ _ _ _ _ _ _ _ _ w1186 _ _ _ _ _ _ _] -> w857
                              tunnel: [_ _ _ _ _ _ _ _ _ _ _ w1218 _ _ _ _ _ _] -> w856
                              tunnel: [_ _ _ _ _ _ _ _ _ _ _ _ w1250 _ _ _ _ _] -> w855
                              tunnel: [_ _ _ _ _ _ _ _ _ _ _ _ _ w1282 _ _ _ _] -> w854
                              tunnel: [_ _ _ _ _ _ _ _ _ _ _ _ _ _ w1315 _ _ _] -> w853
                              tunnel: [_ _ _ _ _ _ _ _ _ _ _ _ _ _ _ w1348 _ _] -> w852
                              tunnel: [_ _ _ _ _ _ _ _ _ _ _ _ _ _ _ _ w1380 _] -> w851
                              tunnel: w850 -> [_ w894 w928 w960 w992 w1024 w1057 w1089 w1121 w1153 w1185 w1217 w1249 w1281 w1314 w1347 w1379 _]
                              tunnel: w849 -> [w870 w893 w927 w959 w991 w1023 w1056 w1088 w1120 w1152 w1184 w1216 w1248 w1280 w1313 w1346 w1378 _]
                              tunnel: [_ _ _ _ _ _ w1054 _ _ _ _ _ _ _ _ _ _ _] -> w848
                              tunnel: [_ _ _ _ _ _ _ _ _ _ _ _ _ _ w1311 _ _ _] -> w847
                              frame #0 {
                                w871 = "\t"
                                n1077 = local write "C-50-L"(w891) -> ()
                                n1078 = local write "C-50-N"(w891) -> ()
                                n1079 = local write "Z-50-L"(w891) -> ()
                                n1080 = local write "C-1K-N"(w891) -> ()
                                n1081 = local write "C-1K-L"(w891) -> ()
                                n1082 = local write "Z-50-N"(w891) -> ()
                                n1083 = local write "Z-1K-N"(w891) -> ()
                                n1084 = local write "Z-1K-L"(w891) -> ()
                                n1085 = local write "C-10K-L"(w891) -> ()
                                n1086 = local write "C-100-N"(w891) -> ()
                                n1087 = local write "C-10K-N"(w891) -> ()
                                n1088 = local write "Z-100-L"(w891) -> ()
                                n1089 = local write "Z-10K-L"(w891) -> ()
                                n1090 = local write "Z-100-N"(w891) -> ()
                                n1091 = local write "Z-10K-N"(w891) -> ()
                                n1092 = local write "C-100-L"(w891) -> ()
                                n1093 = Open/Create/Replace File(file path (use dialog)=w870, operation (0:open)=T3."open") -> (refnum out=w885:refnum<file>, error out=w884:errorcluster)  [unwired: 2 in, 3 out]
                                n1094 = Get Date/Time String(date format (0)=enum16{"short", "long", "abbreviated"}."short", want seconds? (F)=TRUE) -> (date string=w877:string, time string=w876:string)  [unwired: 1 in]
                                n1095 = feedback #4() -> (w875:dbl)  [unwired: 1 in]
                                "SET 2" <- w875
                                n1096 = Set File Position(refnum=w885, from (0:start)=enum16{"start", "end", "current"}."end", error in=w884) -> (refnum out=w887:refnum<file>, error out=w888:errorcluster)  [unwired: 1 in]
                                n1097 = Number To Fractional String(number=w875, precision (6)=i16 2) -> (F-format string=w874:string)  [unwired: 2 in]
                                n1098 = Add(x=w875, y=0.2) -> (x+y=w881:dbl)
                                n1099 = feedback-in #4(w881) -> ()
                                n1100 = Concatenate Strings(w874, w871, w877, w871, w876, w871) -> (w873:string)
                                n1101 = Write to Text File(file (use dialog)=w887, text=w873, error in=w888) -> (refnum out=w883:refnum<file>, error out=w882:errorcluster)  [unwired: 1 in, 1 out]
                                n1102 = Close File(refnum=w883, error in=w882) -> (error out=w890:errorcluster)  [unwired: 1 out]
                                n1103 = call <vilib>:"Simple Error Handler.vi"("error in (no error)"=w890) -> ()  [unwired: 1 in, 8 out]
                              }
                              frame #1 {
                                n1104 = case shown="False" "C50L" {
                                tunnel: w896 -> [_ w923]
                                tunnel: [0.0 ("MEASURE A") w903] -> w895
                                tunnel: w894 -> [_ w902]
                                tunnel: w893 -> [_ w898]
                                frame False {
                                }
                                frame True {
                                w904 = "\t"
                                w922 = i16 4 ("width (-)")
                                n1105 = Open/Create/Replace File(file path (use dialog)=w898, operation (0:open)=T3."open") -> (refnum out=w913:refnum<file>, error out=w912:errorcluster)  [unwired: 2 in, 3 out]
                                n1106 = Multiply(x="Time RLC", y=u32 1000) -> (x*y=w901:u32)
                                n1107 = Wait (ms)(milliseconds to wait=w901) -> ()  [unwired: 1 out]
                                n1108 = Set File Position(refnum=w913, from (0:start)=enum16{"start", "end", "current"}."end", error in=w912) -> (refnum out=w915:refnum<file>, error out=w916:errorcluster)  [unwired: 1 in]
                                n1109 = call "RLC_read.vi"("Path"=w902, "String"="cmd /c rlc_read_cAL.py") -> ("MEASURE A"=w903:dbl, "MEASURE V [V]"=w920:dbl, "concatenated string"=w924:string, "MEASURE B"=w921:dbl, "MEASURE I [A]"=w919:dbl)  [unwired: 1 out]
                                "MEASURE A" <- w903
                                "MEASURE B" <- w921
                                n1110 = Number To Engineering String(2:w922, 4:w919) -> (0:w905:string)  [unwired: 2 in]
                                n1111 = local write "RLC300 - digimess"(w924) -> ()
                                n1112 = Number To Engineering String(2:w922, 4:w920) -> (0:w906:string)  [unwired: 2 in]
                                n1113 = Number To Engineering String(2:w922, 4:w903) -> (0:w908:string)  [unwired: 2 in]
                                n1114 = Number To Engineering String(2:w922, 4:w921) -> (0:w907:string)  [unwired: 2 in]
                                n1115 = Concatenate Strings(w908, w904, w907, w904, w906, w904, w905, w904) -> (w909:string)
                                n1116 = Write to Text File(file (use dialog)=w915, text=w909, error in=w916) -> (refnum out=w911:refnum<file>, error out=w910:errorcluster)  [unwired: 1 in, 1 out]
                                n1117 = Close File(refnum=w911, error in=w910) -> (error out=w918:errorcluster)  [unwired: 1 out]
                                n1118 = call <vilib>:"Simple Error Handler.vi"("error in (no error)"=w918) -> ()  [unwired: 1 in, 8 out]
                                "C-50-L" <- w923
                                }
                                }
                              }
                              frame #2 {
                                n1119 = case shown="False" "C50N" {
                                tunnel: w930 -> [_ w955]
                                tunnel: [0.0 ("MEASURE A") w935] -> w929
                                tunnel: w928 -> [_ w934]
                                tunnel: w927 -> [_ w932]
                                frame False {
                                }
                                frame True {
                                w939 = "\t"
                                w954 = i16 4 ("width (-)")
                                n1120 = property on="Time RLC" class="DigNum (strict)"() -> ("Value"=w933:u32)  [unwired: 2 in, 2 out]
                                n1121 = Wait (ms)(milliseconds to wait=w933) -> ()  [unwired: 1 out]
                                n1122 = Open/Create/Replace File(file path (use dialog)=w932, operation (0:open)=T3."open") -> (refnum out=w948:refnum<file>, error out=w947:errorcluster)  [unwired: 2 in, 3 out]
                                n1123 = Set File Position(refnum=w948, from (0:start)=enum16{"start", "end", "current"}."end", error in=w947) -> (refnum out=w950:refnum<file>, error out=w951:errorcluster)  [unwired: 1 in]
                                n1124 = call "RLC_read.vi"("Path"=w934, "String"="cmd /c rlc_read_cAN.py") -> ("MEASURE A"=w935:dbl, "MEASURE V [V]"=w937:dbl, "concatenated string"=w957:string, "MEASURE B"=w938:dbl, "MEASURE I [A]"=w936:dbl)  [unwired: 1 out]
                                "MEASURE A 2" <- w935
                                "MEASURE B 2" <- w938
                                n1125 = Number To Engineering String(2:w954, 4:w936) -> (0:w940:string)  [unwired: 2 in]
                                n1126 = local write "RLC300 - digimess"(w957) -> ()
                                n1127 = Number To Engineering String(2:w954, 4:w937) -> (0:w941:string)  [unwired: 2 in]
                                n1128 = Number To Engineering String(2:w954, 4:w935) -> (0:w943:string)  [unwired: 2 in]
                                n1129 = Number To Engineering String(2:w954, 4:w938) -> (0:w942:string)  [unwired: 2 in]
                                n1130 = Concatenate Strings(w943, w939, w942, w939, w941, w939, w940, w939) -> (w944:string)
                                n1131 = Write to Text File(file (use dialog)=w950, text=w944, error in=w951) -> (refnum out=w946:refnum<file>, error out=w945:errorcluster)  [unwired: 1 in, 1 out]
                                n1132 = Close File(refnum=w946, error in=w945) -> (error out=w953:errorcluster)  [unwired: 1 out]
                                n1133 = call <vilib>:"Simple Error Handler.vi"("error in (no error)"=w953) -> ()  [unwired: 1 in, 8 out]
                                "C-50-N" <- w955
                                }
                                }
                              }
                              frame #3 {
                                n1134 = case shown="False" "C100L" {
                                tunnel: w962 -> [_ w988]
                                tunnel: [0.0 ("MEASURE A") w967] -> w961
                                tunnel: w960 -> [_ w966]
                                tunnel: w959 -> [_ w964]
                                frame False {
                                }
                                frame True {
                                w971 = "\t"
                                w986 = i16 4 ("width (-)")
                                n1135 = property on="Time RLC" class="DigNum (strict)"() -> ("Value"=w965:u32)  [unwired: 2 in, 2 out]
                                n1136 = Wait (ms)(milliseconds to wait=w965) -> ()  [unwired: 1 out]
                                n1137 = Open/Create/Replace File(file path (use dialog)=w964, operation (0:open)=T3."open") -> (refnum out=w980:refnum<file>, error out=w979:errorcluster)  [unwired: 2 in, 3 out]
                                n1138 = Set File Position(refnum=w980, from (0:start)=enum16{"start", "end", "current"}."end", error in=w979) -> (refnum out=w982:refnum<file>, error out=w983:errorcluster)  [unwired: 1 in]
                                n1139 = call "RLC_read.vi"("Path"=w966, "String"="cmd /c rlc_read_cBL.py") -> ("MEASURE A"=w967:dbl, "MEASURE V [V]"=w969:dbl, "concatenated string"=w989:string, "MEASURE B"=w970:dbl, "MEASURE I [A]"=w968:dbl)  [unwired: 1 out]
                                "MEASURE A 3" <- w967
                                "MEASURE B 3" <- w970
                                n1140 = Number To Engineering String(2:w986, 4:w968) -> (0:w972:string)  [unwired: 2 in]
                                n1141 = local write "RLC300 - digimess"(w989) -> ()
                                n1142 = Number To Engineering String(2:w986, 4:w969) -> (0:w973:string)  [unwired: 2 in]
                                n1143 = Number To Engineering String(2:w986, 4:w967) -> (0:w975:string)  [unwired: 2 in]
                                n1144 = Number To Engineering String(2:w986, 4:w970) -> (0:w974:string)  [unwired: 2 in]
                                n1145 = Concatenate Strings(w975, w971, w974, w971, w973, w971, w972, w971) -> (w976:string)
                                n1146 = Write to Text File(file (use dialog)=w982, text=w976, error in=w983) -> (refnum out=w978:refnum<file>, error out=w977:errorcluster)  [unwired: 1 in, 1 out]
                                n1147 = Close File(refnum=w978, error in=w977) -> (error out=w985:errorcluster)  [unwired: 1 out]
                                n1148 = call <vilib>:"Simple Error Handler.vi"("error in (no error)"=w985) -> ()  [unwired: 1 in, 8 out]
                                "C-100-L" <- w988
                                }
                                }
                              }
                              frame #4 {
                                n1149 = case shown="False" "C100N" {
                                tunnel: w994 -> [_ w1019]
                                tunnel: [0.0 ("MEASURE A") w999] -> w993
                                tunnel: w992 -> [_ w998]
                                tunnel: w991 -> [_ w996]
                                frame False {
                                }
                                frame True {
                                w1003 = "\t"
                                w1018 = i16 4 ("width (-)")
                                n1150 = property on="Time RLC" class="DigNum (strict)"() -> ("Value"=w997:u32)  [unwired: 2 in, 2 out]
                                n1151 = Wait (ms)(milliseconds to wait=w997) -> ()  [unwired: 1 out]
                                n1152 = Open/Create/Replace File(file path (use dialog)=w996, operation (0:open)=T3."open") -> (refnum out=w1012:refnum<file>, error out=w1011:errorcluster)  [unwired: 2 in, 3 out]
                                n1153 = Set File Position(refnum=w1012, from (0:start)=enum16{"start", "end", "current"}."end", error in=w1011) -> (refnum out=w1014:refnum<file>, error out=w1015:errorcluster)  [unwired: 1 in]
                                n1154 = call "RLC_read.vi"("Path"=w998, "String"="cmd /c rlc_read_cBN.py") -> ("MEASURE A"=w999:dbl, "MEASURE V [V]"=w1001:dbl, "concatenated string"=w1021:string, "MEASURE B"=w1002:dbl, "MEASURE I [A]"=w1000:dbl)  [unwired: 1 out]
                                "MEASURE A 4" <- w999
                                "MEASURE B 4" <- w1002
                                n1155 = Number To Engineering String(2:w1018, 4:w1000) -> (0:w1004:string)  [unwired: 2 in]
                                n1156 = local write "RLC300 - digimess"(w1021) -> ()
                                n1157 = Number To Engineering String(2:w1018, 4:w1001) -> (0:w1005:string)  [unwired: 2 in]
                                n1158 = Number To Engineering String(2:w1018, 4:w999) -> (0:w1007:string)  [unwired: 2 in]
                                n1159 = Number To Engineering String(2:w1018, 4:w1002) -> (0:w1006:string)  [unwired: 2 in]
                                n1160 = Concatenate Strings(w1007, w1003, w1006, w1003, w1005, w1003, w1004, w1003) -> (w1008:string)
                                n1161 = Write to Text File(file (use dialog)=w1014, text=w1008, error in=w1015) -> (refnum out=w1010:refnum<file>, error out=w1009:errorcluster)  [unwired: 1 in, 1 out]
                                n1162 = Close File(refnum=w1010, error in=w1009) -> (error out=w1017:errorcluster)  [unwired: 1 out]
                                n1163 = call <vilib>:"Simple Error Handler.vi"("error in (no error)"=w1017) -> ()  [unwired: 1 in, 8 out]
                                "C-100-N" <- w1019
                                }
                                }
                              }
                              frame #5 {
                                n1164 = case shown="False" "C1KL" {
                                tunnel: w1026 -> [_ w1052]
                                tunnel: [0.0 ("MEASURE A") w1031] -> w1025
                                tunnel: w1024 -> [_ w1030]
                                tunnel: w1023 -> [_ w1028]
                                frame False {
                                }
                                frame True {
                                w1050 = "\t"
                                w1035 = i16 4 ("width (-)")
                                n1165 = property on="Time RLC" class="DigNum (strict)"() -> ("Value"=w1029:u32)  [unwired: 2 in, 2 out]
                                n1166 = Wait (ms)(milliseconds to wait=w1029) -> ()  [unwired: 1 out]
                                n1167 = Open/Create/Replace File(file path (use dialog)=w1028, operation (0:open)=T3."open") -> (refnum out=w1041:refnum<file>, error out=w1042:errorcluster)  [unwired: 2 in, 3 out]
                                n1168 = Set File Position(refnum=w1041, from (0:start)=enum16{"start", "end", "current"}."end", error in=w1042) -> (refnum out=w1039:refnum<file>, error out=w1038:errorcluster)  [unwired: 1 in]
                                n1169 = call "RLC_read.vi"("Path"=w1030, "String"="cmd /c rlc_read_cCL.py") -> ("MEASURE A"=w1031:dbl, "MEASURE V [V]"=w1033:dbl, "concatenated string"=w1053:string, "MEASURE B"=w1034:dbl, "MEASURE I [A]"=w1032:dbl)  [unwired: 1 out]
                                "MEASURE A 5" <- w1031
                                "MEASURE B 5" <- w1034
                                n1170 = Number To Engineering String(2:w1035, 4:w1032) -> (0:w1049:string)  [unwired: 2 in]
                                n1171 = local write "RLC300 - digimess"(w1053) -> ()
                                n1172 = Number To Engineering String(2:w1035, 4:w1033) -> (0:w1048:string)  [unwired: 2 in]
                                n1173 = Number To Engineering String(2:w1035, 4:w1031) -> (0:w1046:string)  [unwired: 2 in]
                                n1174 = Number To Engineering String(2:w1035, 4:w1034) -> (0:w1047:string)  [unwired: 2 in]
                                n1175 = Concatenate Strings(w1046, w1050, w1047, w1050, w1048, w1050, w1049, w1050) -> (w1045:string)
                                n1176 = Write to Text File(file (use dialog)=w1039, text=w1045, error in=w1038) -> (refnum out=w1043:refnum<file>, error out=w1044:errorcluster)  [unwired: 1 in, 1 out]
                                n1177 = Close File(refnum=w1043, error in=w1044) -> (error out=w1036:errorcluster)  [unwired: 1 out]
                                n1178 = call <vilib>:"Simple Error Handler.vi"("error in (no error)"=w1036) -> ()  [unwired: 1 in, 8 out]
                                "C-1K-L" <- w1052
                                }
                                }
                              }
                              frame #6 {
                                n1179 = case shown="True" "C1KN" {
                                tunnel: w1059 -> [_ w1084]
                                tunnel: [w1060 w1065] -> w1058
                                tunnel: w1057 -> [_ w1064]
                                tunnel: w1056 -> [_ w1062]
                                tunnel: [w1060 w1061] -> w1054
                                frame False {
                                w1060 = 0.0 ("MEASURE A")
                                }
                                frame True {
                                w1083 = "\t"
                                w1068 = i16 6 ("width (-)")
                                n1180 = property on="Time RLC" class="DigNum (strict)"() -> ("Value"=w1063:u32)  [unwired: 2 in, 2 out]
                                n1181 = Wait (ms)(milliseconds to wait=w1063) -> ()  [unwired: 1 out]
                                n1182 = Open/Create/Replace File(file path (use dialog)=w1062, operation (0:open)=T3."open") -> (refnum out=w1074:refnum<file>, error out=w1075:errorcluster)  [unwired: 2 in, 3 out]
                                n1183 = Set File Position(refnum=w1074, from (0:start)=enum16{"start", "end", "current"}."end", error in=w1075) -> (refnum out=w1072:refnum<file>, error out=w1071:errorcluster)  [unwired: 1 in]
                                n1184 = call "RLC_read.vi"("Path"=w1064, "String"="cmd /c rlc_read_cCN.py") -> ("MEASURE A"=w1065:dbl, "MEASURE V [V]"=w1067:dbl, "concatenated string"=w1086:string, "MEASURE B"=w1061:dbl, "MEASURE I [A]"=w1066:dbl)  [unwired: 1 out]
                                "MEASURE A 6" <- w1065
                                "MEASURE B 6" <- w1061
                                n1185 = Number To Engineering String(2:w1068, 4:w1066) -> (0:w1082:string)  [unwired: 2 in]
                                n1186 = local write "RLC300 - digimess"(w1086) -> ()
                                n1187 = Number To Engineering String(2:w1068, 4:w1067) -> (0:w1081:string)  [unwired: 2 in]
                                n1188 = Number To Engineering String(2:w1068, 4:w1065) -> (0:w1079:string)  [unwired: 2 in]
                                n1189 = Number To Engineering String(2:w1068, 4:w1061) -> (0:w1080:string)  [unwired: 2 in]
                                n1190 = Concatenate Strings(w1079, w1083, w1080, w1083, w1081, w1083, w1082, w1083) -> (w1078:string)
                                n1191 = Write to Text File(file (use dialog)=w1072, text=w1078, error in=w1071) -> (refnum out=w1076:refnum<file>, error out=w1077:errorcluster)  [unwired: 1 in, 1 out]
                                n1192 = Close File(refnum=w1076, error in=w1077) -> (error out=w1069:errorcluster)  [unwired: 1 out]
                                n1193 = call <vilib>:"Simple Error Handler.vi"("error in (no error)"=w1069) -> ()  [unwired: 1 in, 8 out]
                                "C-1K-N" <- w1084
                                }
                                }
                              }
                              frame #7 {
                                n1194 = case shown="True" "C10KL" {
                                tunnel: w1091 -> [_ w1117]
                                tunnel: [0.0 ("MEASURE A") w1096] -> w1090
                                tunnel: w1089 -> [_ w1095]
                                tunnel: w1088 -> [_ w1093]
                                frame False {
                                }
                                frame True {
                                w1100 = "\t"
                                w1115 = i16 4 ("width (-)")
                                n1195 = property on="Time RLC" class="DigNum (strict)"() -> ("Value"=w1094:u32)  [unwired: 2 in, 2 out]
                                n1196 = Wait (ms)(milliseconds to wait=w1094) -> ()  [unwired: 1 out]
                                n1197 = Open/Create/Replace File(file path (use dialog)=w1093, operation (0:open)=T3."open") -> (refnum out=w1109:refnum<file>, error out=w1108:errorcluster)  [unwired: 2 in, 3 out]
                                n1198 = Set File Position(refnum=w1109, from (0:start)=enum16{"start", "end", "current"}."end", error in=w1108) -> (refnum out=w1111:refnum<file>, error out=w1112:errorcluster)  [unwired: 1 in]
                                n1199 = call "RLC_read.vi"("Path"=w1095, "String"="cmd /c rlc_read_cDL.py") -> ("MEASURE A"=w1096:dbl, "MEASURE V [V]"=w1098:dbl, "concatenated string"=w1118:string, "MEASURE B"=w1099:dbl, "MEASURE I [A]"=w1097:dbl)  [unwired: 1 out]
                                "MEASURE A 7" <- w1096
                                "MEASURE B 7" <- w1099
                                n1200 = Number To Engineering String(2:w1115, 4:w1097) -> (0:w1101:string)  [unwired: 2 in]
                                n1201 = local write "RLC300 - digimess"(w1118) -> ()
                                n1202 = Number To Engineering String(2:w1115, 4:w1098) -> (0:w1102:string)  [unwired: 2 in]
                                n1203 = Number To Engineering String(2:w1115, 4:w1096) -> (0:w1104:string)  [unwired: 2 in]
                                n1204 = Number To Engineering String(2:w1115, 4:w1099) -> (0:w1103:string)  [unwired: 2 in]
                                n1205 = Concatenate Strings(w1104, w1100, w1103, w1100, w1102, w1100, w1101, w1100) -> (w1105:string)
                                n1206 = Write to Text File(file (use dialog)=w1111, text=w1105, error in=w1112) -> (refnum out=w1107:refnum<file>, error out=w1106:errorcluster)  [unwired: 1 in, 1 out]
                                n1207 = Close File(refnum=w1107, error in=w1106) -> (error out=w1114:errorcluster)  [unwired: 1 out]
                                n1208 = call <vilib>:"Simple Error Handler.vi"("error in (no error)"=w1114) -> ()  [unwired: 1 in, 8 out]
                                "C-10K-L" <- w1117
                                }
                                }
                              }
                              frame #8 {
                                n1209 = case shown="False" "C10KN" {
                                tunnel: w1123 -> [_ w1149]
                                tunnel: [0.0 ("MEASURE A") w1128] -> w1122
                                tunnel: w1121 -> [_ w1127]
                                tunnel: w1120 -> [_ w1125]
                                frame False {
                                }
                                frame True {
                                w1132 = "\t"
                                w1147 = i16 4 ("width (-)")
                                n1210 = property on="Time RLC" class="DigNum (strict)"() -> ("Value"=w1126:u32)  [unwired: 2 in, 2 out]
                                n1211 = Wait (ms)(milliseconds to wait=w1126) -> ()  [unwired: 1 out]
                                n1212 = Open/Create/Replace File(file path (use dialog)=w1125, operation (0:open)=T3."open") -> (refnum out=w1141:refnum<file>, error out=w1140:errorcluster)  [unwired: 2 in, 3 out]
                                n1213 = Set File Position(refnum=w1141, from (0:start)=enum16{"start", "end", "current"}."end", error in=w1140) -> (refnum out=w1143:refnum<file>, error out=w1144:errorcluster)  [unwired: 1 in]
                                n1214 = call "RLC_read.vi"("Path"=w1127, "String"="cmd /c rlc_read_cDN.py") -> ("MEASURE A"=w1128:dbl, "MEASURE V [V]"=w1130:dbl, "concatenated string"=w1150:string, "MEASURE B"=w1131:dbl, "MEASURE I [A]"=w1129:dbl)  [unwired: 1 out]
                                "MEASURE A 8" <- w1128
                                "MEASURE B 8" <- w1131
                                n1215 = Number To Engineering String(2:w1147, 4:w1129) -> (0:w1133:string)  [unwired: 2 in]
                                n1216 = local write "RLC300 - digimess"(w1150) -> ()
                                n1217 = Number To Engineering String(2:w1147, 4:w1130) -> (0:w1134:string)  [unwired: 2 in]
                                n1218 = Number To Engineering String(2:w1147, 4:w1128) -> (0:w1136:string)  [unwired: 2 in]
                                n1219 = Number To Engineering String(2:w1147, 4:w1131) -> (0:w1135:string)  [unwired: 2 in]
                                n1220 = Concatenate Strings(w1136, w1132, w1135, w1132, w1134, w1132, w1133, w1132) -> (w1137:string)
                                n1221 = Write to Text File(file (use dialog)=w1143, text=w1137, error in=w1144) -> (refnum out=w1139:refnum<file>, error out=w1138:errorcluster)  [unwired: 1 in, 1 out]
                                n1222 = Close File(refnum=w1139, error in=w1138) -> (error out=w1146:errorcluster)  [unwired: 1 out]
                                n1223 = call <vilib>:"Simple Error Handler.vi"("error in (no error)"=w1146) -> ()  [unwired: 1 in, 8 out]
                                "C-10K-N" <- w1149
                                }
                                }
                              }
                              frame #9 {
                                n1224 = case shown="False" "Z50L" {
                                tunnel: w1155 -> [_ w1180]
                                tunnel: [0.0 ("MEASURE A") w1160] -> w1154
                                tunnel: w1153 -> [_ w1159]
                                tunnel: w1152 -> [_ w1157]
                                frame False {
                                }
                                frame True {
                                w1164 = "\t"
                                w1179 = i16 4 ("width (-)")
                                n1225 = property on="Time RLC" class="DigNum (strict)"() -> ("Value"=w1158:u32)  [unwired: 2 in, 2 out]
                                n1226 = Wait (ms)(milliseconds to wait=w1158) -> ()  [unwired: 1 out]
                                n1227 = Open/Create/Replace File(file path (use dialog)=w1157, operation (0:open)=T3."open") -> (refnum out=w1173:refnum<file>, error out=w1172:errorcluster)  [unwired: 2 in, 3 out]
                                n1228 = Set File Position(refnum=w1173, from (0:start)=enum16{"start", "end", "current"}."end", error in=w1172) -> (refnum out=w1175:refnum<file>, error out=w1176:errorcluster)  [unwired: 1 in]
                                n1229 = call "RLC_read.vi"("Path"=w1159, "String"="cmd /c rlc_read_ZAL.py") -> ("MEASURE A"=w1160:dbl, "MEASURE V [V]"=w1162:dbl, "concatenated string"=w1181:string, "MEASURE B"=w1163:dbl, "MEASURE I [A]"=w1161:dbl)  [unwired: 1 out]
                                "MEASURE A 9" <- w1160
                                "MEASURE B 9" <- w1163
                                n1230 = Number To Engineering String(2:w1179, 4:w1161) -> (0:w1165:string)  [unwired: 2 in]
                                n1231 = local write "RLC300 - digimess"(w1181) -> ()
                                n1232 = Number To Engineering String(2:w1179, 4:w1162) -> (0:w1166:string)  [unwired: 2 in]
                                n1233 = Number To Engineering String(2:w1179, 4:w1160) -> (0:w1168:string)  [unwired: 2 in]
                                n1234 = Number To Engineering String(2:w1179, 4:w1163) -> (0:w1167:string)  [unwired: 2 in]
                                n1235 = Concatenate Strings(w1168, w1164, w1167, w1164, w1166, w1164, w1165, w1164) -> (w1169:string)
                                n1236 = Write to Text File(file (use dialog)=w1175, text=w1169, error in=w1176) -> (refnum out=w1171:refnum<file>, error out=w1170:errorcluster)  [unwired: 1 in, 1 out]
                                n1237 = Close File(refnum=w1171, error in=w1170) -> (error out=w1178:errorcluster)  [unwired: 1 out]
                                n1238 = call <vilib>:"Simple Error Handler.vi"("error in (no error)"=w1178) -> ()  [unwired: 1 in, 8 out]
                                "Z-50-L" <- w1180
                                }
                                }
                              }
                              frame #10 {
                                n1239 = case shown="False" "Z50N" {
                                tunnel: w1187 -> [_ w1212]
                                tunnel: [0.0 ("MEASURE A") w1192] -> w1186
                                tunnel: w1185 -> [_ w1191]
                                tunnel: w1184 -> [_ w1189]
                                frame False {
                                }
                                frame True {
                                w1196 = "\t"
                                w1211 = i16 4 ("width (-)")
                                n1240 = property on="Time RLC" class="DigNum (strict)"() -> ("Value"=w1190:u32)  [unwired: 2 in, 2 out]
                                n1241 = Wait (ms)(milliseconds to wait=w1190) -> ()  [unwired: 1 out]
                                n1242 = Open/Create/Replace File(file path (use dialog)=w1189, operation (0:open)=T3."open") -> (refnum out=w1205:refnum<file>, error out=w1204:errorcluster)  [unwired: 2 in, 3 out]
                                n1243 = Set File Position(refnum=w1205, from (0:start)=enum16{"start", "end", "current"}."end", error in=w1204) -> (refnum out=w1207:refnum<file>, error out=w1208:errorcluster)  [unwired: 1 in]
                                n1244 = call "RLC_read.vi"("Path"=w1191, "String"="cmd /c rlc_read_ZAN.py") -> ("MEASURE A"=w1192:dbl, "MEASURE V [V]"=w1194:dbl, "concatenated string"=w1213:string, "MEASURE B"=w1195:dbl, "MEASURE I [A]"=w1193:dbl)  [unwired: 1 out]
                                "MEASURE A 10" <- w1192
                                "MEASURE B 10" <- w1195
                                n1245 = Number To Engineering String(2:w1211, 4:w1193) -> (0:w1197:string)  [unwired: 2 in]
                                n1246 = local write "RLC300 - digimess"(w1213) -> ()
                                n1247 = Number To Engineering String(2:w1211, 4:w1194) -> (0:w1198:string)  [unwired: 2 in]
                                n1248 = Number To Engineering String(2:w1211, 4:w1192) -> (0:w1200:string)  [unwired: 2 in]
                                n1249 = Number To Engineering String(2:w1211, 4:w1195) -> (0:w1199:string)  [unwired: 2 in]
                                n1250 = Concatenate Strings(w1200, w1196, w1199, w1196, w1198, w1196, w1197, w1196) -> (w1201:string)
                                n1251 = Write to Text File(file (use dialog)=w1207, text=w1201, error in=w1208) -> (refnum out=w1203:refnum<file>, error out=w1202:errorcluster)  [unwired: 1 in, 1 out]
                                n1252 = Close File(refnum=w1203, error in=w1202) -> (error out=w1210:errorcluster)  [unwired: 1 out]
                                n1253 = call <vilib>:"Simple Error Handler.vi"("error in (no error)"=w1210) -> ()  [unwired: 1 in, 8 out]
                                "Z-50-N" <- w1212
                                }
                                }
                              }
                              frame #11 {
                                n1254 = case shown="False" "Z100L" {
                                tunnel: w1219 -> [_ w1244]
                                tunnel: [0.0 ("MEASURE A") w1224] -> w1218
                                tunnel: w1217 -> [_ w1223]
                                tunnel: w1216 -> [_ w1221]
                                frame False {
                                }
                                frame True {
                                w1228 = "\t"
                                w1243 = i16 4 ("width (-)")
                                n1255 = property on="Time RLC" class="DigNum (strict)"() -> ("Value"=w1222:u32)  [unwired: 2 in, 2 out]
                                n1256 = Wait (ms)(milliseconds to wait=w1222) -> ()  [unwired: 1 out]
                                n1257 = Open/Create/Replace File(file path (use dialog)=w1221, operation (0:open)=T3."open") -> (refnum out=w1237:refnum<file>, error out=w1236:errorcluster)  [unwired: 2 in, 3 out]
                                n1258 = Set File Position(refnum=w1237, from (0:start)=enum16{"start", "end", "current"}."end", error in=w1236) -> (refnum out=w1239:refnum<file>, error out=w1240:errorcluster)  [unwired: 1 in]
                                n1259 = call "RLC_read.vi"("Path"=w1223, "String"="cmd /c rlc_read_ZBL.py") -> ("MEASURE A"=w1224:dbl, "MEASURE V [V]"=w1226:dbl, "concatenated string"=w1245:string, "MEASURE B"=w1227:dbl, "MEASURE I [A]"=w1225:dbl)  [unwired: 1 out]
                                "MEASURE A 11" <- w1224
                                "MEASURE B 11" <- w1227
                                n1260 = Number To Engineering String(2:w1243, 4:w1225) -> (0:w1229:string)  [unwired: 2 in]
                                n1261 = local write "RLC300 - digimess"(w1245) -> ()
                                n1262 = Number To Engineering String(2:w1243, 4:w1226) -> (0:w1230:string)  [unwired: 2 in]
                                n1263 = Number To Engineering String(2:w1243, 4:w1224) -> (0:w1232:string)  [unwired: 2 in]
                                n1264 = Number To Engineering String(2:w1243, 4:w1227) -> (0:w1231:string)  [unwired: 2 in]
                                n1265 = Concatenate Strings(w1232, w1228, w1231, w1228, w1230, w1228, w1229, w1228) -> (w1233:string)
                                n1266 = Write to Text File(file (use dialog)=w1239, text=w1233, error in=w1240) -> (refnum out=w1235:refnum<file>, error out=w1234:errorcluster)  [unwired: 1 in, 1 out]
                                n1267 = Close File(refnum=w1235, error in=w1234) -> (error out=w1242:errorcluster)  [unwired: 1 out]
                                n1268 = call <vilib>:"Simple Error Handler.vi"("error in (no error)"=w1242) -> ()  [unwired: 1 in, 8 out]
                                "Z-100-L" <- w1244
                                }
                                }
                              }
                              frame #12 {
                                n1269 = case shown="False" "Z100N" {
                                tunnel: w1251 -> [_ w1276]
                                tunnel: [0.0 ("MEASURE A") w1256] -> w1250
                                tunnel: w1249 -> [_ w1255]
                                tunnel: w1248 -> [_ w1253]
                                frame False {
                                }
                                frame True {
                                w1260 = "\t"
                                w1275 = i16 4 ("width (-)")
                                n1270 = property on="Time RLC" class="DigNum (strict)"() -> ("Value"=w1254:u32)  [unwired: 2 in, 2 out]
                                n1271 = Wait (ms)(milliseconds to wait=w1254) -> ()  [unwired: 1 out]
                                n1272 = Open/Create/Replace File(file path (use dialog)=w1253, operation (0:open)=T3."open") -> (refnum out=w1269:refnum<file>, error out=w1268:errorcluster)  [unwired: 2 in, 3 out]
                                n1273 = Set File Position(refnum=w1269, from (0:start)=enum16{"start", "end", "current"}."end", error in=w1268) -> (refnum out=w1271:refnum<file>, error out=w1272:errorcluster)  [unwired: 1 in]
                                n1274 = call "RLC_read.vi"("Path"=w1255, "String"="cmd /c rlc_read_ZBN.py") -> ("MEASURE A"=w1256:dbl, "MEASURE V [V]"=w1258:dbl, "concatenated string"=w1277:string, "MEASURE B"=w1259:dbl, "MEASURE I [A]"=w1257:dbl)  [unwired: 1 out]
                                "MEASURE A 12" <- w1256
                                "MEASURE B 12" <- w1259
                                n1275 = Number To Engineering String(2:w1275, 4:w1257) -> (0:w1261:string)  [unwired: 2 in]
                                n1276 = local write "RLC300 - digimess"(w1277) -> ()
                                n1277 = Number To Engineering String(2:w1275, 4:w1258) -> (0:w1262:string)  [unwired: 2 in]
                                n1278 = Number To Engineering String(2:w1275, 4:w1256) -> (0:w1264:string)  [unwired: 2 in]
                                n1279 = Number To Engineering String(2:w1275, 4:w1259) -> (0:w1263:string)  [unwired: 2 in]
                                n1280 = Concatenate Strings(w1264, w1260, w1263, w1260, w1262, w1260, w1261, w1260) -> (w1265:string)
                                n1281 = Write to Text File(file (use dialog)=w1271, text=w1265, error in=w1272) -> (refnum out=w1267:refnum<file>, error out=w1266:errorcluster)  [unwired: 1 in, 1 out]
                                n1282 = Close File(refnum=w1267, error in=w1266) -> (error out=w1274:errorcluster)  [unwired: 1 out]
                                n1283 = call <vilib>:"Simple Error Handler.vi"("error in (no error)"=w1274) -> ()  [unwired: 1 in, 8 out]
                                "Z-100-N" <- w1276
                                }
                                }
                              }
                              frame #13 {
                                n1284 = case shown="False" "Z1KL" {
                                tunnel: w1283 -> [_ w1308]
                                tunnel: [0.0 ("MEASURE A") w1288] -> w1282
                                tunnel: w1281 -> [_ w1287]
                                tunnel: w1280 -> [_ w1285]
                                frame False {
                                }
                                frame True {
                                w1292 = "\t"
                                w1307 = i16 4 ("width (-)")
                                n1285 = property on="Time RLC" class="DigNum (strict)"() -> ("Value"=w1286:u32)  [unwired: 2 in, 2 out]
                                n1286 = Wait (ms)(milliseconds to wait=w1286) -> ()  [unwired: 1 out]
                                n1287 = Open/Create/Replace File(file path (use dialog)=w1285, operation (0:open)=T3."open") -> (refnum out=w1301:refnum<file>, error out=w1300:errorcluster)  [unwired: 2 in, 3 out]
                                n1288 = Set File Position(refnum=w1301, from (0:start)=enum16{"start", "end", "current"}."end", error in=w1300) -> (refnum out=w1303:refnum<file>, error out=w1304:errorcluster)  [unwired: 1 in]
                                n1289 = call "RLC_read.vi"("Path"=w1287, "String"="cmd /c rlc_read_ZCL.py") -> ("MEASURE A"=w1288:dbl, "MEASURE V [V]"=w1290:dbl, "concatenated string"=w1309:string, "MEASURE B"=w1291:dbl, "MEASURE I [A]"=w1289:dbl)  [unwired: 1 out]
                                "MEASURE A 13" <- w1288
                                "MEASURE B 13" <- w1291
                                n1290 = Number To Engineering String(2:w1307, 4:w1289) -> (0:w1293:string)  [unwired: 2 in]
                                n1291 = local write "RLC300 - digimess"(w1309) -> ()
                                n1292 = Number To Engineering String(2:w1307, 4:w1290) -> (0:w1294:string)  [unwired: 2 in]
                                n1293 = Number To Engineering String(2:w1307, 4:w1288) -> (0:w1296:string)  [unwired: 2 in]
                                n1294 = Number To Engineering String(2:w1307, 4:w1291) -> (0:w1295:string)  [unwired: 2 in]
                                n1295 = Concatenate Strings(w1296, w1292, w1295, w1292, w1294, w1292, w1293, w1292) -> (w1297:string)
                                n1296 = Write to Text File(file (use dialog)=w1303, text=w1297, error in=w1304) -> (refnum out=w1299:refnum<file>, error out=w1298:errorcluster)  [unwired: 1 in, 1 out]
                                n1297 = Close File(refnum=w1299, error in=w1298) -> (error out=w1306:errorcluster)  [unwired: 1 out]
                                n1298 = call <vilib>:"Simple Error Handler.vi"("error in (no error)"=w1306) -> ()  [unwired: 1 in, 8 out]
                                "Z-1K-L" <- w1308
                                }
                                }
                              }
                              frame #14 {
                                n1299 = case shown="True" "Z1KN" {
                                tunnel: w1316 -> [_ w1342]
                                tunnel: [0.0 ("MEASURE A") w1323] -> w1315
                                tunnel: w1314 -> [_ w1322]
                                tunnel: w1313 -> [_ w1320]
                                tunnel: [_ w1319] -> w1311
                                frame False {
                                }
                                frame True {
                                w1326 = "\t"
                                w1341 = i16 6 ("width (-)")
                                n1300 = property on="Time RLC" class="DigNum (strict)"() -> ("Value"=w1321:u32)  [unwired: 2 in, 2 out]
                                n1301 = Wait (ms)(milliseconds to wait=w1321) -> ()  [unwired: 1 out]
                                n1302 = Open/Create/Replace File(file path (use dialog)=w1320, operation (0:open)=T3."open") -> (refnum out=w1335:refnum<file>, error out=w1334:errorcluster)  [unwired: 2 in, 3 out]
                                n1303 = Set File Position(refnum=w1335, from (0:start)=enum16{"start", "end", "current"}."end", error in=w1334) -> (refnum out=w1337:refnum<file>, error out=w1338:errorcluster)  [unwired: 1 in]
                                n1304 = call "RLC_read.vi"("Path"=w1322, "String"="cmd /c rlc_read_ZCN.py") -> ("MEASURE A"=w1323:dbl, "MEASURE V [V]"=w1325:dbl, "concatenated string"=w1343:string, "MEASURE B"=w1319:dbl, "MEASURE I [A]"=w1324:dbl)  [unwired: 1 out]
                                "MEASURE A 14" <- w1323
                                "MEASURE B 14" <- w1319
                                n1305 = Number To Engineering String(2:w1341, 4:w1324) -> (0:w1327:string)  [unwired: 2 in]
                                n1306 = local write "RLC300 - digimess"(w1343) -> ()
                                n1307 = Number To Engineering String(2:w1341, 4:w1325) -> (0:w1328:string)  [unwired: 2 in]
                                n1308 = Number To Engineering String(2:w1341, 4:w1323) -> (0:w1330:string)  [unwired: 2 in]
                                n1309 = Number To Engineering String(2:w1341, 4:w1319) -> (0:w1329:string)  [unwired: 2 in]
                                n1310 = Concatenate Strings(w1330, w1326, w1329, w1326, w1328, w1326, w1327, w1326, "\r\n") -> (w1331:string)
                                n1311 = Write to Text File(file (use dialog)=w1337, text=w1331, error in=w1338) -> (refnum out=w1333:refnum<file>, error out=w1332:errorcluster)  [unwired: 1 in, 1 out]
                                n1312 = Close File(refnum=w1333, error in=w1332) -> (error out=w1340:errorcluster)  [unwired: 1 out]
                                n1313 = call <vilib>:"Simple Error Handler.vi"("error in (no error)"=w1340) -> ()  [unwired: 1 in, 8 out]
                                "Z-1K-N" <- w1342
                                }
                                }
                              }
                              frame #15 {
                                n1314 = case shown="False" "Z10KL" {
                                tunnel: w1349 -> [_ w1374]
                                tunnel: [0.0 ("MEASURE A") w1354] -> w1348
                                tunnel: w1347 -> [_ w1353]
                                tunnel: w1346 -> [_ w1351]
                                frame False {
                                }
                                frame True {
                                w1358 = "\t"
                                w1373 = i16 4 ("width (-)")
                                n1315 = property on="Time RLC" class="DigNum (strict)"() -> ("Value"=w1352:u32)  [unwired: 2 in, 2 out]
                                n1316 = Wait (ms)(milliseconds to wait=w1352) -> ()  [unwired: 1 out]
                                n1317 = Open/Create/Replace File(file path (use dialog)=w1351, operation (0:open)=T3."open") -> (refnum out=w1367:refnum<file>, error out=w1366:errorcluster)  [unwired: 2 in, 3 out]
                                n1318 = Set File Position(refnum=w1367, from (0:start)=enum16{"start", "end", "current"}."end", error in=w1366) -> (refnum out=w1369:refnum<file>, error out=w1370:errorcluster)  [unwired: 1 in]
                                n1319 = call "RLC_read.vi"("Path"=w1353, "String"="cmd /c rlc_read_ZDL.py") -> ("MEASURE A"=w1354:dbl, "MEASURE V [V]"=w1356:dbl, "concatenated string"=w1375:string, "MEASURE B"=w1357:dbl, "MEASURE I [A]"=w1355:dbl)  [unwired: 1 out]
                                "MEASURE A 15" <- w1354
                                "MEASURE B 15" <- w1357
                                n1320 = Number To Engineering String(2:w1373, 4:w1355) -> (0:w1359:string)  [unwired: 2 in]
                                n1321 = local write "RLC300 - digimess"(w1375) -> ()
                                n1322 = Number To Engineering String(2:w1373, 4:w1356) -> (0:w1360:string)  [unwired: 2 in]
                                n1323 = Number To Engineering String(2:w1373, 4:w1354) -> (0:w1362:string)  [unwired: 2 in]
                                n1324 = Number To Engineering String(2:w1373, 4:w1357) -> (0:w1361:string)  [unwired: 2 in]
                                n1325 = Concatenate Strings(w1362, w1358, w1361, w1358, w1360, w1358, w1359, w1358) -> (w1363:string)
                                n1326 = Write to Text File(file (use dialog)=w1369, text=w1363, error in=w1370) -> (refnum out=w1365:refnum<file>, error out=w1364:errorcluster)  [unwired: 1 in, 1 out]
                                n1327 = Close File(refnum=w1365, error in=w1364) -> (error out=w1372:errorcluster)  [unwired: 1 out]
                                n1328 = call <vilib>:"Simple Error Handler.vi"("error in (no error)"=w1372) -> ()  [unwired: 1 in, 8 out]
                                "Z-10K-L" <- w1374
                                }
                                }
                              }
                              frame #16 {
                                n1329 = case shown="True" "Z10KN" {
                                tunnel: w1381 -> [_ w1407]
                                tunnel: [0.0 ("MEASURE A") w1386] -> w1380
                                tunnel: w1379 -> [_ w1385]
                                tunnel: w1378 -> [_ w1383]
                                frame False {
                                }
                                frame True {
                                w1391 = "\t"
                                w1406 = i16 4 ("width (-)")
                                n1330 = property on="Time RLC" class="DigNum (strict)"() -> ("Value"=w1384:u32)  [unwired: 2 in, 2 out]
                                n1331 = Wait (ms)(milliseconds to wait=w1384) -> ()  [unwired: 1 out]
                                n1332 = Open/Create/Replace File(file path (use dialog)=w1383, operation (0:open)=T3."open") -> (refnum out=w1400:refnum<file>, error out=w1399:errorcluster)  [unwired: 2 in, 3 out]
                                n1333 = Set File Position(refnum=w1400, from (0:start)=enum16{"start", "end", "current"}."end", error in=w1399) -> (refnum out=w1402:refnum<file>, error out=w1403:errorcluster)  [unwired: 1 in]
                                n1334 = call "RLC_read.vi"("Path"=w1385, "String"="cmd /c rlc_read_ZDN.py") -> ("MEASURE A"=w1386:dbl, "MEASURE V [V]"=w1389:dbl, "concatenated string"=w1408:string, "MEASURE B"=w1390:dbl, "MEASURE I [A]"=w1388:dbl)  [unwired: 1 out]
                                "MEASURE A 16" <- w1386
                                "MEASURE B 16" <- w1390
                                n1335 = Number To Engineering String(2:w1406, 4:w1388) -> (0:w1392:string)  [unwired: 2 in]
                                n1336 = local write "RLC300 - digimess"(w1408) -> ()
                                n1337 = Number To Engineering String(2:w1406, 4:w1389) -> (0:w1393:string)  [unwired: 2 in]
                                n1338 = Number To Engineering String(2:w1406, 4:w1386) -> (0:w1395:string)  [unwired: 2 in]
                                n1339 = Number To Engineering String(2:w1406, 4:w1390) -> (0:w1394:string)  [unwired: 2 in]
                                n1340 = Concatenate Strings(w1395, w1391, w1394, w1391, w1393, w1391, w1392, w1391, "\r\n") -> (w1396:string)
                                n1341 = Write to Text File(file (use dialog)=w1402, text=w1396, error in=w1403) -> (refnum out=w1398:refnum<file>, error out=w1397:errorcluster)  [unwired: 1 in, 1 out]
                                n1342 = Close File(refnum=w1398, error in=w1397) -> (error out=w1405:errorcluster)  [unwired: 1 out]
                                n1343 = call <vilib>:"Simple Error Handler.vi"("error in (no error)"=w1405) -> ()  [unwired: 1 in, 8 out]
                                "Z-10K-N" <- w1407
                                }
                                }
                              }
                              frame #17 {
                                n1344 = local write "Z-50-L"(w1411) -> ()
                                n1345 = local write "Z-1K-L"(w1411) -> ()
                                n1346 = local write "Z-1K-N"(w1411) -> ()
                                n1347 = local write "C-50-N"(w1411) -> ()
                                n1348 = local write "C-50-L"(w1411) -> ()
                                n1349 = local write "Z-50-N"(w1411) -> ()
                                n1350 = local write "C-1K-N"(w1411) -> ()
                                n1351 = local write "C-1K-L"(w1411) -> ()
                                n1352 = local write "Z-100-L"(w1411) -> ()
                                n1353 = local write "Z-100-N"(w1411) -> ()
                                n1354 = local write "Z-10K-L"(w1411) -> ()
                                n1355 = local write "Z-10K-N"(w1411) -> ()
                                n1356 = local write "C-10K-N"(w1411) -> ()
                                n1357 = local write "C-10K-L"(w1411) -> ()
                                n1358 = local write "C-100-N"(w1411) -> ()
                                n1359 = local write "C-100-L"(w1411) -> ()
                              }
                            }
                          }
                          n1360 = call <vilib>:"Mean.vi"("X"=w842) -> ("mean"=w824:dbl)  [unwired: 1 out]
                          "mean" <- w824
                          n1361 = call <vilib>:"Mean.vi"("X"=w841) -> ("mean"=w823:dbl)  [unwired: 1 out]
                          "mean 2" <- w823
                          n1362 = call <vilib>:"Mean.vi"("X"=w840) -> ("mean"=w822:dbl)  [unwired: 1 out]
                          "mean 3" <- w822
                          n1363 = call <vilib>:"Mean.vi"("X"=w839) -> ("mean"=w821:dbl)  [unwired: 1 out]
                          "mean 4" <- w821
                          n1364 = call <vilib>:"Mean.vi"("X"=w838) -> ("mean"=w820:dbl)  [unwired: 1 out]
                          "mean 5" <- w820
                          n1365 = call <vilib>:"Mean.vi"("X"=w837) -> ("mean"=w819:dbl)  [unwired: 1 out]
                          "mean 6" <- w819
                          n1366 = call <vilib>:"Mean.vi"("X"=w836) -> ("mean"=w818:dbl)  [unwired: 1 out]
                          "mean 7" <- w818
                          n1367 = call <vilib>:"Mean.vi"("X"=w835) -> ("mean"=w817:dbl)  [unwired: 1 out]
                          "mean 8" <- w817
                          n1368 = call <vilib>:"Mean.vi"("X"=w834) -> ("mean"=w816:dbl)  [unwired: 1 out]
                          "mean 9" <- w816
                          n1369 = call <vilib>:"Mean.vi"("X"=w833) -> ("mean"=w815:dbl)  [unwired: 1 out]
                          "mean 10" <- w815
                          n1370 = call <vilib>:"Mean.vi"("X"=w832) -> ("mean"=w814:dbl)  [unwired: 1 out]
                          "mean 11" <- w814
                          n1371 = call <vilib>:"Mean.vi"("X"=w831) -> ("mean"=w813:dbl)  [unwired: 1 out]
                          "mean 12" <- w813
                          n1372 = call <vilib>:"Mean.vi"("X"=w830) -> ("mean"=w812:dbl)  [unwired: 1 out]
                          "mean 13" <- w812
                          n1373 = call <vilib>:"Mean.vi"("X"=w829) -> ("mean"=w811:dbl)  [unwired: 1 out]
                          "mean 14" <- w811
                          n1374 = call <vilib>:"Mean.vi"("X"=w828) -> ("mean"=w810:dbl)  [unwired: 1 out]
                          "mean 15" <- w810
                          n1375 = call <vilib>:"Mean.vi"("X"=w827) -> ("mean"=w809:dbl)  [unwired: 1 out]
                          "mean 16" <- w809
                          n1376 = call <vilib>:"Mean.vi"("X"=w808) -> ("mean"=w807:dbl)  [unwired: 1 out]
                          "mean 17" <- w807
                          n1377 = call <vilib>:"Mean.vi"("X"=w805) -> ("mean"=w806:dbl)  [unwired: 1 out]
                          "mean 18" <- w806
                        }
                      }
                    }
                    frame #2 {
                      n1378 = case shown="True" w1414 {
                        tunnel: w1431 -> [_ w1455]
                        tunnel: w1430 -> [_ w1454]
                        tunnel: w1429 -> [_ w1453]
                        tunnel: w1428 -> [_ w1452]
                        tunnel: w1427 -> [_ w1451]
                        tunnel: w1426 -> [_ w1450]
                        tunnel: w1425 -> [_ w1449]
                        tunnel: w1424 -> [_ w1448]
                        tunnel: w1423 -> [_ w1447]
                        tunnel: w1422 -> [_ w1446]
                        tunnel: w1421 -> [_ w1445]
                        tunnel: w1420 -> [_ w1444]
                        tunnel: w1419 -> [_ w1443]
                        tunnel: w1418 -> [_ w1442]
                        tunnel: w1417 -> [_ w1441]
                        tunnel: w1416 -> [_ w1440]
                        tunnel: w1413 -> [_ w1433]
                        tunnel: w1412 -> [_ w1432]
                        frame False {
                        }
                        frame True {
                          w1439 = "\t"
                          w1484 = i16 6 ("precision (6)")
                          n1379 = property on="SET" class="DigNum (strict)"() -> ("Value"=w1485:i32)  [unwired: 2 in, 2 out]
                          n1380 = Number To Engineering String(2:i16 6 ("precision (6)"), 4:w1433) -> (0:w1437:string)  [unwired: 2 in]
                          n1381 = Number To Engineering String(2:i16 6 ("precision (6)"), 4:w1432) -> (0:w1434:string)  [unwired: 2 in]
                          n1382 = Number To Engineering String(2:w1484, 4:w1455) -> (0:w1482:string)  [unwired: 2 in]
                          n1383 = Number To Engineering String(2:w1484, 4:w1440) -> (0:w1481:string)  [unwired: 2 in]
                          n1384 = Number To Engineering String(2:w1484, 4:w1454) -> (0:w1480:string)  [unwired: 2 in]
                          n1385 = Number To Engineering String(2:w1484, 4:w1453) -> (0:w1479:string)  [unwired: 2 in]
                          n1386 = Number To Engineering String(2:w1484, 4:w1452) -> (0:w1478:string)  [unwired: 2 in]
                          n1387 = Number To Engineering String(2:w1484, 4:w1451) -> (0:w1477:string)  [unwired: 2 in]
                          n1388 = Number To Engineering String(2:w1484, 4:w1450) -> (0:w1476:string)  [unwired: 2 in]
                          n1389 = Number To Engineering String(2:w1484, 4:w1449) -> (0:w1475:string)  [unwired: 2 in]
                          n1390 = Number To Engineering String(2:w1484, 4:w1448) -> (0:w1474:string)  [unwired: 2 in]
                          n1391 = Number To Engineering String(2:w1484, 4:w1447) -> (0:w1473:string)  [unwired: 2 in]
                          n1392 = Number To Engineering String(2:w1484, 4:w1446) -> (0:w1472:string)  [unwired: 2 in]
                          n1393 = Number To Engineering String(2:w1484, 4:w1445) -> (0:w1471:string)  [unwired: 2 in]
                          n1394 = Number To Engineering String(2:w1484, 4:w1444) -> (0:w1470:string)  [unwired: 2 in]
                          n1395 = Number To Engineering String(2:w1484, 4:w1443) -> (0:w1469:string)  [unwired: 2 in]
                          n1396 = Number To Engineering String(2:w1484, 4:w1442) -> (0:w1468:string)  [unwired: 2 in]
                          n1397 = Number To Engineering String(2:w1484, 4:w1441) -> (0:w1467:string)  [unwired: 2 in]
                          n1398 = Number To Decimal String(number=w1485) -> (decimal integer string=w1483:string)  [unwired: 1 in]
                          n1399 = property on="path RLC_mean" class="Path"() -> ("Value"=w1456:path)  [unwired: 2 in, 2 out]
                          n1400 = Open/Create/Replace File(file path (use dialog)=w1456, operation (0:open)=T3."open") -> (refnum out=w1461:refnum<file>, error out=w1460:errorcluster)  [unwired: 2 in, 3 out]
                          n1401 = Concatenate Strings(w1483, w1439, w1482, w1439, w1481, w1439, w1480, w1439, w1479, w1439, w1478, w1439, w1477, w1439, w1476, w1439, w1475, w1439, w1474, w1439, w1473, w1439, w1472, w1439, w1471, w1439, w1470, w1439, w1469, w1439, w1468, w1439, w1467, w1439, w1437, w1439, w1434, "\r\n") -> (w1457:string)
                          n1402 = Set File Position(refnum=w1461, from (0:start)=enum16{"start", "end", "current"}."end", error in=w1460) -> (refnum out=w1463:refnum<file>, error out=w1464:errorcluster)  [unwired: 1 in]
                          n1403 = Write to Text File(file (use dialog)=w1463, text=w1457, error in=w1464) -> (refnum out=w1459:refnum<file>, error out=w1458:errorcluster)  [unwired: 1 in, 1 out]
                          n1404 = Close File(refnum=w1459, error in=w1458) -> (error out=w1466:errorcluster)  [unwired: 1 out]
                          n1405 = call <vilib>:"Simple Error Handler.vi"("error in (no error)"=w1466) -> ()  [unwired: 1 in, 8 out]
                        }
                      }
                    }
                  }
                  n1406 = local write "graph RLC"(w754) -> ()
                }
                frame 9 {
                  n1407 = flat-sequence {
                    tunnel: w1537 -> [w1548]
                    tunnel: [w1548] -> w1536
                    tunnel: [w1542] -> w1535
                    tunnel: [w1541] -> w1534
                    tunnel: w1536 -> [w1573]
                    tunnel: w1535 -> [_]
                    tunnel: w1534 -> [w1570]
                    frame #0 {
                      n1408 = property on="SET" class="DigNum (strict)"() -> ("Value"=w1546:i32)  [unwired: 2 in, 2 out]
                      n1409 = Increment(x=w1546) -> (x+1=w1541:i32)
                      n1410 = property on="P_max camara" class="DigNum (strict)"() -> ("Value"=w1539:dbl)  [unwired: 2 in, 2 out]
                      n1411 = local write "SET"(w1541) -> ()
                      n1412 = property on="Camara 2" class="Slide (strict)"() -> ("Value"=w1540:dbl)  [unwired: 2 in, 2 out]
                      n1413 = case shown="False" "Boolean" {
                        selector: "Boolean" -> [w1554 w1559]
                        tunnel: [w1556 w1563] -> w1543
                        tunnel: w1541 -> [w1557 _]
                        frame False {
                          n1414 = local write "Boolean 2"(w1554) -> ()
                          n1415 = Index Array(array="Array", index=w1557) -> (element=w1556:dbl)
                          n1416 = Not(x=w1554) -> (.not. x?=→"Boolean 3":bool)
                        }
                        frame True {
                          n1417 = property on="Set P auto" class="DigNum (strict)"() -> ("Value"=w1561:dbl)  [unwired: 2 in, 2 out]
                          n1418 = Add(x="Step P", y=w1561) -> (x+y=w1563:dbl)
                          n1419 = Not(x=w1559) -> (.not. x?=w1560:bool)
                          n1420 = local write "Boolean 3"(w1560) -> ()
                          "Boolean 2" <- w1559
                        }
                      }
                      n1421 = Greater?(x=w1540, y=w1539) -> (0:w1538:bool)
                      n1422 = case shown="True" w1538 {
                        frame False {
                        }
                        frame True {
                          n1423 = property on="Desc SET" class="DigNum (strict)"() -> ("Value"=w1550:i32)  [unwired: 2 in, 2 out]
                          n1424 = local write "Descarga"(TRUE ("Descarga")) -> ()
                          n1425 = Increment(x=w1550) -> (x+1=w1549:i32)
                          n1426 = local write "Desc SET"(w1549) -> ()
                        }
                      }
                      n1427 = Greater?(x=w1543, y="P_max") -> (0:w1545:bool)
                      n1428 = case shown="True" w1545 {
                        tunnel: [w1552 w1553] -> w1542
                        tunnel: "P_max" -> [_ w1553]
                        tunnel: w1543 -> [w1552 _]
                        frame False {
                        }
                        frame True {
                        }
                      }
                      n1429 = local write "Set P auto"(w1542) -> ()
                    }
                    frame #1 {
                      n1430 = property on="Desc SET" class="DigNum (strict)"() -> ("Value"=w1565:i32)  [unwired: 2 in, 2 out]
                      n1431 = Quotient & Remainder(x=w1570, y="Step ZPit") -> (x-y*floor(x/y)=w1571:dbl)  [unwired: 1 out]
                      n1432 = Greater Than 0?(x=w1565) -> (x > 0?=w1567:bool)
                      n1433 = Equal To 0?(x=w1571) -> (x = 0?=w1569:bool)
                      "Read ZPit" <- w1569
                      n1434 = property on="Descarga" class="Bool (strict)"() -> ("Value"=w1564:bool)  [unwired: 2 in, 2 out]
                      n1435 = And(x=w1567, y=w1564) -> (x .and. y?=w1566:bool)
                      n1436 = case shown="True" w1566 {
                        tunnel: w1569 -> [w1574 _]
                        tunnel: [w1574 w1575] -> w1568
                        frame False {
                        }
                        frame True {
                          w1575 = TRUE
                          n1437 = local write "Read ZPit"(w1575) -> ()
                        }
                      }
                      n1438 = case shown="True" w1568 {
                        tunnel: w1573 -> [_ w1577]
                        frame False {
                          n1439 = local write "Estagio auto"(11 ("Estagio auto")) -> ()
                        }
                        frame True {
                          n1440 = Greater?(x=w1577, y=1.0) -> (0:w1582:bool)
                          n1441 = case shown="True" w1582 {
                            tunnel: [FALSE ("Boolean") TRUE ("Boolean")] -> w1580
                            frame False {
                              w1602 = TRUE ("Boolean")
                              n1442 = local write "Vácuo 2"(w1602) -> ()
                              n1443 = Multiply(x="ZPf2 time", y=0.0741) -> (x*y=w1597:dbl)
                              n1444 = local write "String"("Limpar volume referencia" ("String")) -> ()
                              n1445 = Add(x=w1597, y=1.9801) -> (x+y=w1595:dbl)
                              n1446 = call "Controle_vacuo.vi"("time (s) to wait vacuo"=w1595, "Boolean"=w1602) -> ("Vacuo"=w1603:bool)  [unwired: 9 in]
                              n1447 = local write "Vácuo 2"(w1603) -> ()
                            }
                            frame True {
                              n1448 = property on="ATM wait" class="DigNum (strict)"() -> ("Value"=w1604:u32)  [unwired: 2 in, 2 out]
                              n1449 = call "Controle_ATM.vi"("seconds to wait"=w1604) -> ("String 2"=w1607:string, "Atm"=w1606:bool)  [unwired: 9 in]
                              n1450 = local write "Atm 2"(w1606) -> ()
                              n1451 = local write "String"(w1607) -> ()
                            }
                          }
                          n1452 = for {
                            N: 1 -> [_]
                            tunnel: [w1584] -> w1579
                            tunnel: w1580 -> [w1584]
                            n1453 = Wait (ms)(milliseconds to wait=u32 500 ("x")) -> ()  [unwired: 1 out]
                          }
                          n1454 = case shown="True" w1579 {
                            frame False {
                              n1455 = local write "Estagio auto"(10 ("Estagio auto")) -> ()
                            }
                            frame True {
                              w1593 = TRUE ("Boolean")
                              n1456 = property on="ZPf2 time" class="DigNum (strict)"() -> ("Value"=w1587:dbl)  [unwired: 2 in, 2 out]
                              n1457 = local write "Estagio auto"(10 ("Estagio auto")) -> ()
                              n1458 = local write "Vácuo 2"(w1593) -> ()
                              n1459 = Multiply(x=w1587, y=0.0741) -> (x*y=w1589:dbl)
                              n1460 = local write "String"("Limpar volume referencia" ("String")) -> ()
                              n1461 = Add(x=w1589, y=1.9801) -> (x+y=w1586:dbl)
                              n1462 = call "Controle_vacuo.vi"("time (s) to wait vacuo"=w1586, "Boolean"=w1593) -> ("Vacuo"=w1594:bool)  [unwired: 9 in]
                              n1463 = local write "Vácuo 2"(w1594) -> ()
                            }
                          }
                        }
                      }
                    }
                  }
                }
                frame 10 {
                  n1464 = property on="Contador" class="DigNum (strict)"() -> ("Value"=w1609:i32)  [unwired: 2 in, 2 out]
                  n1465 = Increment(x=w1609) -> (x+1=w1611:i32)
                  n1466 = local write "String"("Ler ZPf2 e T" ("String")) -> ()
                  n1467 = property on="N fit 2" class="DigNum (strict)"() -> ("Value"=w1608:i32)  [unwired: 2 in, 2 out]
                  n1468 = Equal?(x=w1611, y=w1608) -> (x = y?=w1610:bool)
                  n1469 = case shown="True" w1610 {
                    frame False {
                    }
                    frame True {
                      n1470 = local write "Estagio auto"(11 ("Estagio auto")) -> ()
                    }
                  }
                }
                frame 11 {
                  n1471 = property on="Contador" class="DigNum (strict)"() -> ("Value"=w1617:i32)  [unwired: 2 in, 2 out]
                  n1472 = Increment(x=w1617) -> (x+1=w1618:i32)
                  n1473 = property on="N fit 2" class="DigNum (strict)"() -> ("Value"=w1614:i32)  [unwired: 2 in, 2 out]
                  n1474 = Equal?(x=w1618, y=w1614) -> (x = y?=w1616:bool)
                  n1475 = case shown="True" w1616 {
                    tunnel: w1619 -> [_ w1630]
                    tunnel: w1615 -> [_ w1620]
                    frame False {
                    }
                    frame True {
                      w1621 = i16 3 ("precision (6)")
                      w1624 = "\t"
                      n1476 = property on="T fit" class="DigNum (strict)"() -> ("Value"=w1626:dbl)  [unwired: 2 in, 2 out]
                      n1477 = property on="Read ZPit" class="Bool (strict)"() -> ("Value"=w1625:bool)  [unwired: 2 in, 2 out]
                      n1478 = case shown="False" w1625 {
                        tunnel: ["  ==>" w1636] -> w1629
                        tunnel: w1621 -> [_ w1635]
                        frame False {
                        }
                        frame True {
                          n1479 = property on="P fit" class="DigNum (strict)"() -> ("Value"=w1634:dbl)  [unwired: 2 in, 2 out]
                          n1480 = Number To Fractional String(number=w1634, precision (6)=w1635) -> (F-format string=w1636:string)  [unwired: 2 in]
                        }
                      }
                      n1481 = Number To Fractional String(number=w1626, precision (6)=w1621) -> (F-format string=w1628:string)  [unwired: 2 in]
                      n1482 = Number To Fractional String(number=w1620, precision (6)=w1621) -> (F-format string=w1623:string)  [unwired: 2 in]
                      n1483 = Concatenate Strings(w1629, w1624, w1628, w1624, w1623, "\r\n") -> (w1627:string)
                      n1484 = flat-sequence {
                        tunnel: [w1640] -> w1632
                        tunnel: [w1639] -> w1631
                        tunnel: w1627 -> [w1638]
                        tunnel: w1630 -> [w1637]
                        tunnel: w1632 -> [w1654]
                        tunnel: w1631 -> [w1653]
                        frame #0 {
                          n1485 = Open/Create/Replace File(file path (use dialog)=w1637, operation (0:open)=T3."open") -> (refnum out=w1646:refnum<file>, error out=w1647:errorcluster)  [unwired: 2 in, 3 out]
                          n1486 = Set File Position(refnum=w1646, from (0:start)=enum16{"start", "end", "current"}."end", error in=w1647) -> (refnum out=w1644:refnum<file>, error out=w1643:errorcluster)  [unwired: 1 in]
                          n1487 = Write to Text File(file (use dialog)=w1644, text=w1638, error in=w1643) -> (refnum out=w1648:refnum<file>, error out=w1649:errorcluster)  [unwired: 2 out]
                          n1488 = Close File(refnum=w1648, error in=w1649) -> (path=w1640:path, error out=w1641:errorcluster)
                          n1489 = call <vilib>:"Simple Error Handler.vi"("error in (no error)"=w1641) -> ("error out"=w1639:errorcluster)  [unwired: 1 in, 7 out]
                        }
                        frame #1 {
                          w1650 = TRUE ("ZPit")
                          n1490 = Wait (ms)(milliseconds to wait=u32 500) -> ()  [unwired: 1 out]
                          n1491 = local write "T 2"(w1650) -> ()
                          n1492 = local write "ZPf2 2"(w1650) -> ()
                          n1493 = Read from Text File(file (use dialog)=w1654, count=-1 ("Count  3"), error in=w1653) -> (refnum out=w1655:refnum<file>, text=w1659:string, error out=w1656:errorcluster)  [unwired: 1 in, 1 out]
                          n1494 = local write "String 3"(w1659) -> ()
                          n1495 = Close File(refnum=w1655, error in=w1656) -> (error out=w1657:errorcluster)  [unwired: 1 out]
                          n1496 = call <vilib>:"Simple Error Handler.vi"("error in (no error)"=w1657) -> ()  [unwired: 1 in, 8 out]
                          n1497 = local write "String"("abrir valvula entrada gas" ("String")) -> ()
                        }
                        frame #2 {
                          n1498 = property on="Desc SET" class="DigNum (strict)"() -> ("Value"=w1661:i32)  [unwired: 2 in, 2 out]
                          n1499 = Greater Than 0?(x=w1661) -> (x > 0?=w1660:bool)
                          n1500 = property on="Camara 2" class="Slide (strict)"() -> ("Value"=w1668:dbl)  [unwired: 2 in, 2 out]
                          n1501 = Greater?(x=w1668, y="P_max camara") -> (0:w1666:bool)
                          n1502 = property on="Carga" class="Bool (strict)"() -> ("Value"=w1665:bool)  [unwired: 2 in, 2 out]
                          n1503 = And(x=w1666, y=w1665) -> (x .and. y?=w1663:bool)
                          n1504 = case shown="False" w1660 {
                            tunnel: w1663 -> [w1669 _]
                            tunnel: [w1669 TRUE] -> w1662
                            frame False {
                            }
                            frame True {
                            }
                          }
                          n1505 = case shown="True" w1662 {
                            tunnel: [5 ("N fit") w1675] -> w1664
                            frame False {
                              n1506 = local write "Estagio auto"(0 ("Estagio auto")) -> ()
                              "Carga" <- TRUE
                              "Descarga" <- FALSE
                            }
                            frame True {
                              n1507 = local write "teste slope"(0 ("teste slope")) -> ()
                              n1508 = local write "Carga"(FALSE ("Carga")) -> ()
                              n1509 = local write "Descarga"(TRUE ("Descarga")) -> ()
                              n1510 = local write "Estagio auto"(12 ("Estagio auto")) -> ()
                              n1511 = property on="N fit 2" class="DigNum (strict)"() -> ("Value"=w1675:i32)  [unwired: 2 in, 2 out]
                            }
                          }
                          n1512 = local write "N fit"(w1664) -> ()
                        }
                      }
                    }
                  }
                }
                frame 12 {
                  w1685 = "\t"
                  n1513 = property on="SET" class="DigNum (strict)"() -> ("Value"=w1689:i32)  [unwired: 2 in, 2 out]
                  n1514 = Number To Decimal String(number=w1689) -> (decimal integer string=w1692:string)  [unwired: 1 in]
                  n1515 = Number To Fractional String(number=0.0, precision (6)=i16 3) -> (F-format string=w1686:string)  [unwired: 2 in]
                  n1516 = Concatenate Strings(w1692, w1685, w1686, w1685, w1686, w1685) -> (w1691:string)
                  n1517 = flat-sequence {
                    tunnel: w1688 -> [w1697]
                    tunnel: w1691 -> [w1698]
                    tunnel: [w1698] -> w1684
                    tunnel: [w1697] -> w1683
                    tunnel: [w1702] -> w1694
                    tunnel: [w1701] -> w1693
                    tunnel: w1684 -> [w1700]
                    tunnel: w1683 -> [w1699]
                    tunnel: [w1699] -> w1682
                    tunnel: w1694 -> [w1718]
                    tunnel: w1693 -> [w1717]
                    tunnel: w1682 -> [w1712]
                    tunnel: [w1712] -> w1681
                    tunnel: w1681 -> [w1726]
                    tunnel: [w1725] -> w1680
                    tunnel: w1680 -> [w1763]
                    frame #0 {
                      w1696 = FALSE ("ZPit 2")
                      n1518 = Wait (ms)(milliseconds to wait=u32 1000) -> ()  [unwired: 1 out]
                      n1519 = local write "ZPit 2"(w1696) -> ()
                      n1520 = local write "Pit 2"(w1696) -> ()
                      n1521 = local write "Pf2 2"(w1696) -> ()
                      n1522 = local write "ZPf2 2"(w1696) -> ()
                      n1523 = local write "T 2"(w1696) -> ()
                    }
                    frame #1 {
                      n1524 = Open/Create/Replace File(file path (use dialog)=w1699, operation (0:open)=T3."open") -> (refnum out=w1708:refnum<file>, error out=w1709:errorcluster)  [unwired: 2 in, 3 out]
                      n1525 = Set File Position(refnum=w1708, from (0:start)=enum16{"start", "end", "current"}."end", error in=w1709) -> (refnum out=w1706:refnum<file>, error out=w1705:errorcluster)  [unwired: 1 in]
                      n1526 = Write to Text File(file (use dialog)=w1706, text=w1700, error in=w1705) -> (refnum out=w1710:refnum<file>, error out=w1711:errorcluster)  [unwired: 2 out]
                      n1527 = Close File(refnum=w1710, error in=w1711) -> (path=w1702:path, error out=w1703:errorcluster)
                      n1528 = call <vilib>:"Simple Error Handler.vi"("error in (no error)"=w1703) -> ("error out"=w1701:errorcluster)  [unwired: 1 in, 7 out]
                    }
                    frame #2 {
                      w1713 = TRUE ("ZPit")
                      n1529 = local write "Estagio auto"(7 ("Estagio auto")) -> ()
                      n1530 = Wait (ms)(milliseconds to wait=u32 500) -> ()  [unwired: 1 out]
                      n1531 = local write "ZPit 2"(w1713) -> ()
                      n1532 = local write "Pit 2"(w1713) -> ()
                      n1533 = Read from Text File(file (use dialog)=w1718, count=-1 ("Count  3"), error in=w1717) -> (refnum out=w1719:refnum<file>, text=w1723:string, error out=w1720:errorcluster)  [unwired: 1 in, 1 out]
                      n1534 = local write "String 3"(w1723) -> ()
                      n1535 = Close File(refnum=w1719, error in=w1720) -> (error out=w1721:errorcluster)  [unwired: 1 out]
                      n1536 = call <vilib>:"Simple Error Handler.vi"("error in (no error)"=w1721) -> ()  [unwired: 1 in, 8 out]
                      n1537 = local write "String"("abrir valvula camara" ("String")) -> ()
                    }
                    frame #3 {
                      n1538 = property on="Camara 2" class="Slide (strict)"() -> ("Value"=w1729:dbl)  [unwired: 2 in, 2 out]
                      n1539 = Less?(x=w1729, y="P_min descarga") -> (x < y?=w1724:bool)
                      n1540 = property on="Efetuados" class="DigNum (strict)"() -> ("Value"=w1727:dbl)  [unwired: 2 in, 2 out]
                      n1541 = case shown="True" w1724 {
                        tunnel: w1727 -> [_ w1758]
                        tunnel: w1726 -> [_ w1747]
                        tunnel: [TRUE ("data") FALSE ("data")] -> w1725
                        tunnel: w1724 -> [_ w1736]
                        frame False {
                          n1542 = property on="Desc SET" class="DigNum (strict)"() -> ("Value"=w1731:i32)  [unwired: 2 in, 2 out]
                          n1543 = Increment(x=w1731) -> (x+1=→"Desc SET":i32)
                        }
                        frame True {
                          w1745 = "\r\n"
                          n1544 = Increment(x=w1758) -> (x+1=w1733:dbl)
                          "Efetuados" <- w1733
                          n1545 = local write "Estagio auto"(0 ("Estagio auto")) -> ()
                          n1546 = local write "SET"(0 ("SET")) -> ()
                          n1547 = local write "Desc SET"(0 ("Desc SET")) -> ()
                          n1548 = local write "Carga"(TRUE ("Carga")) -> ()
                          n1549 = local write "Descarga"(FALSE ("Descarga")) -> ()
                          n1550 = local write "Set P auto"(0.5 ("Set P auto")) -> ()
                          n1551 = Open/Create/Replace File(file path (use dialog)=w1747, operation (0:open)=T3."open") -> (refnum out=w1753:refnum<file>, error out=w1754:errorcluster)  [unwired: 2 in, 3 out]
                          n1552 = Less Or Equal?(x="Ciclos", y=w1733) -> (x <= y?=w1734:bool)
                          n1553 = And(x=w1736, y=w1734) -> (x .and. y?=w1737:bool)
                          n1554 = Set File Position(refnum=w1753, from (0:start)=enum16{"start", "end", "current"}."end", error in=w1754) -> (refnum out=w1751:refnum<file>, error out=w1750:errorcluster)  [unwired: 1 in]
                          n1555 = case shown="False" w1737 {
                            frame False {
                              n1556 = local write "FIM"(FALSE ("FIM")) -> ()
                            }
                            frame True {
                              w1762 = 1 ("N fit")
                              n1557 = local write "Auto Ctrl"(FALSE ("Auto Ctrl")) -> ()
                              n1558 = local write "N fit"(w1762) -> ()
                              n1559 = local write "N to fit"(w1762) -> ()
                              "FIM" <- TRUE ("stop")
                            }
                          }
                          n1560 = Concatenate Strings(w1745, ">>>>>>>>>>>>>>" ("string"), w1745, w1745) -> (w1744:string)
                          n1561 = Write to Text File(file (use dialog)=w1751, text=w1744, error in=w1750) -> (refnum out=w1755:refnum<file>, error out=w1756:errorcluster)  [unwired: 2 out]
                          n1562 = Close File(refnum=w1755, error in=w1756) -> (error out=w1748:errorcluster)  [unwired: 1 out]
                          n1563 = call <vilib>:"Simple Error Handler.vi"("error in (no error)"=w1748) -> ()  [unwired: 1 in, 8 out]
                        }
                      }
                    }
                    frame #4 {
                      w1765 = T4 3 items=["no dialog", "OK message", "continue or stop message", "OK message + warnings", "continue/stop + warnings"] ("type of dialog (OK msg:1)")
                      n1564 = local write "Câmara 2"(w1763) -> ()
                      n1565 = call-poly <vilib>:"DAQmx Create Virtual Channel.vi"("lines"=tag "Dev1/port0/line3") -> ("task out"=w1774:refnum<k21>, "error out"=w1773:errorcluster)  [unwired: 13 in]
                      n1566 = call <vilib>:"DAQmx Start Task.vi"("task/channels in"=w1774, "error in"=w1773) -> ("task out"=w1772:refnum<k21>, "error out"=w1771:errorcluster)  [unwired: 12 in]
                      n1567 = call-poly <vilib>:"DAQmx Write.vi"("task/channels in"=w1772, "data"=w1763, "error in"=w1771) -> ("task out"=w1767:refnum<k21>, "error out"=w1766:errorcluster)  [unwired: 10 in, 1 out]
                      n1568 = call <vilib>:"DAQmx Stop Task.vi"("task/channels in"=w1767, "error in"=w1766) -> ("task out"=w1769:refnum<k21>, "error out"=w1770:errorcluster)  [unwired: 12 in]
                      n1569 = call <vilib>:"DAQmx Clear Task.vi"("task in"=w1769, "error in"=w1770) -> ("error out"=w1764:errorcluster)  [unwired: 13 in]
                      n1570 = call <vilib>:"Simple Error Handler.vi"("type of dialog (OK msg:1)"=w1765, "error in (no error)"=w1764) -> ()  [unwired: 3 in, 5 out]
                    }
                  }
                }
              }
            }
          }
          n1571 = Index Array(array=w274, index=w272) -> (element=w271:dbl)
          n1572 = Index Array(array=w273, index=w272) -> (element=w270:dbl)
          n1573 = Bundle("Real 2D Array"=w277, "Best Linear Fit"=w289) -> (w288:T9)  [unwired: 1 in]
          n1574 = Bundle("Real 2D Array"=w277, "Best Polynomial Fit"=w278) -> (w275:T10)  [unwired: 1 in]
          n1575 = Bundle("Real 2D Array"=w277, "Best Polynomial Fit"=w279) -> (w276:T10)  [unwired: 1 in]
          n1576 = Build Array(w287, w288, w275) -> (→"Linear T":T11)
          n1577 = Bundle("Real 2D Array"=w277, "Best Linear Fit"=w284) -> (w285:T9)  [unwired: 1 in]
          n1578 = case shown="True" w269 {
            tunnel: w271 -> [_ w1777]
            tunnel: w270 -> [_ w1776]
            tunnel: w264 -> [_ w1775]
            frame False {
            }
            frame True {
              "P fit" <- w1777
              "T fit" <- w1776
              "P (bar/s)" <- w1775
            }
          }
          n1579 = Build Array(w286, w285, w276) -> (→"Linear P":T11)
          n1580 = property on="ON/OFF" class="Bool (strict)"() -> ("Value"=w244:bool)  [unwired: 2 in, 2 out]
          n1581 = case shown="True" w244 {
            frame False {
            }
            frame True {
              n1582 = property on="Auto Ctrl" class="Bool (strict)"() -> ("Value"=w295:bool)  [unwired: 2 in, 2 out]
              n1583 = case shown="False" w295 {
                tunnel: [w300 w304] -> w298
                tunnel: [w301 w303] -> w299
                tunnel: [w302 w305] -> w297
                frame False {
                  n1584 = property on="S#01" class="DigNum (strict)"() -> ("Value"=w302:dbl)  [unwired: 2 in, 2 out]
                  n1585 = property on="termopar K" class="DigNum (strict)"() -> ("Value"=w301:dbl)  [unwired: 2 in, 2 out]
                  n1586 = property on="T fit" class="DigNum (strict)"() -> ("Value"=w300:dbl)  [unwired: 2 in, 2 out]
                }
                frame True {
                  n1587 = property on="T fit" class="DigNum (strict)"() -> ("Value"=w304:dbl)  [unwired: 2 in, 2 out]
                  n1588 = property on="termopar K 2" class="DigNum (strict)"() -> ("Value"=w303:dbl)  [unwired: 2 in, 2 out]
                  n1589 = property on="S#1_auto" class="DigNum (strict)"() -> ("Value"=w305:dbl)  [unwired: 2 in, 2 out]
                }
              }
              n1590 = Merge Signals(w297, w298, w299) -> (w296:dynamicdata)
              n1591 = property on="Waveform Chart 2" class="WFChart (strict)"("Value"=w296) -> ()  [unwired: 2 in, 2 out]
            }
          }
          "Contador" <- w268
        }
        n1592 = local write "P subarray 2"(dbl[] [0.0, 1.0] ("subarray")) -> ()
        n1593 = local write "T subarray 3"(dbl[] [0.0, 1.0] ("subarray")) -> ()
      }
    }
    n1594 = Or(x=w43, y=w42) -> (x .or. y?=w44:bool)
    n1595 = Or(x=w44, y="Refresh Button") -> (x .or. y?=w46:bool)
    n1596 = case shown="True" w46 {
      frame False {
      }
      frame True {
        n1597 = stacked-sequence {
          frame #0 {
            n1598 = property on="Waveform Chart P 2" class="WFChart (strict)"("History Data"=dbl[][] []) -> ()  [unwired: 2 in, 2 out]
          }
          frame #1 {
            n1599 = property on="path RLC_mean" class="Path"() -> ("Value"=w80:path)  [unwired: 2 in, 2 out]
            n1600 = Open/Create/Replace File(file path (use dialog)=w80, operation (0:open)=T3."open", access (0:read/write)=enum16{"read/write", "read-only", "write-only"}."read-only") -> (refnum out=w84:refnum<file>, error out=w83:errorcluster)  [unwired: 3 in, 1 out]
            n1601 = Read from Text File(file (use dialog)=w84, error in=w83) -> (refnum out=w89:refnum<file>, text=w85:string, error out=w88:errorcluster)  [unwired: 2 in, 1 out]
            n1602 = Close File(refnum=w89, error in=w88) -> ()  [unwired: 2 out]
            n1603 = Search/Split String(string=w85, search string/char (-)="SET\tDATE\tTIME\t\tP (BAR)\tT (ºC)\tC-50-L\tC-50-N\tC-100-L\tC-100-N\tC-1K-L\tC-1K-N\tC-10K-L\tC-10K-N\tZ-50-L\tZ-50-N\tZ-100-L\tZ-100-N\tZ-1K-L\tZ-1K-N\tZ-10K-L\tZ-10K-N") -> (match + rest of string=w90:string)  [unwired: 1 in, 2 out]
            n1604 = String Subset(string=w90, offset (0)=150) -> (substring=w97:string)  [unwired: 1 in]
            n1605 = Spreadsheet String To Array(format string="%#g", spreadsheet string=w97) -> (array=w96:dbl[][])  [unwired: 2 in]
            n1606 = Transpose Matrix(1:w96) -> (0:w110:dbl[][])
            n1607 = Index Array(array=w110, index (row)=1 ("index (row) 4")) -> (element=w111:dbl[])  [unwired: 1 in]
            n1608 = Index Array(array=w110, index (row)=2 ("index (row) 5")) -> (element=w112:dbl[])  [unwired: 1 in]
            n1609 = Index Array(array=w110, index (row)=3 ("index (row) 2")) -> (element=w113:dbl[])  [unwired: 1 in]
            n1610 = Index Array(array=w110, index (row)=4 ("index (row) 3")) -> (element=w114:dbl[])  [unwired: 1 in]
            n1611 = Index Array(array=w110, index (row)=5 ("index (row) 4")) -> (element=w115:dbl[])  [unwired: 1 in]
            n1612 = Index Array(array=w110, index (row)=6 ("index (row) 5")) -> (element=w116:dbl[])  [unwired: 1 in]
            n1613 = Index Array(array=w110, index (row)=7 ("index (row) 2")) -> (element=w117:dbl[])  [unwired: 1 in]
            n1614 = Index Array(array=w110, index (row)=8 ("index (row) 3")) -> (element=w118:dbl[])  [unwired: 1 in]
            n1615 = Index Array(array=w110, index (row)=9 ("index (row) 4")) -> (element=w79:dbl[])  [unwired: 1 in]
            n1616 = Index Array(array=w110, index (row)=10 ("index (row) 5")) -> (element=w78:dbl[])  [unwired: 1 in]
            n1617 = Index Array(array=w110, index (row)=11 ("index (row) 2")) -> (element=w77:dbl[])  [unwired: 1 in]
            n1618 = Index Array(array=w110, index (row)=12 ("index (row) 3")) -> (element=w76:dbl[])  [unwired: 1 in]
            n1619 = Index Array(array=w110, index (row)=13 ("index (row) 4")) -> (element=w75:dbl[])  [unwired: 1 in]
            n1620 = Index Array(array=w110, index (row)=14 ("index (row) 5")) -> (element=w74:dbl[])  [unwired: 1 in]
            n1621 = Index Array(array=w110, index (row)=15 ("index (row) 2")) -> (element=w73:dbl[])  [unwired: 1 in]
            n1622 = Index Array(array=w110, index (row)=16 ("index (row) 3")) -> (element=w72:dbl[])  [unwired: 1 in]
            n1623 = Build Array(w111, w112, w113, w114, w115, w116, w117, w118, w79, w78, w77, w76, w75, w74, w73, w72) -> (w71:dbl[][])
            n1624 = Transpose Matrix(1:w71) -> (0:→"Waveform Chart P 2":dbl[][])
          }
        }
      }
    }
  }
  n1625 = local write "path 2_cinetica"(path "C:/H2_Painel/painel_auto/cinetica.txt" ("path")) -> ()
  n1626 = local write "path RLC_completo"(path "C:/H2_Painel/painel_auto/RLC_full.txt" ("path RLC_mean")) -> ()
  n1627 = local write "path RLC_mean"(path "C:/H2_Painel/painel_auto/RLC_mean.txt" ("path RLC_mean")) -> ()
  n1628 = local write "path"(path "C:/H2_Painel/painel_auto/Arquivo_Padrao.txt" ("path")) -> ()
  n1629 = local write "path 2"(path "C:/H2_Painel/painel_auto/Arquivo_PadraoS1.txt" ("path")) -> ()
